vi "arc - v1.vi"() -> ()   [LabVIEW 2015]
doc: "This is the interface, the one VI which loads all the others. Run this one first.\n\n(the line below ensures settings are saved)\n[Red Tweezers Save Settings]"
uses:
  Matt Fall 2018 files/Matt working/Red Tweezers Image Processing Final 1-19/subvis/line_trapping.ctl
  Matt Fall 2018 files/Matt working/Red Tweezers Image Processing Final 1-19/subvis/spot.ctl
  <vilib>/userdefined/High Color/IMAQdx.ctl
  Matt Fall 2018 files/Matt working/Red Tweezers Image Processing Final 1-19/subvis/selection_element.ctl
  <vilib>/Analysis/Matrix/Datatypes/RealMatrix.ctl
  Matt Fall 2018 files/Matt working/Red Tweezers Image Processing Final 1-19/subvis/mouse_info.ctl
  <vilib>/Analysis/baseanly.llb/Real A x B.vi
  Matt Fall 2018 files/Matt working/Red Tweezers Image Processing Final 1-19/subvis/red_tweezers_globals_INTERNAL_VOLATILE.vi
  Matt Fall 2018 files/Matt working/Red Tweezers Image Processing Final 1-19/subvis/red_tweezers_globals.vi
  <vilib>/Analysis/Matrix/Numeric/Multiply/Multiply - RM,R.vi
  <vilib>/Analysis/NI_AALBase.lvlib
  <vilib>/vision/driver/NI_Vision_Acquisition_Software.lvlib
  <vilib>/vision/NI_Vision_Development_Module.lvlib
  <vilib>/Analysis/Matrix/NI_Matrix.lvlib
panel:
  out "Objects":T1(array[cluster]) {"Aspect Ratio" format="%.2f"; "Orientation" format="%.2f"; "Area" format="%.2f"; "Object Center"."Y" format="%.2f"; "Object Center"."X" format="%.2f"}
  out "Specific Point 2":cluster{i32, i32}
  out "Specific Point":cluster{i32, i32}
  out "bottomrx 3":dbl
  out "toply 3":dbl
  out "bottomry 3":dbl
  out "toplx 3":dbl
  out "Circles 2":T2(array[cluster]) {"Position"."Y" format="%.2f"; "Position"."X" format="%.2f"}
  out "Spot Storage":T3[](array[typedef]) {"Amplitude Correction" step=0.1; "Line Trapping"."Phase Gradient" step=0.05; "Line Trapping"."Vector"."x" step=1e-06 format="%#_6p"; "Line Trapping"."Vector"."y" step=1e-06 format="%#_6p"; "Line Trapping"."Vector"."z" step=1e-06 format="%#_6p"; "NA Position"."r" step=1e-06; "NA Position"."y" step=1e-06; "NA Position"."x" step=1e-06; "Position"."z" step=1e-06; "Position"."y" step=1e-06; "Position"."x" step=1e-06; "Phase" step=0.7753; "Intensity" step=0.1}
  out "# selected":i16
  out "Last Pattern":T3[](array[typedef]) {"Amplitude Correction" step=0.1; "Line Trapping"."Phase Gradient" step=0.05; "Line Trapping"."Vector"."x" step=1e-06 format="%#_6p"; "Line Trapping"."Vector"."y" step=1e-06 format="%#_6p"; "Line Trapping"."Vector"."z" step=1e-06 format="%#_6p"; "NA Position"."r" step=1e-06; "NA Position"."y" step=1e-06; "NA Position"."x" step=1e-06; "Position"."z" step=1e-06; "Position"."y" step=1e-06; "Position"."x" step=1e-06; "Phase" step=0.7753; "Intensity" step=0.1}
  out "Plugins":T5(array[cluster])=[{"Name"="ASI Stage", "Folder"=path "C:/Users/Richard Bowman/Dropbox/red_tweezers_1_4_rc4/plugins/ASI Stage.llb", "vi reference"=refnum, "Needs to be run"=TRUE, "Error"={"status"=FALSE, "code"=0, "source"=""}}, {"Name"="iTweezers", "Folder"=path "C:/Users/Richard Bowman/Dropbox/red_tweezers_1_4_rc4/plugins/iTweezers.llb", "vi reference"=refnum, "Needs to be run"=TRUE, "Error"={"status"=FALSE, "code"=0, "source"=""}}, {"Name"="MightexLED", "Folder"=path "C:/Users/Richard Bowman/Dropbox/red_tweezers_1_4_rc4/plugins/MightexLED.llb", "vi reference"=refnum, "Needs to be run"=TRUE, "Error"={"status"=FALSE, "code"=0, "source"=""}}]
  in  "Tab":T6(tab)
  out "Play Pressed":bool
  out "Y":dbl
  out "X":dbl
  in  "O Button":bool
  in  "OK Button":bool
  in  "Bubble Size":dbl=50.0002
  out "Hit Indicator":bool
  in  "On":bool
  out "Induce check":bool
  out "Area+ Buffer":dbl
  in  "Area to check":dbl=0.00025
  out "Prev Current Spot":dbl
  out "spots selected 2":i32=4
  out "Spot # Check":dbl
  out "Orig Y SC":dbl
  out "Orig X SC":dbl
  out "ID num check":dbl
  out "Value Check":dbl
  out "ID":dbl[](array[numeric])
  out "Null array":dbl[](array[numeric])
  out "Potential Collisions":dbl
  out "What to Check":dbl[](array[numeric])
  out "Num":dbl
  out "Old Y":dbl
  out "Old X":dbl
  out "init":dbl
  out "Looper":bool
  in  "Output to SLM":bool
  out "Maximum":dbl
  out "Projected Distance":dbl
  out "Previous Distance":dbl
  out "Group ID #":dbl
  in  "Buffer Zone":dbl=7e-05
  out "# of Spots":dbl
  out "Distance":dbl
  out "Hit":bool
  out "Y Displacement":dbl
  out "X Displacement":dbl
  out "Current Spot #":dbl
  out "spots selected":i32=4
  in  "lock aspect ratio":bool=TRUE
  in  "Size":cluster{"x":dbl, "y":dbl, "z":dbl} {"z" step=1e-06 format="%#_4p"; "y" step=1e-06 format="%#_4p"; "x" step=1e-06 format="%#_4p"}
  in  "Position":cluster{"x":dbl, "y":dbl, "z":dbl}={"x"=1e-06, "y"=-6.3e-06, "z"=0.0} {"z" step=1e-06 format="%#_4p"; "y" step=1e-06 format="%#_4p"; "x" step=1e-06 format="%#_4p"}
  in  "phase":dbl step=0.7753
  in  "Vortex Charge":i8
  in  "Intensity":dbl=1.0 step=0.1
  in  "add to selection":bool
  in  "random position":bool
  in  "new spot":bool
  in  "delete":bool
  in  "rotate":bool
  in  "Rotation Axis":u16(ring)=2 items=["Z", "X", "Y", "Custom"]
  in  "Angle (degrees)":dbl=2.0
  in  "Custom Axis":cluster{dbl, dbl, dbl}
  in  "Spot Shape":enum32{"Normal", "Line", "NA", "Mixed"}(tab)=enum."Mixed"
  in  "Line Trapping":T4 {"Phase Gradient" step=0.05; "Vector"."x" step=1e-06 format="%#_4p"; "Vector"."y" step=1e-06 format="%#_4p"; "Vector"."z" step=1e-06 format="%#_4p"}
  in  "Scale back aperture":dbl=1.1 step=0.1
  in  "Scale BA":bool
  in  "Position on back aperture":cluster{"x":dbl, "y":dbl}={"x"=-5.84327907697451e-18, "y"=0.0} {"y" step=0.1 format="%#_4p"; "x" step=0.1 format="%#_4p"}
  in  "Radius on back aperture":dbl=1.1 step=0.1
  in  "Generate":bool
  in  "Pattern":T7(tab)
  in  "Spots across centre":i32=5
  in  "Reference Array?":bool
  in  "Fraction of SLM":dbl=1.0
  in  "Spots across centre":i32=5
  in  "N":cluster{i32, i32}
  in  "spacing/m":dbl=2.0
  in  "Iterations":i32=10
  out "non-uniformity":dbl(slide)=0.031119223416512406 scale=0.0..0.2
  out "efficiency":dbl(slide)=0.8985936267644501 scale=0.0..1.0
  in  "Optimise":bool
  in  "Reset Phase/Amplitude":bool
  in  "Fall-off/m":dbl=0.00025 min=0.0 step=1e-06 format="%#_4p"
  in  "Abort Plugin":bool
  in  "Plugin:":u16(ring)=1 items=["ASI Stage", "iTweezers", "MightexLED"]
  in  "Save Video":bool
  in  "Global ROI (requires restart)":i32[](array[numeric])=[0, 0, 1280, 512]
  in  "Zoom":bool
  in  "Draw ROI":bool
  in  "Zoom to Fit":bool
  out "Image Information":string="640x480 1.93X 8-bit image 255    (0,0)"
  in  "Camera":T8
  in  "Time per Frame (ms)":dbl
  in  "Edit Sequence Mode":bool
  in  "Manual Edit":bool
  in  "Bubble ID to Empty":dbl
  in  "Clearance Button":bool
  in  "Manual Sequence":bool
  in  "Play Sequence":bool
  in  "Reset":bool
  out "Sequence Instances":dbl
  out "Counter":dbl
  in  "Save State":bool
  out "Sequence On?":bool
  in  "Sequence Order":dbl
  out "Selection/Group":T9[](array[typedef])
  in  "Sequence Storer":T3[][](array[typedef]) {"Amplitude Correction" step=0.1; "Line Trapping"."Phase Gradient" step=0.05; "Line Trapping"."Vector"."x" step=1e-06 format="%#_6p"; "Line Trapping"."Vector"."y" step=1e-06 format="%#_6p"; "Line Trapping"."Vector"."z" step=1e-06 format="%#_6p"; "NA Position"."r" step=1e-06; "NA Position"."y" step=1e-06; "NA Position"."x" step=1e-06; "Position"."z" step=1e-06; "Position"."y" step=1e-06; "Position"."x" step=1e-06; "Phase" step=0.7753; "Intensity" step=0.1}
  out "# of pairs":dbl
  out "Caging Radius":dbl
  out "Radius":dbl
  in  "New location\n ROI":bool
  out "Radius ROI x6":dbl
  out "Radius ROI y6":dbl
  out "Radius ROI y5":dbl
  out "Radius ROI x5":dbl
  out "Radius ROI y4":dbl
  out "Radius ROI x4":dbl
  out "Radius ROI y3":dbl
  out "Radius ROI x3":dbl
  out "Radius ROI x2":dbl
  out "Radius ROI y2":dbl
  out "Radius ROI y1":dbl
  out "Radius ROI x1":dbl
  out "ROI Point 1":T10
  out "ROI Point 0":T10
  out "ROI Point 2":T10
  in  "New Center Y":dbl
  in  "New Center X":dbl
  out "Delta x":dbl[](array[numeric])
  out "Delta y":dbl[](array[numeric])
  in  "Input New \nObject Location":bool
  out "Time Elapsed(ms)":i32
  out "Start":i32
  out "Stop":i32
  out "Insert End":bool
  out "NewXYRates":dbl[][](array[numeric])
  out "NewXYArraySize":dbl
  out "NewXYArray":dbl[][](array[numeric])
  in  "Rates":dbl
  out "LCS Y":dbl
  out "LCS X":dbl
  in  "LCS":dbl
  in  "Play":bool
  out "Initiate Creation":dbl
  in  "Max Number \nof Bubbles":dbl
  in  "Number of \nPlanned\nSequence Frames":dbl
  in  "Add Additional Frames":bool
  in  "Frame Location":dbl
  in  "Additional Frames Wanted":dbl
  in  "Tab Control":enum32{"Line", "Arc"}(tab)
  out "X Rate":dbl
  out "Y Rate":dbl
  out "Degree Rate":dbl
  out "Radians":dbl
  out "Center Y":dbl
  out "Center X":dbl
  in  "Radius X":dbl
  in  "Theta":dbl
  in  "Lock Current Spot":bool
  out "Locked Current Spot":dbl
  out "Numeric":dbl
  out "probe":dbl
  in  "Insert":bool
  in  "Start at Which Frame?":dbl
  out "Original Y":dbl
  out "Original X":dbl
  in  "Mark Original Position":bool
  in  "How Many Frames?":dbl
  out "New Y":dbl
  out "New X":dbl
  out "Spot Storage 2":T3[](array[typedef]) {"Amplitude Correction" step=0.1; "Line Trapping"."Phase Gradient" step=0.05; "Line Trapping"."Vector"."x" step=1e-06 format="%#_6p"; "Line Trapping"."Vector"."y" step=1e-06 format="%#_6p"; "Line Trapping"."Vector"."z" step=1e-06 format="%#_6p"; "NA Position"."r" step=1e-06; "NA Position"."y" step=1e-06; "NA Position"."x" step=1e-06; "Position"."z" step=1e-06; "Position"."y" step=1e-06; "Position"."x" step=1e-06; "Phase" step=0.7753; "Intensity" step=0.1}
  in  "Save":bool
  in  "Load":bool
  out "Object MP Y":dbl
  out "Object MP X":dbl
  out "ROI Point 3":T10
  out "Numeric 3":dbl
  out "Numeric 2":dbl
  in  "ROI points":dbl
  out "ROI Y":dbl
  out "ROI X":dbl
  out "Center Y":dbl
  out "Center X":dbl
  in  "Camera Capture 2":bool
  out "Bubble y 2":dbl
  out "Bubble x 2":dbl
  out "Number of Matches Returned":dbl
  out "bottomry 2":dbl
  out "toply 2":dbl
  out "bottomrx 2":dbl
  out "toplx 2":dbl
  in  "Send Data":bool
  out "Camera 3":T11(plugin-control)
  in  "Circle Descriptor 2":cluster{"Min Radius":dbl, "Max Radius":dbl}={"Min Radius"=3.0, "Max Radius"=500.0}
  out "Radius":dbl
  in  "Settings":T12={"Objects"=0, "Threshold"=128, "Reject Border"=FALSE, "Fill Holes"=FALSE, "Min Object Size"=FALSE, "Min Size"=3, "Max Object Size"=FALSE, "Max Size"=100, "Show Search Area"=FALSE, "Show Center"=TRUE, "Show Bounding Box"=TRUE} {"Objects" items=["Bright Objects", "Dark Objects"]; "Threshold" min=1 max=999999999 step=1; "Max Size" min=1 max=999999999 step=1; "Min Size" min=1 max=999999999 step=1}
  out "Number of Objects":i32
  in  "ROI switch":bool
  out "Video Frame Rate":dbl(knob)=50.00000000000003 scale=0.0..100.0 scale format="%.1f"
  out "Interface Frame Rate":dbl(knob)=97.23240312927678 scale=0.0..100.0 scale format="%.1f"
  in  "stop":bool=TRUE
  out "ROI new Mpy":dbl
  out "ROI new MPx":dbl
  out "ROI y6":dbl
  out "ROI x6":dbl
  out "ROI y5":dbl
  out "ROI x5":dbl
  out "ROI y4":dbl
  out "ROI x4":dbl
  out "ROI y3":dbl
  out "ROI x3":dbl
  out "ROI y2":dbl
  out "ROI x2":dbl
  out "ROI y1":dbl
  out "ROI x1":dbl
  out "ROI Point 6":T10
  out "ROI point 5":T10
  out "ROI Point 4":T10
  out "MOP pressed":bool
  out "MOP pressed After":bool
  out "X Pos every 10 sec":dbl
  out "Elapsed Time":dbl
  out "Position Indicator":string
  out "Spot Checker":T3[](array[typedef]) {"Amplitude Correction" step=0.1; "Line Trapping"."Phase Gradient" step=0.05; "Line Trapping"."Vector"."x" step=1e-06 format="%#_6p"; "Line Trapping"."Vector"."y" step=1e-06 format="%#_6p"; "Line Trapping"."Vector"."z" step=1e-06 format="%#_6p"; "NA Position"."r" step=1e-06; "NA Position"."y" step=1e-06; "NA Position"."x" step=1e-06; "Position"."z" step=1e-06; "Position"."y" step=1e-06; "Position"."x" step=1e-06; "Phase" step=0.7753; "Intensity" step=0.1}
  out "Image":T11(plugin-control)
  # "Notes:\n\nIf you are doing non-sequence controls,\nthe delete function can be used as intended.\nHowever, do not use the delete function after\nrunning a sequence! Using it will prevent\nthe bubbles from appearing as the\nnumber of spots will change, which is\nessential for the sequence to work (it would\nbe displaying the maximum number of\nbubbles). \n\nIf you happen to delete a bubble, it can be \nrestored by inserting a new spot. Once enough\nspots have been restored, click on manual edit\nto correct the # of spots tracker. It should \nbe restored to where it originally was."
  # "The SLM can be used to shape spots; here you can restrict the NA of a spot (so it comes only from part of the back aperture), or create a line-trap"
  # "The traps do not have any spot-shaping applied (so they should just be diffraction-limited focal spots)."
  # "This shapes the amplitude (and phase) of the beam to create extended line traps.  The \"Phase Gradient\" control allows the Poynting vector to push things along the line.  Unfortunately, some work is needed on the scaling factors so the phase gradient control will need tweaking if the line trap has a nonzero z component."
  # "By default,each spot comes from the whole back aperture.  Here, you can limit a spot to come from a specific part of the back aperture."
  # "The control below allows you to scale the whole back aperture (i.e. the position and size of all the apertures).  It's a one-time operation, i.e. only changes things when you push \"ok\"."
  # "A Combination of line-trapping and NA restriction has been applied to these traps.  You can get at the line trap or NA parameters on the other tabs, switching to the NA tab does not delete the line-trap settings."
  # "This tab generates Shack-Hartmann type holograms, which are often useful when aligning the system, and arrays of spots."
  # "The controls above only work when using the \"IMAQdx with ROI Buttons\" case in the bottom loop.  You can save video regardless of camera code though."
  # "Manual Edit allows a user to\ngo to a specific sequence frame."
  # "To clear the sequence, you must\nclear the array. Right click on sequence\nstorer to do this."
  # "Use this to \"clear\" a \nspecific bubble. If\nworking on a sequence,\nuse this as your delete\nbutton! You can update\nthe view by using manual edit."
  # "Use the reset button\nto clear counter.\nIt becomes necessary\nwhen you clear the array,\nespecially in manual mode."
  # "Use the sequence creator tab to specify the\nnumber of bubbles you want along with\nthe number of frames.\n\nTo save at a specific interval, the sequence\norder can be used to place the state. If used\nto correct something, it will replace the\nentire sequence frame.\n\n\"Sequence On?\" is only used in auto mode."
  # "Multiple bubbles can  be done with the\nline function. One bubble at a time for the arc\nfunction."
  # "Using the Load/Save function:\n\nRed Tweezers itself is unable to save long \nsequences, but a separate program is able to\naccomplish this. To do this, follow these\nsteps:\n\n1. After creating your sequence, press the save\nbutton below.\n\n2. Then, go to the subvi folder and find\nSequenceSaver.vi.\n\n3. At the control \"Sequence Storer,\" right-click\nthe dimensions part of the array and go to\ndata operations.\n\n4. Press \"Make Current Values Default\" and save\nthe sequence.\n\n5. The next time you load the program, simply\npress load to re-acquire the sequence. You\nwill need to insert the bubbles again, but after\nthe first frame can be recovered by using\nSequenceControl.vi."
types:
  T1 = cluster{"Object Center":cluster{"X":sgl, "Y":sgl}, "Bounding Box":cluster{"X Left":i32, "Y Top":i32, "X Right":i32, "Y Bottom":i32}, "Area":sgl, "Orientation":sgl, "Aspect Ratio":sgl, "Nb Holes":i32}[]
  T2 = cluster{"Position":cluster{"X":sgl, "Y":sgl}, "Radius":dbl, "Score":dbl}[]
  T3 = typedef "spot.ctl" = cluster{"Position":cluster{"x":dbl, "y":dbl, "z":dbl}, "Intensity":dbl, "Vortex Charge":i8, "Phase":dbl, "NA Position":cluster{"x":dbl, "y":dbl, "r":dbl}, "Line Trapping":T4, "Amplitude Correction":dbl}
  T4 = typedef "line_trapping.ctl" = cluster{"Vector":cluster{"x":dbl, "y":dbl, "z":dbl}, "Phase Gradient":dbl}
  T5 = cluster{"Name":string, "Folder":path, "vi reference":refnum<vi>, "Needs to be run":bool, "Error":errorcluster}[]
  T6 = enum32{"Current Spot", "Rotate", "Spot Shape", "Patterns", "Plugins", "Video", "Sequence", "Sequence Creator", "Spot Control", "Load/Save", "Image Process"}
  T7 = enum32{"HCP Shack-Hartmann", "Square Shack-Hartmann", "Rectangular Grid"}
  T8 = typedef "IMAQdx.ctl" = refnum<k21>
  T9 = typedef "selection_element.ctl" = cluster{"Group ID":i32, "Selected":bool}
  T10 = typedef "NI_Matrix.lvlib/RealMatrix.ctl" = dbl[][]
  T11 = typedef "IMAQ Image.ctl" = refnum<image>
  T12 = cluster{"Objects":u16, "Threshold":i32, "Reject Border":bool, "Fill Holes":bool, "Min Object Size":bool, "Min Size":i32, "Max Object Size":bool, "Max Size":i32, "Show Search Area":bool, "Show Center":bool, "Show Bounding Box":bool}
  T13 = typedef "mouse_info.ctl" = cluster{"Button Down":bool, "Dragging":bool, "Position (Image Pixels)":cluster{"X":dbl, "Y":dbl}, "Previous Position (Image Pixels)":cluster{"X":dbl, "Y":dbl}, "Button":u16, "Mods":cluster{"Double Click":bool, "Menu Key":bool}, "PlatMods":cluster{"Shift":bool, "Ctrl":bool, "Alt":bool, "Cmd":bool, "Opt":bool}}
  T14 = cluster{"Desired Font (Application)":enum16{"User-specified Font", "Application Font", "System Font", "Dialog Font"}, "[User-specified Font]":cluster{"Font Name":string, "Size":i16, "Strikeout?":bool, "Italic?":bool, "Underline?":bool, "Outline?":bool, "Shadow?":bool, "Bold?":bool, "Rotation Angle":dbl}, "Horizontal Alignment":i16, "Vertical Alignment":i16}
  T15 = cluster{"Position":cluster{"x":dbl, "y":dbl, "z":dbl}, "Intensity":dbl, "Vortex Charge":i8, "Phase":dbl, "NA Position":cluster{"x":dbl, "y":dbl, "r":dbl}, "Line Trapping":T4, "Amplitude Correction":dbl}
  T16 = enum16{"Set guide visibility", "Set grid visibility", "Show front panel", "Render on image"}
  T17 = enum32{"Current Spot", "Rotate", "Spot Shape", "Patterns", "Plugins", "Video"}
  T18 = enum16{"Left Button", "Center Button", "Right Button", "Window Close"}
  T19 = typedef "Image Type" = u32
  T20 = cluster{"number: 0 to 1":dbl, "number: 0 to 1":dbl}
  T21 = typedef "overlay_element.ctl" = cluster{"Tool":enum16{"Lines", "Oval", "Rectangle", "Text"}, "Points":cluster{"X":dbl, "Y":dbl}[], "Drawing Mode":u32, "Color":u32, "String":string}
  T22 = enum32{"Current Spot", "Rotate", "Spot Shape", "Patterns", "Plugins", "Video", "Particle Tracking", "Clamping", "Blank"}[]
  T23 = typedef "LVMenuShortCut.ctl" = cluster{"include Shift key?":bool, "include Ctrl key?":bool, "shortcut key":string}
  T24 = typedef "LVPoint32TypeDef.ctl" = cluster{"Horizontal":i32, "Vertical":i32}
  T25 = cluster{"Shift":bool, "Ctrl":bool, "Alt":bool, "Cmd":bool, "Opt":bool}
  T26 = cluster{"Button Down":bool, "Dragging":bool, "Mouse Coords (image pixels)":cluster{dbl, dbl}, "Mouse Coords (image pixels)":cluster{dbl, dbl}, "Button":u16, "Mods":cluster{"Double Click":bool, "Menu Key":bool}, "PlatMods":cluster{"Shift":bool, "Ctrl":bool, "Alt":bool, "Cmd":bool, "Opt":bool}}
  T27 = cluster{"Global Rectangle":i32[], "Contours":cluster{"Contour Type":u32, "ROI Type":u32, "Points":i32[]}[]}
  T28 = cluster{"Contour Type":u32, "ROI Type":u32, "Points":i32[]}[]
  T29 = cluster{"Position":cluster{"X":sgl, "Y":sgl}, "Radius":dbl, "Score":dbl}
  T30 = cluster{"Contour Type":u32, "ROI Type":u32, "Points":i32[]}
  T31 = cluster{"[0]":dbl, "[1]":dbl, "[2]":dbl, "[3]":dbl}
  T32 = cluster{"Object Center":cluster{"X":sgl, "Y":sgl}, "Bounding Box":cluster{"X Left":i32, "Y Top":i32, "X Right":i32, "Y Bottom":i32}, "Area":sgl, "Orientation":sgl, "Aspect Ratio":sgl, "Nb Holes":i32}
  T33 = cluster{"NewXYArray[0]":dbl, "NewXYArray[1]":dbl, "NewXYArray[2]":dbl, "NewXYArray[3]":dbl, "NewXYArray[4]":dbl, "NewXYArray[5]":dbl, "NewXYArray[6]":dbl, "NewXYArray[7]":dbl, "NewXYArray[8]":dbl}
  T34 = cluster{"Average Frame Time":dbl, "millisecond timer value":u32}
  T35 = cluster{"Position":cluster{"x":dbl, "y":dbl, "z":dbl}, "Intensity":dbl, "Vortex Charge":i8, "Phase":dbl, "NA Position":cluster{"x":dbl, "y":dbl, "r":dbl}, "Line Trapping":T4, "Amplitude Correction":dbl}[]
  T36 = enum32{"Bad", "Idle", "Run top level", "Running"}
  T37 = typedef "AviRefnum.ctl" = refnum<k1>
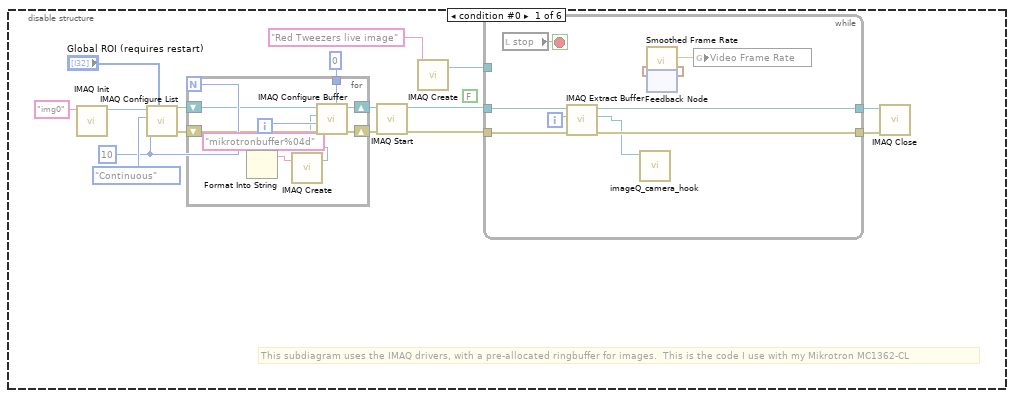
[diagram p3: hidden frame]
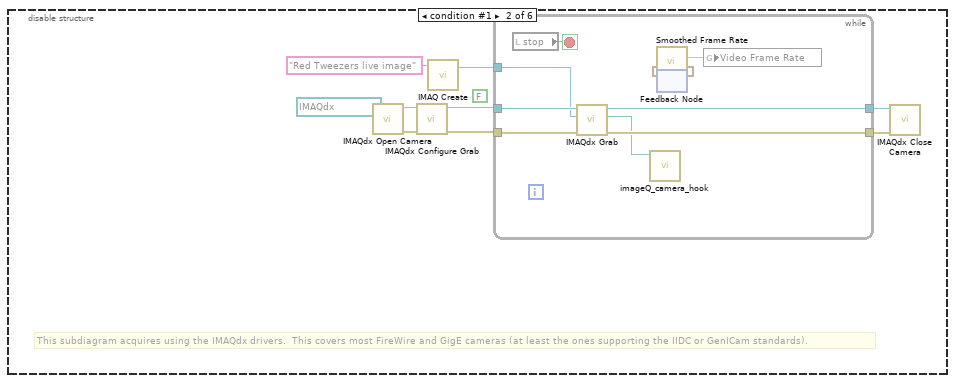
[diagram p4: hidden frame]
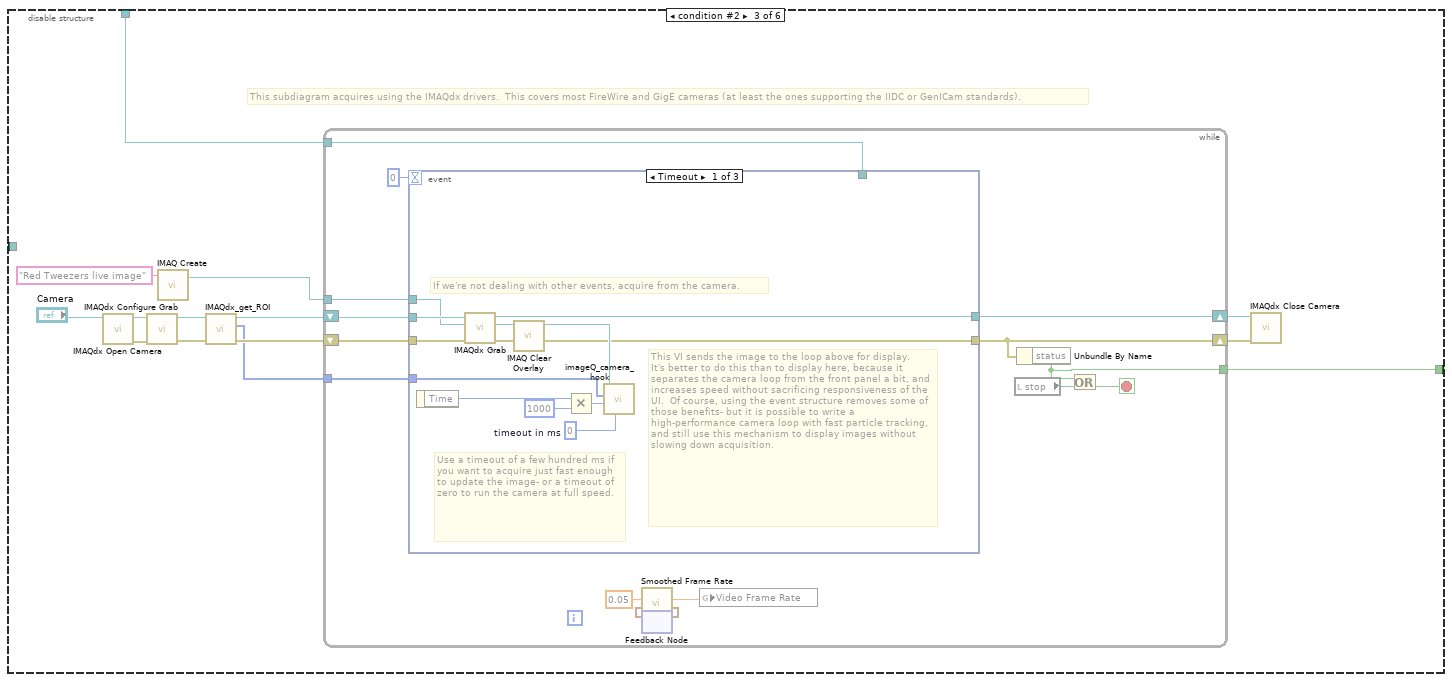
[diagram p5: hidden frame]
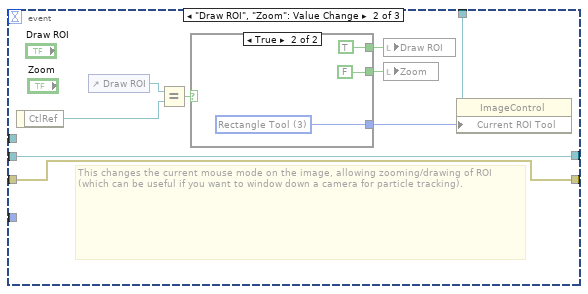
[diagram p6: hidden frame]
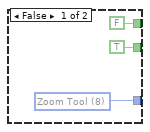
[diagram p7: hidden frame]
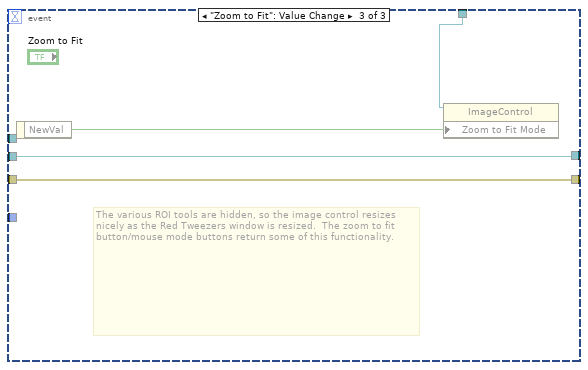
[diagram p8: hidden frame]
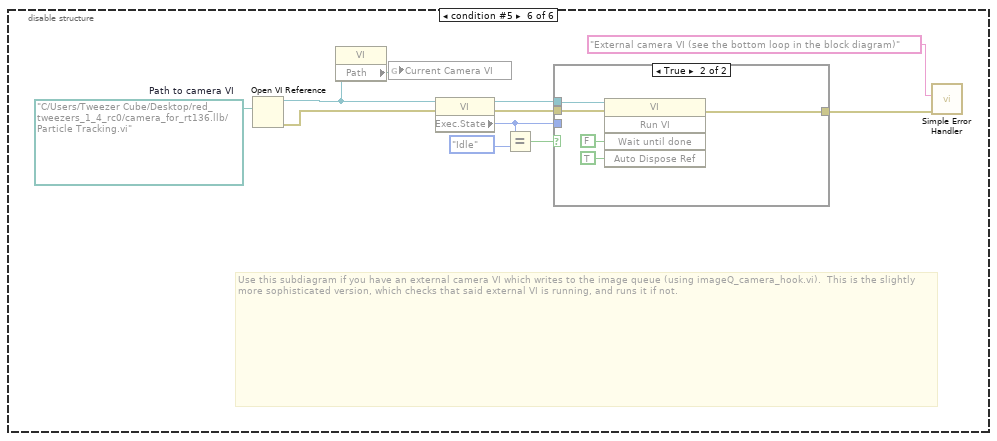
[diagram p10: hidden frame]
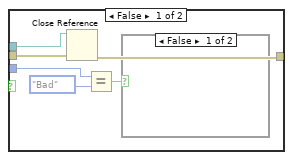
[diagram p11: hidden frame]
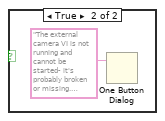
[diagram p12: hidden frame]
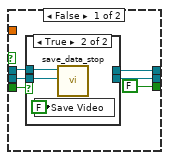
[diagram p13: hidden frame]
diagram:
  w11 = "red_tweezers_display_imageQ" ("Queue Name")
  w23 = T13 {"Button Down"=FALSE, "Dragging"=FALSE, "Position (Image Pixels)"={"X"=0.0, "Y"=0.0}, "Previous Position (Image Pixels)"={"X"=0.0, "Y"=0.0}, "Button"=0, "Mods"={"Double Click"=FALSE, "Menu Key"=FALSE}, "PlatMods"={"Shift"=FALSE, "Ctrl"=FALSE, "Alt"=FALSE, "Cmd"=FALSE, "Opt"=FALSE}}  # Mouse Information
  w24 = refnum<vi> refnum  # Image
  # "The funny looking feedback-node structure is deliberate (if odd).  We want to reload settings from the last used file (stored in the registry) only if this program has not been run since it was last loaded from file/recompiled.  That's why I use an uninitialised shift register: every time the program runs, it increments.  So, if it is zero, this is our first run (or we've been recently recompiled)."
  # "This loop handles the video that is displayed on-screen and saved to file."
  # "Initially, we only register to be told when the user clicks the image"
  # "This is the actual image control"
  # "This is a generic reference.\nIt is just a placeholder, so we can register for events later."
  # "This version of red tweezers uses two coordinate systems: \n1. Real Coordinates - corresponding to physical distances in 3D in microns\n2. Image Coordinates - position on the camera image, relative to the top left of the CURRENT ROI, measured in pixels. If the ROI changes, the relationship between \"real units\" and \"image pixels\" may change, so all values should be stored and presented to the user in REAL units unless there is a good reason to do otherwise."
  n1 = control-ref of="Plugin Pnl"() -> (w20:refnum<vi>)
  n2 = flat-sequence {
    tunnel: [w27] -> w6
    tunnel: w4 -> [_]
    frame #0 {
      n3 = vi-ref "red_tweezers_globals_INTERNAL.vi"() -> (w28:refnum<vi>)
      n4 = property class="VI"(reference=w28) -> ("Path"=w27:path)  [unwired: 1 in, 2 out]
      n5 = global write "red_tweezers_globals_INTERNAL_VOLATILE.vi" "Current Camera VI"(w27) -> ()
    }
  }
  n6 = control-ref of="Plugin:"() -> (w21:refnum<vi>)
  n7 = feedback #1() -> (w14:dbl)  [unwired: 1 in]
  n8 = Equal To 0?(x=w14) -> (x = 0?=w13:bool)
  n9 = Increment(x=w14) -> (x+1=w12:dbl)
  n10 = feedback-in #1(w12) -> ()
  n11 = call "plugins_load.vi"("Sub Panel"=w20, "Plugin Chooser"=w21) -> ("error out"=w15:errorcluster, "Plugins"=w17:T5)  [unwired: 2 in, 2 out]
  "Plugins" <- w17
  n12 = control-ref of="Image"() -> (w5:refnum<vi>)
  n13 = case shown="True" w13 {
    tunnel: w15 -> [_ w29]
    tunnel: [_ w29] -> w4
    frame False {
    }
    frame True {
      n14 = call "settings_load_default_file.vi"("error out"=w29) -> ()
    }
  }
  n15 = flat-sequence {
    tunnel: w4 -> [_]
    tunnel: w2 -> [w31]
    frame #0 {
      # "ensure we don't accidentally start saving video, and run UDP Sender to set up the hologram window."
      n16 = local write "Save Video"(FALSE ("background subtraction")) -> ()
      n17 = call "UDP Sender generic_2.vi"("Spots"=w31) -> ()  [unwired: 2 in, 1 out]
    }
  }
  n18 = global read "red_tweezers_globals.vi" "Selection/Group"() -> (w22:T9[])
  n19 = register-events(w5, w24, w24, w24) -> (reference out=w25:refnum<event-registration>)  [unwired: 2 in, 1 out]
  n20 = global read "red_tweezers_globals.vi" "Spots"() -> (w2:T3[])
  n21 = local write "stop"(FALSE ("STOP")) -> ()
  n22 = call "ensure_selection_matches_spots.vi"("Selection and Groups in"=w22, "Spots"=w2) -> ("Selection and Groups out"=w26:T9[], "Spots (duplicate)"=w1:T3[])  [unwired: 4 in]
  n23 = call "IMAQ Create"("Image Name"=w11) -> ("New Image"=w9:T11)  [unwired: 4 in, 1 out]
  n24 = call "imageQ_create_return_queue.vi"("Queue Name"=w11) -> ("queue out"=w10:refnum<queue>)
  n25 = while {
    shift-right: [w147] -> _
    shift-left: w1 -> [w167]
    shift-right: [w166] -> _
    shift-left: w26 -> [w165]
    shift-right: [w169] -> _
    shift-left: _ -> [w160]
    shift-right: [w168] -> _
    shift-left: _ -> [w159]
    tunnel: w5 -> [w164]
    shift-right: [w158] -> _
    shift-left: w23 -> [w157]
    shift-right: [w161] -> _
    shift-left: w25 -> [w162]
    border: errorcluster {"status"=FALSE, "code"=0, "source"=""} ("error out") -> [_]
    tunnel: [errorcluster {"status"=FALSE, "code"=0, "source"=""} ("error in (no error)")] -> w18
    border: w17 -> [_]
    tunnel: w1 -> [w148]
    stop <- w149 stop-if-true
    (unwired) 1 ("index")
    w64 = 7 items=["Red", "Green", "Blue", "Hue", "Saturation", "Luminance", "Value", "Intensity"] ("Color Plane")
    w67 = T19 0 items=["Grayscale (U8)", "Grayscale (I16)", "Grayscale (SGL)", "Complex (CSG)", "RGB (U32)", "HSL (U32)", "RGB (U64)", "Grayscale (U16)"] ("Image Type")
    # "When done obtatining points\nKEEP it at 7!"
    # "Cycle through to obtain points"
    # "This is the calculation for the center of the detected circle, not sure where to put for now"
    # "This Play Function inserts bubbles from a given .mat file into the sequence storer"
    # "The function inserts the newly generated sequence for the automatic sequence generator. It also contains the code\nthe code necessary to check whether the bubbles will intersect with each other in the sequence."
    # "This calculates the size of the area including the buffer zone length.\nThe bubble diameter will also be included in the near future."
    # "The statement to the right controls the area that are being chcecked and checks\nwhich bubbles need to be checked.  There are two instances where this activates\nin this case:\n\nWhen a new bubble is selected\nWhen a bubble is deselected, reverting to the last current spot #\n\nThe other case, when the bubble moves out of the area specified, is located\ninside the while loop controlling the bubble movement with a mouse."
    # "Timer function example"
    # "These functions help with the calculations for the sequence generator."
    # "This loads the sequence from the \"saver\" VI. The save function below \"saves\" the sequence into the saver VI."
    # "The VI above is SequenceSaver.vi which contains the\ncode necessary to create a sequence."
    # "This case structure is the Save State structure. This stores\nthe current state of the bubbles (ie position)."
    # "Reset sets the counter back to zero. This is particularly useful \nwhen using the manual sequence."
    # "This case structure helps to continue the sequence.\nThis takes the true case of the Sequence On? function\nor the true case for the Manual Sequence function\nin order to go to the next sequence frame."
    # "This case structure allows for the playing of the sequence.\nThe amount of time it takes to go through the sequence\ncan be edited on the current spot menu."
    # "We only write to the image overlay when we are in one of the tabs, to prevent it disappearing when we are (for example) using the mouse."
    # "These wires control saving undo info. See the VI below's tip strips for details."
    # "Setting these wires to false means:\n(1) dragging moves the selection\n(2) clicking spots changes selection\nset them to true to stop the default mouse behaviour, don't wire them straight through!"
    n26 = event shown="[6] <Image>: Mouse Move" {
      selector: w162 -> [w764 w1435 w1440 w1662 w1690 w1707 w1804 _]
      dyn-events: [w764 w1434 w1440 w1660 w1687 w1708 w1804 _] -> w161
      timeout: 0 -> [_ _ _ _ _ _ _ _]
      tunnel: [w772 _ w1442 w1657 w1692 w1699 w1791 _] -> w169
      tunnel: [w771 _ w1441 w1656 w1691 w1698 w1795 _] -> w168
      tunnel: [w770 _ _ _ _ _ _ _] -> w120
      tunnel: w167 -> [w769 w1430 w1447 w1652 w1685 w1704 w1799 w2122]
      tunnel: [w768 w1430 w1445 w1652 w1685 w1695 w1797 w2122] -> w155
      tunnel: [w767 w1429 w1444 w1641 w1684 w1705 w1787 w2121] -> w154
      tunnel: w165 -> [w766 w1429 w1446 w1641 w1684 w1703 w1798 w2121]
      tunnel: w164 -> [w765 w1431 w1437 w1651 w1688 w1706 w1800 _]
      tunnel: [w763 _ w1439 w1661 T13 {"Button Down"=FALSE, "Dragging"=FALSE, "Position (Image Pixels)"={"X"=0.0, "Y"=0.0}, "Previous Position (Image Pixels)"={"X"=0.0, "Y"=0.0}, "Button"=0, "Mods"={"Double Click"=FALSE, "Menu Key"=FALSE}, "PlatMods"={"Shift"=FALSE, "Ctrl"=FALSE, "Alt"=FALSE, "Cmd"=FALSE, "Opt"=FALSE}} T13 {"Button Down"=FALSE, "Dragging"=FALSE, "Position (Image Pixels)"={"X"=0.0, "Y"=0.0}, "Previous Position (Image Pixels)"={"X"=0.0, "Y"=0.0}, "Button"=0, "Mods"={"Double Click"=FALSE, "Menu Key"=FALSE}, "PlatMods"={"Shift"=FALSE, "Ctrl"=FALSE, "Alt"=FALSE, "Cmd"=FALSE, "Opt"=FALSE}} w1803 _] -> w158
      tunnel: w157 -> [w763 _ w1439 _ _ w1702 w1794 _]
      tunnel: w160 -> [_ _ w1442 w1657 w1692 w1699 w1791 _]
      tunnel: w159 -> [_ _ w1441 w1656 w1691 w1698 w1795 _]
      tunnel: [w762 _ _ _ _ _ _ _] -> w156
      tunnel: [_ _ w1438 _ _ _ TRUE _] -> w153
      tunnel: [_ _ _ TRUE TRUE TRUE FALSE _] -> w152
      tunnel: [TRUE _ _ _ _ _ _ _] -> w150
      tunnel: [_ _ _ _ _ _ _ "stop"] -> w149
      tunnel: w148 -> [_ _ _ _ _ _ w1788 _]
      event Timeout {
        n27 = event-data() -> ()  [unwired: 1 in, 1 out]
        n28 = case shown="\"Current Spot\", Default" "Tab" {
          tunnel: [w787 w1055 w1202 w1304 w1385 w1423] -> w768
          tunnel: w769 -> [w784 w1057 w1203 w1306 w1385 w1423]
          tunnel: w766 -> [w773 w1056 w1200 w1305 w1384 w1422]
          tunnel: [w786 w1054 w1201 w1303 w1384 w1422] -> w767
          tunnel: [w774 _ TRUE _ _ _] -> w772
          tunnel: [w774 _ _ _ _ _] -> w771
          tunnel: [_ _ _ FALSE _ _] -> w770
          tunnel: w765 -> [_ _ _ _ _ w1419]
          tunnel: w763 -> [_ _ w1182 _ _ _]
          tunnel: [_ _ w1184 _ _ _] -> w762
          frame "Current Spot", Default {
            w774 = FALSE
            # "The function below contains the code necessary to use the automatic sequence generator to create specific movements. It also helps translate cases where the point is entered in not dragged.\nThis prevents bubbles from intersecting if the bubble is told not to intersect."
            # "If it's out of date, update front panel"
            n29 = call "find_centroid.vi"("Selection and Groups"=w773, "Spots"=w784) -> ("Mean Values"=w782:T3, "size"=w776:cluster{"x":dbl, "y":dbl, "z":dbl}, "centroid"=w777:cluster{"x":dbl, "y":dbl, "z":dbl}, "# selected"=w775:i16)  [unwired: 2 in, 1 out]
            n30 = stacked-sequence {
              tunnel: w775 -> [_ w789]
              frame #0 {
                n31 = local read "spots selected"() -> (→"spots selected 2":i32)
              }
              frame #1 {
                "spots selected" <- w789
              }
            }
            n32 = feedback-in #2(w782) -> ()
            n33 = feedback #2() -> (w783:T3)  [unwired: 1 in]
            n34 = feedback #3() -> (w781:cluster{"x":dbl, "y":dbl, "z":dbl})  [unwired: 1 in]
            n35 = feedback-in #3(w776) -> ()
            n36 = Not Equal?(x=w783, y=w782) -> (x != y?=w780:bool)
            n37 = Not Equal?(x=w781, y=w776) -> (x != y?=w779:bool)
            n38 = Or(x=w780, y=w779) -> (x .or. y?=w778:bool)
            n39 = case shown="True" w778 {
              tunnel: w782 -> [_ w795]
              tunnel: w776 -> [_ w791]
              frame False {
              }
              frame True {
                n40 = Unbundle By Name(w795) -> ("Position"=w790:cluster{"x":dbl, "y":dbl, "z":dbl}, "Intensity"=w793:dbl, "Vortex Charge"=w792:i8, "Phase"=w794:dbl)
                n41 = local write "Size"(w791) -> ()
                n42 = local write "Vortex Charge"(w792) -> ()
                n43 = local write "Intensity"(w793) -> ()
                n44 = local write "Position"(w790) -> ()
                n45 = local write "phase"(w794) -> ()
                n46 = Unbundle By Name(w790) -> ()  [unwired: 2 out]
              }
            }
            n47 = local write "Selection/Group"(w773) -> ()
            n48 = event shown="[3] \"Position\": Value Change" {
              selector: _ -> [_ _ _ _ _ _ _ _]
              dyn-events: _ -> [_ _ _ _ _ _ _ _]
              timeout: 10 -> [_ _ _ _ _ _ _ _]
              tunnel: w784 -> [w797 w801 w815 w838 w942 w987 w1013 w1036]
              tunnel: w773 -> [w796 w800 w818 w845 w929 w984 w1010 w1034]
              tunnel: [w797 w799 w816 w837 w930 w985 w1011 w1035] -> w787
              tunnel: [w796 w798 w817 w845 w929 w984 w1010 w1034] -> w786
              tunnel: w777 -> [_ _ _ _ w941 _ _ _]
              event Timeout {
                n49 = event-data() -> ()  [unwired: 3 out]
              }
              event "delete": Value Change {
                n50 = event-data() -> ()  [unwired: 7 out]
                n51 = call "delete_selected_spots.vi"("Selection/Group 3"=w800, "Spots 3"=w801) -> ("Selection/Group 2"=w798:T9[], "Spots 2"=w799:T3[])  [unwired: 4 in]
              }
              event "new spot": Value Change {
                # "If we're not adding it to the selection, de-select all the other spots"
                n52 = event-data() -> ()  [unwired: 7 out]
                n53 = call "coords_ROI_currentimage.vi"() -> ("Mono ROI"=w802:i32[])
                n54 = case shown="False" "add to selection" {
                  tunnel: w818 -> [w831 w836]
                  tunnel: [w830 w836] -> w813
                  frame False {
                    n55 = for {
                      tunnel: w831 -> [w834] mode=indexing
                      tunnel: [w835] -> w830 mode=indexing
                      n56 = Unbundle(w834) -> ("Group ID"=w833:i32)  [unwired: 1 out]
                      n57 = Bundle(cluster=w834, "Group ID"=w833, "Selected"=FALSE ("Label.Visible")) -> (w835:T9)
                    }
                  }
                  frame True {
                  }
                }
                n58 = Index Array(array=w802) -> (element #1=w808:i32, element #2=w809:i32, element #3=w807:i32, element #4=w806:i32)  [unwired: 4 in]
                n59 = Bundle("Numeric"=w808, "Numeric"=w809) -> (w803:cluster{"Numeric":i32, "Numeric":i32})  [unwired: 1 in]
                n60 = Bundle("Numeric"=w807, "Numeric"=w806) -> (w805:cluster{"Numeric":i32, "Numeric":i32})  [unwired: 1 in]
                n61 = Subtract(x=w805, y=w803) -> (x-y=w804:cluster{"Numeric":i32, "Numeric":i32})
                n62 = case shown="True" "random position" {
                  tunnel: [w820 w826] -> w811
                  tunnel: w804 -> [_ w822]
                  tunnel: w803 -> [_ w821]
                  frame False {
                    n63 = call "replace_position.vi"("Position"=cluster{"x":dbl, "y":dbl, "z":dbl} {"x"=0.0, "y"=0.0, "z"=0.0}) -> ("Spot"=w820:T3)  [unwired: 1 in, 2 out]
                  }
                  frame True {
                    n64 = Random Number (0-1)() -> (number: 0 to 1=w828:dbl)
                    n65 = Random Number (0-1)() -> (number: 0 to 1=w829:dbl)
                    n66 = Bundle("number: 0 to 1"=w829, "number: 0 to 1"=w828) -> (w827:T20)  [unwired: 1 out]
                    n67 = Multiply(x=w827, y=w822) -> (x*y=w824:cluster{dbl, dbl})
                    n68 = Add(x=w824, y=w821) -> (x+y=w823:cluster{dbl, dbl})
                    n69 = call "coords_image_to_real_currentimage.vi"("Position (pixels on image)"=w823) -> ("Position (real coords)"=w825:cluster{dbl, dbl, "Z":dbl})  [unwired: 9 in]
                    n70 = call "replace_position.vi"("Position"=w825) -> ("Spot"=w826:T3)  [unwired: 1 in, 2 out]
                  }
                }
                n71 = Build Array (concatenate)(w815, w811) -> (w816:T3[])
                n72 = Build Array (concatenate)(w813, cluster{i32, "Label.Visible":bool} {0, "Label.Visible"=TRUE}) -> (w817:T9[])
              }
              event "Position": Value Change {
                # "If the position has changed, translate the spots"
                n73 = event-data() -> ("OldVal"=w843:cluster{"x":dbl, "y":dbl, "z":dbl}, "NewVal"=w844:cluster{"x":dbl, "y":dbl, "z":dbl})  [unwired: 5 out]
                n74 = flat-sequence {
                  tunnel: w845 -> [w849]
                  tunnel: w842 -> [w848]
                  tunnel: w838 -> [w847]
                  tunnel: [w846] -> w839
                  frame #0 {
                    n75 = for {
                      tunnel: w847 -> [w854] mode=indexing
                      tunnel: w849 -> [w851] mode=indexing
                      tunnel: [w853] -> w846 mode=indexing
                      tunnel: w848 -> [w852]
                      n76 = Unbundle(w851) -> ("Selected"=w850:bool)  [unwired: 1 out]
                      n77 = case shown="True" w850 {
                        tunnel: w854 -> [w855 w860]
                        tunnel: [w855 w859] -> w853
                        tunnel: w852 -> [_ w856]
                        frame False {
                        }
                        frame True {
                          n78 = call "extract_position.vi"("Spot"=w860) -> ("Position"=w857:cluster{"x":dbl, "y":dbl, "z":dbl})
                          n79 = Add(x=w857, y=w856) -> (x+y=w858:cluster{"x":dbl, "y":dbl, "z":dbl})
                          n80 = call "replace_position.vi"("Position"=w858, "Spot in"=w860) -> ("Spot"=w859:T3)  [unwired: 2 out]
                        }
                      }
                    }
                  }
                }
                n81 = Subtract(x=w844, y=w843) -> (x-y=w842:cluster{"x":dbl, "y":dbl, "z":dbl})
                n82 = local read "# of Spots"() -> (w841:dbl)
                n83 = stacked-sequence {
                  tunnel: w838 -> [_ w865 _]
                  tunnel: w839 -> [_ w864 _]
                  tunnel: w841 -> [_ w863 _]
                  tunnel: [_ _ w912] -> w840
                  tunnel: w839 -> [_ _ w911]
                  tunnel: w838 -> [_ _ w910]
                  tunnel: [_ _ w909] -> w837
                  frame #0 {
                    n84 = local write "Looper"(FALSE) -> ()
                    "init" <- 0
                  }
                  frame #1 {
                    n85 = for {
                      N: w863 -> [_]
                      tunnel: w865 -> [w870]
                      tunnel: w864 -> [w875]
                      stop <- w876 stop-if-true
                      n86 = local read "init"() -> (w869:dbl)
                      n87 = Index Array(array=w875, index=w869) -> (element=w874:T3)
                      n88 = Index Array(array=w870, index=w869) -> (element=w868:T3)
                      n89 = Unbundle By Name(w874) -> ("Position.x"=w873:dbl, "Position.y"=w872:dbl)
                      n90 = local read "# of Spots"() -> (w871:dbl)
                      n91 = Unbundle By Name(w868) -> ("Position.x"=→"Old X":dbl, "Position.y"=→"Old Y":dbl)
                      n92 = local write "New X"(w873) -> ()
                      n93 = local write "New Y"(w872) -> ()
                      n94 = stacked-sequence {
                        tunnel: w870 -> [w881 _]
                        tunnel: w873 -> [w880 _]
                        tunnel: w872 -> [w879 _]
                        tunnel: w871 -> [w878 _]
                        tunnel: w869 -> [w877 _]
                        frame #0 {
                          n95 = for {
                            N: w878 -> [_]
                            tunnel: w881 -> [w903]
                            tunnel: w880 -> [w902]
                            tunnel: w879 -> [w900]
                            tunnel: w877 -> [w885]
                            i -> [w887]
                            stop <- w886 stop-if-true
                            n96 = Index Array(array=w903, index=w887) -> (element=w904:T3)
                            n97 = Unbundle By Name(w904) -> ("Position.x"=w901:dbl, "Position.y"=w899:dbl)
                            n98 = Subtract(x=w902, y=w901) -> (x-y=w898:dbl)
                            n99 = Subtract(x=w900, y=w899) -> (x-y=w897:dbl)
                            n100 = Square(x=w898) -> (x^2=w896:dbl)
                            n101 = Square(x=w897) -> (x^2=w895:dbl)
                            n102 = local read "# of Spots"() -> (w889:dbl)
                            n103 = Add(x=w896, y=w895) -> (x+y=w894:dbl)
                            n104 = local read "Buffer Zone"() -> (w884:dbl)
                            n105 = Square Root(x=w894) -> (sqrt(x)=w893:dbl)
                            n106 = Multiply(x=2, y=w884) -> (x*y=w882:dbl)
                            n107 = Less?(x=w893, y=w882) -> (x < y?=w891:bool)
                            n108 = Not Equal?(x=w885, y=w887) -> (x != y?=w890:bool)
                            n109 = Equal?(x=w889, y=w887) -> (x = y?=w892:bool)
                            n110 = And(x=w890, y=w891) -> (x .and. y?=w888:bool)
                            "Looper" <- w888
                            n111 = Or(x=w888, y=w892) -> (x .or. y?=w886:bool)
                          }
                        }
                        frame #1 {
                          n112 = local read "Looper"() -> (w905:bool)
                          n113 = case shown="False" w905 {
                            frame False {
                              n114 = local read "init"() -> (w906:dbl)
                              n115 = Add(x=w906, y=1) -> (x+y=w908:dbl)
                              n116 = local write "init"(w908) -> ()
                            }
                            frame True {
                            }
                          }
                        }
                      }
                      n117 = local read "Looper"() -> (w876:bool)
                    }
                  }
                  frame #2 {
                    n118 = local read "Looper"() -> (w913:bool)
                    n119 = case shown="True" w913 {
                      tunnel: w911 -> [w917 _]
                      tunnel: w910 -> [_ w925]
                      tunnel: ["This is an acceptable entry." "ERROR: A bubble will intersect the buffer zone."] -> w912
                      tunnel: [w917 w925] -> w909
                      frame False {
                        n120 = local write "Looper"(FALSE) -> ()
                        n121 = local read "Current Spot #"() -> (w918:dbl)
                        n122 = Index Array(array=w917, index=w918) -> (element=w916:T3)
                        n123 = Unbundle By Name(w916) -> ("Position.x"=w915:dbl, "Position.y"=w914:dbl)
                        n124 = local write "New Y"(w914) -> ()
                        n125 = local write "New X"(w915) -> ()
                      }
                      frame True {
                        # "Restore original position"
                        n126 = local write "Looper"(FALSE) -> ()
                        n127 = local read "Old Y"() -> (w922:dbl)
                        n128 = local read "Old X"() -> (w923:dbl)
                        n129 = local read "Position"() -> (w921:cluster{"x":dbl, "y":dbl, "z":dbl})
                        n130 = Bundle By Name(cluster=w921, "x"=w923, "y"=w922) -> (w924:cluster{"x":dbl, "y":dbl, "z":dbl})
                        n131 = local write "Position"(w924) -> ()
                      }
                    }
                  }
                }
                "Position Indicator" <- w840
              }
              event "Size": Value Change {
                # "If we were constraining the aspect ratio, or preventing a divide by zero, the size control on the FP may be incorrect.  We refresh it in here to stop it displaying a wrong value."
                # "If the size has changed, scale the spots"
                n132 = event-data() -> ("OldVal"=w934:cluster{"x":dbl, "y":dbl, "z":dbl}, "NewVal"=w940:cluster{"x":dbl, "y":dbl, "z":dbl})  [unwired: 5 out]
                n133 = Not Equal?(x=w934, y=w940) -> (x != y?=w933:cluster{"x":bool, "y":bool, "z":bool})
                n134 = Divide(x=w940, y=w934) -> (x/y=w939:cluster{"x":dbl, "y":dbl, "z":dbl})
                n135 = Not Equal To 0?(x=w934) -> (x != 0?=w932:cluster{"x":bool, "y":bool, "z":bool})
                n136 = And(x=w933, y=w932) -> (x .and. y?=w931:cluster{"x":bool, "y":bool, "z":bool})
                n137 = Cluster To Array(cluster=w931) -> (array=w938:bool[])
                n138 = Cluster To Array(cluster=w939) -> (array=w937:dbl[])
                n139 = case shown="True" "lock aspect ratio" {
                  tunnel: w938 -> [w946 w963]
                  tunnel: w937 -> [w945 w961]
                  tunnel: [w943 w953] -> w936
                  frame False {
                    # "We are not constraining the aspect ratio here, so just check we're not introducing NAs"
                    n140 = for {
                      tunnel: w946 -> [w952] mode=indexing
                      tunnel: w945 -> [w948] mode=indexing
                      tunnel: [w950] -> w944 mode=indexing
                      n141 = Not A Number/Path/Refnum?(number/path/refnum=w948) -> (NaN/Path/Refnum?=w949:bool)
                      n142 = Compound Arithmetic op=AND(w952, invert w949) -> (w951:bool)
                      n143 = Select(t=w948, s=w951, f=1.0) -> (s? t:f=w950:dbl)
                    }
                    n144 = Array To Cluster(array=w944) -> (cluster=w943:cluster{"[0]":dbl, "[1]":dbl, "[2]":dbl})
                  }
                  frame True {
                    # "Pick the first element that changed and use it.  Also need to make sure (1) an element did change and (2) everything's valid (no divide by zeros)"
                    n145 = Search 1D Array(1D array=w963, element=TRUE) -> (index of element=w960:i32)  [unwired: 1 in]
                    n146 = Index Array(array=w961, index=w960) -> (element=w956:dbl)
                    n147 = Not A Number/Path/Refnum?(number/path/refnum=w956) -> (NaN/Path/Refnum?=w959:bool)
                    n148 = Less Than 0?(x=w960) -> (x < 0?=w958:bool)
                    n149 = Or(x=w959, y=w958) -> (x .or. y?=w957:bool)
                    n150 = Select(t=1.0, s=w957, f=w956) -> (s? t:f=w954:dbl)
                    n151 = Bundle("x"=w954, "x"=w954, "x"=w954) -> (w953:cluster{"x":dbl, "x":dbl, "x":dbl})  [unwired: 1 in]
                  }
                }
                n152 = for {
                  tunnel: w942 -> [w969] mode=indexing
                  tunnel: w929 -> [w966] mode=indexing
                  tunnel: [w968] -> w930 mode=indexing
                  tunnel: w936 -> [w967]
                  tunnel: w941 -> [w964]
                  n153 = Unbundle(w966) -> ("Selected"=w965:bool)  [unwired: 1 out]
                  n154 = case shown="True" w965 {
                    tunnel: w969 -> [w970 w978]
                    tunnel: [w970 w977] -> w968
                    tunnel: w967 -> [_ w976]
                    tunnel: w964 -> [_ w972]
                    frame False {
                    }
                    frame True {
                      n155 = call "extract_position.vi"("Spot"=w978) -> ("Position"=w974:cluster{"x":dbl, "y":dbl, "z":dbl})
                      n156 = Subtract(x=w974, y=w972) -> (x-y=w975:cluster{"x":dbl, "y":dbl, "z":dbl})
                      n157 = Multiply(x=w975, y=w976) -> (x*y=w973:cluster{"x":dbl, dbl, dbl})
                      n158 = Add(x=w972, y=w973) -> (x+y=w971:cluster{"x":dbl, dbl, dbl})
                      n159 = call "replace_position.vi"("Position"=w971, "Spot in"=w978) -> ("Spot"=w977:T3)  [unwired: 2 out]
                    }
                  }
                }
                n160 = call "find_centroid.vi"("Selection and Groups"=w929, "Spots"=w930) -> ("size"=w928:cluster{"x":dbl, "y":dbl, "z":dbl})  [unwired: 2 in, 4 out]
                n161 = local write "Size"(w928) -> ()
              }
              event "Intensity": Value Change {
                # "When  the user changes intensity, scale all the spots selected so the new mean is correct but keep the ratio between the selected spots.\n\nThe exception to this is when the mean intensity is zero, in which case multiplying makes no sense- in that case we just replace with the new value."
                n162 = event-data() -> ("NewVal"=w979:dbl, "OldVal"=w986:dbl)  [unwired: 5 out]
                n163 = Equal To 0?(x=w986) -> (x = 0?=w982:bool)
                n164 = Not A Number/Path/Refnum?(number/path/refnum=w986) -> (NaN/Path/Refnum?=w981:bool)
                n165 = Or(x=w982, y=w981) -> (x .or. y?=w980:bool)
                n166 = Divide(x=w979, y=w986) -> (x/y=w983:dbl)
                n167 = for {
                  tunnel: w987 -> [w992] mode=indexing
                  tunnel: w984 -> [w994] mode=indexing
                  tunnel: [w991] -> w985 mode=indexing
                  tunnel: w983 -> [w990]
                  tunnel: w980 -> [w989]
                  tunnel: w979 -> [w988]
                  n168 = Unbundle(w994) -> ("Selected"=w993:bool)  [unwired: 1 out]
                  n169 = case shown="True" w993 {
                    tunnel: w992 -> [w995 w1002]
                    tunnel: [w995 w999] -> w991
                    tunnel: w990 -> [_ w998]
                    tunnel: w989 -> [_ w997]
                    tunnel: w988 -> [_ w996]
                    frame False {
                    }
                    frame True {
                      n170 = Unbundle By Name(w1002) -> ("Intensity"=w1000:dbl)
                      n171 = case shown="True" w997 {
                        tunnel: [w1005 w1006] -> w1001
                        tunnel: w1000 -> [w1004 _]
                        tunnel: w998 -> [w1003 _]
                        tunnel: w996 -> [_ w1006]
                        frame False {
                          n172 = Multiply(x=w1004, y=w1003) -> (x*y=w1005:dbl)
                        }
                        frame True {
                        }
                      }
                      n173 = Bundle By Name(cluster=w1002, "Intensity"=w1001) -> (w999:T3)
                    }
                  }
                }
              }
              event "phase": Value Change {
                # "When  the user changes phase, translate the phase of all spots selectedd"
                n174 = event-data() -> ("NewVal"=w1008:dbl, "OldVal"=w1012:dbl)  [unwired: 5 out]
                n175 = Not A Number/Path/Refnum?(number/path/refnum=w1012) -> (NaN/Path/Refnum?=w1007:bool)
                n176 = Subtract(x=w1008, y=w1012) -> (x-y=w1009:dbl)
                n177 = for {
                  tunnel: w1013 -> [w1018] mode=indexing
                  tunnel: w1010 -> [w1020] mode=indexing
                  tunnel: [w1017] -> w1011 mode=indexing
                  tunnel: w1009 -> [w1016]
                  tunnel: w1007 -> [w1015]
                  tunnel: w1008 -> [w1014]
                  n178 = Unbundle(w1020) -> ("Selected"=w1019:bool)  [unwired: 1 out]
                  n179 = case shown="False" w1019 {
                    tunnel: w1018 -> [w1021 w1028]
                    tunnel: [w1021 w1025] -> w1017
                    tunnel: w1016 -> [_ w1024]
                    tunnel: w1015 -> [_ w1023]
                    tunnel: w1014 -> [_ w1022]
                    frame False {
                    }
                    frame True {
                      n180 = Unbundle By Name(w1028) -> ("Phase"=w1026:dbl)
                      n181 = case shown="False" w1023 {
                        tunnel: [w1031 w1032] -> w1027
                        tunnel: w1026 -> [w1030 _]
                        tunnel: w1024 -> [w1029 _]
                        tunnel: w1022 -> [_ w1032]
                        frame False {
                          n182 = Add(x=w1030, y=w1029) -> (x+y=w1031:dbl)
                        }
                        frame True {
                        }
                      }
                      n183 = Bundle By Name(cluster=w1028, "Phase"=w1027) -> (w1025:T3)
                    }
                  }
                }
              }
              event "Vortex Charge": Value Change {
                # "When  the user changes l, just set all selected spots to have that value of l."
                n184 = event-data() -> ("NewVal"=w1033:i8)  [unwired: 6 out]
                n185 = for {
                  tunnel: w1036 -> [w1039] mode=indexing
                  tunnel: w1034 -> [w1041] mode=indexing
                  tunnel: [w1038] -> w1035 mode=indexing
                  tunnel: w1033 -> [w1037]
                  n186 = Unbundle(w1041) -> ("Selected"=w1040:bool)  [unwired: 1 out]
                  n187 = case shown="True" w1040 {
                    tunnel: w1039 -> [w1042 w1045]
                    tunnel: [w1042 w1044] -> w1038
                    tunnel: w1037 -> [_ w1043]
                    frame False {
                    }
                    frame True {
                      n188 = Bundle By Name(cluster=w1045, "Vortex Charge"=w1043) -> (w1044:T3)
                    }
                  }
                }
              }
            }
          }
          frame "Spot Shape" {
            # "We update the spot shape tab only when spots have changed OUTSIDE this tab.  This avoids unnecessary jumping about of the tab control."
            n189 = call "find_centroid.vi"("Selection and Groups"=w1056, "Spots"=w1057) -> ("Mean Values"=w1052:T3)  [unwired: 2 in, 4 out]
            n190 = Wait (ms)(milliseconds to wait=u32 10) -> ()  [unwired: 1 out]
            n191 = call "spots_shape.vi"("Selection and Groups"=w1056, "Spots"=w1057) -> ("Spot Shape"=w1059:enum32{"Normal", "Line", "NA", "Mixed"})  [unwired: 7 in]
            n192 = feedback-in #4(w1052) -> ()
            n193 = feedback #4() -> (w1053:T3)  [unwired: 1 in]
            n194 = Not Equal?(x=w1053, y=w1052) -> (x != y?=w1058:bool)
            n195 = feedback #5() -> (w1048:enum32{"Normal", "Line", "NA", "Mixed"})  [unwired: 1 in]
            n196 = feedback #6() -> (w1050:T3)  [unwired: 1 in]
            n197 = Not Equal?(x=w1050, y=w1052) -> (x != y?=w1049:bool)
            n198 = case shown="False" w1049 {
              tunnel: w1059 -> [_ w1178]
              tunnel: ["Spot Shape" w1178] -> w1047
              frame False {
              }
              frame True {
                n199 = local write "Spot Shape"(w1178) -> ()
              }
            }
            n200 = feedback-in #5(w1047) -> ()
            n201 = Not Equal?(x=w1047, y=w1048) -> (x != y?=w1046:bool)
            n202 = case shown="\"Normal\", Default" w1047 {
              tunnel: w1057 -> [w1063 w1080 w1106 w1176]
              tunnel: w1056 -> [w1062 w1079 w1105 w1175]
              tunnel: [w1062 w1078 w1103 w1175] -> w1054
              tunnel: [w1061 w1077 w1104 w1176] -> w1055
              tunnel: w1052 -> [_ w1076 w1102 _]
              tunnel: w1058 -> [_ w1075 w1101 _]
              tunnel: w1046 -> [_ w1073 w1099 _]
              frame "Normal", Default {
                # "If \"normal\" is selected, don't allow any NA or line-trapping stuff"
                n203 = for {
                  tunnel: w1063 -> [w1066] mode=indexing
                  tunnel: w1062 -> [w1065] mode=indexing
                  tunnel: [w1067] -> w1061 mode=indexing
                  n204 = Unbundle(w1065) -> ("Selected"=w1064:bool)  [unwired: 1 out]
                  n205 = case shown="True" w1064 {
                    tunnel: [w1068 w1072] -> w1067
                    tunnel: w1066 -> [w1068 w1071]
                    frame False {
                    }
                    frame True {
                      n206 = Bundle By Name(cluster=w1071, "NA Position"=cluster{"x":dbl, "y":dbl, "r":dbl} {"x"=0.0, "y"=0.0, "r"=1.0} ("x"), "Line Trapping"=T4 {"Vector"={"x"=0.0, "y"=0.0, "z"=0.0}, "Phase Gradient"=0.0}) -> (w1072:T3)
                    }
                  }
                }
              }
              frame "Line" {
                # "If it's out of date, update front panel"
                n207 = Or(x=w1075, y=w1073) -> (x .or. y?=w1074:bool)
                n208 = case shown="True" w1074 {
                  tunnel: w1076 -> [_ w1083]
                  frame False {
                  }
                  frame True {
                    n209 = Unbundle By Name(w1083) -> ("Line Trapping"=w1082:T4)
                    n210 = local write "Line Trapping"(w1082) -> ()
                  }
                }
                n211 = event shown="[1] \"Line Trapping\": Value Change" {
                  selector: _ -> [_ _]
                  dyn-events: _ -> [_ _]
                  timeout: 10 -> [_ _]
                  tunnel: w1080 -> [w1085 w1089]
                  tunnel: w1079 -> [w1084 w1087]
                  tunnel: [w1085 w1088] -> w1077
                  tunnel: [w1084 w1087] -> w1078
                  event Timeout {
                    n212 = event-data() -> ()  [unwired: 3 out]
                  }
                  event Value Change {
                    # "If the line vector has changed, update it"
                    n213 = event-data() -> ("NewVal"=w1086:T4)  [unwired: 6 out]
                    n214 = for {
                      tunnel: w1089 -> [w1094] mode=indexing
                      tunnel: w1087 -> [w1091] mode=indexing
                      tunnel: [w1093] -> w1088 mode=indexing
                      tunnel: w1086 -> [w1092]
                      n215 = Unbundle(w1091) -> ("Selected"=w1090:bool)  [unwired: 1 out]
                      n216 = case shown="True" w1090 {
                        tunnel: w1094 -> [w1095 w1097]
                        tunnel: [w1095 w1098] -> w1093
                        tunnel: w1092 -> [_ w1096]
                        frame False {
                        }
                        frame True {
                          n217 = Bundle By Name(cluster=w1097, "Line Trapping"=w1096) -> (w1098:T3)
                        }
                      }
                    }
                  }
                }
              }
              frame "NA" {
                n218 = Or(x=w1099, y=w1101) -> (x .or. y?=w1100:bool)
                n219 = case shown="True" w1100 {
                  tunnel: w1102 -> [_ w1111]
                  frame False {
                  }
                  frame True {
                    n220 = Unbundle By Name(w1111) -> ("NA Position"=w1110:cluster{"x":dbl, "y":dbl, "r":dbl})
                    n221 = call "xyz_to_xy.vi"("Position"=w1110) -> ("Position (2D)"=w1109:cluster{"x":dbl, "y":dbl}, "z"=w1108:dbl)  [unwired: 6 out]
                    n222 = local write "Position on back aperture"(w1109) -> ()
                    n223 = local write "Radius on back aperture"(w1108) -> ()
                  }
                }
                n224 = event shown="[3] \"Scale BA\": Value Change" {
                  selector: _ -> [_ _ _ _]
                  dyn-events: _ -> [_ _ _ _]
                  timeout: 10 -> [_ _ _ _]
                  tunnel: w1106 -> [w1113 w1119 w1140 w1162]
                  tunnel: w1105 -> [w1112 w1117 w1137 w1163]
                  tunnel: [w1113 w1118 w1138 w1160] -> w1104
                  tunnel: [w1112 w1117 w1137 w1163] -> w1103
                  event Timeout {
                    n225 = event-data() -> ()  [unwired: 3 out]
                  }
                  event "Position on back aperture": Value Change {
                    # "If the position has changed, translate the spots"
                    n226 = event-data() -> ("OldVal"=w1115:cluster{"x":dbl, "y":dbl}, "NewVal"=w1116:cluster{"x":dbl, "y":dbl})  [unwired: 5 out]
                    n227 = Subtract(x=w1116, y=w1115) -> (x-y=w1114:cluster{"x":dbl, "y":dbl})
                    n228 = for {
                      tunnel: w1119 -> [w1124] mode=indexing
                      tunnel: w1117 -> [w1121] mode=indexing
                      tunnel: [w1123] -> w1118 mode=indexing
                      tunnel: w1114 -> [w1122]
                      n229 = Unbundle(w1121) -> ("Selected"=w1120:bool)  [unwired: 1 out]
                      n230 = case shown="True" w1120 {
                        tunnel: w1124 -> [w1125 w1127]
                        tunnel: [w1125 w1128] -> w1123
                        tunnel: w1122 -> [_ w1129]
                        frame False {
                        }
                        frame True {
                          n231 = Unbundle By Name(w1127) -> ("NA Position"=w1131:cluster{"x":dbl, "y":dbl, "r":dbl})
                          n232 = call "xy_to_xyz.vi"("Position (2D)"=w1129) -> ("Position (3D)"=w1130:cluster{dbl, dbl, dbl})  [unwired: 1 in, 2 out]
                          n233 = Add(x=w1131, y=w1130) -> (x+y=w1126:cluster{dbl, dbl, dbl})
                          n234 = Bundle By Name(cluster=w1127, "NA Position"=w1126) -> (w1128:T3)
                        }
                      }
                    }
                  }
                  event "Radius on back aperture": Value Change {
                    # "When  the user changes intensity, scale all the spots selected so the new mean is correct but keep the ratio between the selected spots.\n\nThe exception to this is when the mean intensity is zero, in which case multiplying makes no sense- in that case we just replace with the new value."
                    n235 = event-data() -> ("NewVal"=w1132:dbl, "OldVal"=w1139:dbl)  [unwired: 5 out]
                    n236 = Equal To 0?(x=w1139) -> (x = 0?=w1135:bool)
                    n237 = Not A Number/Path/Refnum?(number/path/refnum=w1139) -> (NaN/Path/Refnum?=w1134:bool)
                    n238 = Or(x=w1135, y=w1134) -> (x .or. y?=w1133:bool)
                    n239 = Divide(x=w1132, y=w1139) -> (x/y=w1136:dbl)
                    n240 = for {
                      tunnel: w1140 -> [w1145] mode=indexing
                      tunnel: w1137 -> [w1147] mode=indexing
                      tunnel: [w1144] -> w1138 mode=indexing
                      tunnel: w1136 -> [w1143]
                      tunnel: w1133 -> [w1142]
                      tunnel: w1132 -> [w1141]
                      n241 = Unbundle(w1147) -> ("Selected"=w1146:bool)  [unwired: 1 out]
                      n242 = case shown="True" w1146 {
                        tunnel: w1145 -> [w1148 w1155]
                        tunnel: [w1148 w1152] -> w1144
                        tunnel: w1143 -> [_ w1151]
                        tunnel: w1142 -> [_ w1150]
                        tunnel: w1141 -> [_ w1149]
                        frame False {
                        }
                        frame True {
                          n243 = Unbundle By Name(w1155) -> ("NA Position.r"=w1153:dbl)
                          n244 = case shown="False" w1150 {
                            tunnel: [w1158 w1159] -> w1154
                            tunnel: w1153 -> [w1157 _]
                            tunnel: w1151 -> [w1156 _]
                            tunnel: w1149 -> [_ w1159]
                            frame False {
                              n245 = Multiply(x=w1157, y=w1156) -> (x*y=w1158:dbl)
                            }
                            frame True {
                            }
                          }
                          n246 = Bundle By Name(cluster=w1155, "NA Position.r"=w1154) -> (w1152:T3)
                        }
                      }
                    }
                  }
                  event "Scale BA": Value Change {
                    n247 = event-data() -> ()  [unwired: 7 out]
                    n248 = for {
                      tunnel: w1163 -> [w1168] mode=indexing
                      tunnel: w1162 -> [w1166] mode=indexing
                      tunnel: "Scale back aperture" -> [w1165]
                      tunnel: [w1164] -> w1160 mode=indexing
                      n249 = Unbundle(w1168) -> ("Selected"=w1167:bool)  [unwired: 1 out]
                      n250 = case shown="True" w1167 {
                        tunnel: w1166 -> [w1169 w1170]
                        tunnel: w1165 -> [_ w1173]
                        tunnel: [w1169 w1171] -> w1164
                        frame False {
                        }
                        frame True {
                          n251 = Unbundle By Name(w1170) -> ("NA Position"=w1174:cluster{"x":dbl, "y":dbl, "r":dbl})
                          n252 = Multiply(x=w1173, y=w1174) -> (x*y=w1172:cluster{"x":dbl, "y":dbl, "r":dbl})
                          n253 = Bundle By Name(cluster=w1170, "NA Position"=w1172) -> (w1171:T3)
                        }
                      }
                    }
                  }
                }
              }
              frame "Mixed" {
              }
            }
            n254 = call "find_centroid.vi"("Selection and Groups"=w1054, "Spots"=w1055) -> ("Mean Values"=w1051:T3)  [unwired: 2 in, 4 out]
            n255 = feedback-in #6(w1051) -> ()
          }
          frame "Rotate" {
            w1189 = u32 0 items=["Frame", "Fill", "Highlight"] ("Drawing Mode")
            w1188 = u32 0 ("Color")
            w1185 = i16 100 ("radius")
            # "It's necessary to check this has changed to stop us unintentionally \"spinning\" the spots..."
            # "Draw the centroid as a spot, then a large circle+cross"
            # "It's important that this loop doesn't go too fast- it hogs the CPU.  However, each tab can have a different loop speed."
            n256 = Unbundle By Name(w1182) -> ("Position (Image Pixels)"=w1198:cluster{"X":dbl, "Y":dbl}, "Previous Position (Image Pixels)"=w1197:cluster{"X":dbl, "Y":dbl}, "Dragging"=w1199:bool)
            n257 = feedback-in #7(w1182) -> ()
            n258 = feedback #7() -> (w1183:T13)  [unwired: 1 in]
            n259 = call "find_centroid.vi"("Selection and Groups"=w1200, "Spots"=w1203) -> ("centroid"=w1196:cluster{"x":dbl, "y":dbl, "z":dbl})  [unwired: 2 in, 4 out]
            n260 = Not Equal?(x=w1182, y=w1183) -> (x != y?=w1180:bool)
            n261 = Wait (ms)(milliseconds to wait=u32 10) -> ()  [unwired: 1 out]
            n262 = And(x=w1180, y=w1199) -> (x .and. y?=w1181:bool)
            n263 = call "coords_real_to_image_currentview.vi"("Position (real coords)"=w1196) -> ("Position (pixels, relative to the top left of the image)"=w1179:cluster{dbl, dbl})  [unwired: 7 in, 1 out]
            n264 = case shown="True" w1181 {
              tunnel: w1203 -> [w1212 w1256]
              tunnel: [w1214 w1255] -> w1202
              tunnel: w1200 -> [w1213 w1257]
              tunnel: [w1213 w1257] -> w1201
              tunnel: w1196 -> [w1211 w1248]
              tunnel: w1198 -> [_ w1247]
              tunnel: w1197 -> [_ w1246]
              tunnel: w1179 -> [_ w1245]
              frame False {
                n265 = event shown="[1] Timeout" {
                  selector: _ -> [_ _]
                  dyn-events: _ -> [_ _]
                  timeout: 10 -> [_ _]
                  tunnel: [w1227 w1244] -> w1214
                  tunnel: w1213 -> [w1226 _]
                  tunnel: w1212 -> [w1225 w1244]
                  tunnel: w1211 -> [w1221 _]
                  event "rotate": Value Change {
                    n266 = event-data() -> ()  [unwired: 6 out]
                    n267 = case shown="3" "Rotation Axis" {
                      tunnel: [cluster{dbl, dbl, dbl} {0.0, 0.0, 1.0} ("Custom Axis") cluster{dbl, dbl, dbl} {1.0, 0.0, 0.0} ("Custom Axis") cluster{dbl, dbl, dbl} {0.0, 1.0, 0.0} ("Custom Axis") "Custom Axis"] -> w1222
                      frame 0, Default {
                        # "Z"
                      }
                      frame 1 {
                        # "X"
                      }
                      frame 2 {
                        # "Y"
                      }
                      frame 3 {
                      }
                    }
                    n268 = call "normalise_3d_vector.vi"("Vector"=w1222) -> ("Unit Vector"=w1224:cluster{dbl, dbl, dbl})  [unwired: 3 out]
                    n269 = Divide(x=6.283185307179586, y=360.0) -> (x/y=w1219:dbl)
                    n270 = Multiply(x="Angle (degrees)", y=w1219) -> (x*y=w1216:dbl)
                    n271 = call "arb_rotation_matrix.vi"("Unit Vector"=w1224, "theta"=w1216) -> ("Real Matrix"=w1228:T10)
                    n272 = for {
                      tunnel: w1226 -> [w1238] mode=indexing
                      tunnel: w1225 -> [w1233] mode=indexing
                      tunnel: [w1234] -> w1227 mode=indexing
                      tunnel: w1221 -> [w1236]
                      tunnel: w1228 -> [w1235]
                      n273 = Unbundle(w1238) -> ("Selected"=w1237:bool)  [unwired: 1 out]
                      n274 = case shown="True" w1237 {
                        tunnel: w1236 -> [_ w1243]
                        tunnel: [w1239 w1242] -> w1234
                        tunnel: w1233 -> [w1239 w1241]
                        tunnel: w1235 -> [_ w1240]
                        frame False {
                        }
                        frame True {
                          n275 = call "apply_matrix_transformation_to_spots.vi"("Transform centre (i.e. transform about this point)"=w1243, "Transformation Matrix (3x3)"=w1240, "Spot In"=w1241) -> ("Spot Out"=w1242:T3)  [unwired: 5 out]
                        }
                      }
                    }
                  }
                  event Timeout {
                    n276 = event-data() -> ()  [unwired: 4 out]
                  }
                }
              }
              frame True {
                # "if the mouse has not moved, stuff will be NaN, so let's make like a leopard and not change our spots"
                # "the magnitude of the change in our direction vector gives the rotation angle in radians"
                # "If it's within 100px of the centroid, pretend the mouse is on the surface of a sphere, and synthesize Z accordingly (z^2=100^2-x^2-y^2).  This allows rotation in 3d :)  The output should always be a unit vector."
                n277 = Build Array(w1247, w1246) -> (w1262:cluster{"X":dbl, "Y":dbl}[])
                n278 = for {
                  tunnel: w1245 -> [w1295]
                  tunnel: w1262 -> [w1291] mode=indexing
                  tunnel: [w1281] -> w1261 mode=indexing
                  n279 = Subtract(x=w1291, y=w1295) -> (x-y=w1286:cluster{dbl, dbl})
                  n280 = Divide(x=w1286, y=100.0 ("x")) -> (x/y=w1287:cluster{dbl, dbl})
                  n281 = Square(x=w1287) -> (x^2=w1294:cluster{dbl, dbl})
                  n282 = Unbundle(w1294) -> (w1292:dbl, w1293:dbl)
                  n283 = Add(x=w1292, y=w1293) -> (x+y=w1283:dbl)
                  n284 = Subtract(x=1.0, y=w1283) -> (x-y=w1289:dbl)
                  n285 = Square Root(x=w1283) -> (sqrt(x)=w1284:dbl)
                  n286 = Greater Than 0?(x=w1289) -> (x > 0?=w1290:bool)
                  n287 = case shown="False" w1290 {
                    tunnel: w1289 -> [_ w1302]
                    tunnel: [0.0 w1301] -> w1280
                    tunnel: w1287 -> [w1299 w1300]
                    tunnel: w1284 -> [w1298 _]
                    tunnel: [w1297 w1300] -> w1282
                    frame False {
                      n288 = Divide(x=w1299, y=w1298) -> (x/y=w1297:cluster{dbl, dbl})
                    }
                    frame True {
                      n289 = Square Root(x=w1302) -> (sqrt(x)=w1301:dbl)
                    }
                  }
                  n290 = call "xy_to_xyz.vi"("z"=w1280, "Position (2D)"=w1282) -> ("Position (3D)"=w1281:cluster{dbl, dbl, dbl})  [unwired: 2 out]
                }
                n291 = Index Array(array=w1261) -> (element #1=w1260:cluster{dbl, dbl, dbl}, element #2=w1251:cluster{dbl, dbl, dbl})  [unwired: 2 in]
                n292 = Add(x=w1260, y=w1251) -> (x+y=w1250:cluster{dbl, dbl, dbl})
                n293 = Subtract(x=w1260, y=w1251) -> (x-y=w1249:cluster{dbl, dbl, dbl})
                n294 = call "cross_product.vi"("b"=w1250, "a"=w1249) -> ("a cross b"=w1259:cluster{dbl, dbl, dbl})
                n295 = call "normalise_3d_vector.vi"("Vector"=w1259) -> ("Unit Vector"=w1258:cluster{dbl, dbl, dbl})  [unwired: 3 out]
                n296 = call "normalise_3d_vector.vi"("Vector"=w1249) -> ("magnitude"=w1253:dbl)  [unwired: 3 out]
                n297 = Not Equal To 0?(x=w1253) -> (x != 0?=w1252:bool)
                n298 = call "arb_rotation_matrix.vi"("Unit Vector"=w1258, "theta"=w1253) -> ("Real Matrix"=w1254:T10)
                n299 = case shown="True" w1252 {
                  tunnel: w1257 -> [_ w1268]
                  tunnel: w1256 -> [w1263 w1267]
                  tunnel: [w1263 w1266] -> w1255
                  tunnel: w1254 -> [_ w1265]
                  tunnel: w1248 -> [_ w1264]
                  frame False {
                  }
                  frame True {
                    n300 = for {
                      tunnel: w1268 -> [w1274] mode=indexing
                      tunnel: w1267 -> [w1271] mode=indexing
                      tunnel: [w1270] -> w1266 mode=indexing
                      tunnel: w1265 -> [w1272]
                      tunnel: w1264 -> [w1269]
                      n301 = Unbundle(w1274) -> ("Selected"=w1273:bool)  [unwired: 1 out]
                      n302 = case shown="True" w1273 {
                        tunnel: [w1275 w1278] -> w1270
                        tunnel: w1271 -> [w1275 w1279]
                        tunnel: w1272 -> [_ w1276]
                        tunnel: w1269 -> [_ w1277]
                        frame False {
                        }
                        frame True {
                          n303 = call "apply_matrix_transformation_to_spots.vi"("Transform centre (i.e. transform about this point)"=w1277, "Transformation Matrix (3x3)"=w1276, "Spot In"=w1279) -> ("Spot Out"=w1278:T3)  [unwired: 5 out]
                        }
                      }
                    }
                  }
                }
              }
            }
            n304 = call "coords_real_to_image_currentview.vi"("Position (real coords)"=w1196) -> ("Position (pixels, relative to the top left of the image)"=w1191:cluster{dbl, dbl}, "z (real coords)"=w1195:dbl)  [unwired: 7 in]
            n305 = expression code="z*1e7+20"(w1195) -> (w1207:dbl)
            n306 = In Range and Coerce(upper limit=100.0, x=w1207, lower limit=2.0) -> (coerced(x)=w1194:dbl)  [unwired: 1 out]
            n307 = Bundle("upper limit"=w1194, "upper limit"=w1194) -> (w1187:cluster{"upper limit":dbl, "upper limit":dbl})  [unwired: 1 in]
            n308 = call "myoverlay_oval.vi"("Color"=w1188, "Drawing Mode"=w1189, "Size"=w1187, "Centre Position (pixels on image)"=w1191) -> ("Overlay Elements Out"=w1193:T21[])  [unwired: 5 in]
            n309 = Bundle("radius"=w1185, "radius"=w1185) -> (w1186:cluster{"radius":i16, "radius":i16})  [unwired: 1 in]
            n310 = call "myoverlay_oval.vi"("Color"=w1188, "Drawing Mode"=w1189, "Size"=w1186, "Centre Position (pixels on image)"=w1191, "Overlay Elements In"=w1193) -> ("Overlay Elements Out"=w1192:T21[])  [unwired: 4 in]
            n311 = Multiply(x=w1185, y=cluster{dbl, dbl}[] [{0.0, 0.0}, {1.0, 0.0}, {0.0, 0.0}, {0.0, 1.0}, {0.0, 0.0}, {-1.0, 0.0}, {0.0, 0.0}, {0.0, -1.0}, {0.0, 0.0}]) -> (x*y=w1204:cluster{dbl, dbl}[])
            n312 = Add(x=w1191, y=w1204) -> (x+y=w1190:cluster{dbl, dbl}[])
            n313 = call "myoverlay_lines.vi"("Color"=w1188, "Drawing Mode"=w1189, "Line Endpoints"=w1190, "Overlay Elements In"=w1192) -> ("Overlay Elements Out"=w1184:T21[])  [unwired: 5 in]
          }
          frame "Patterns" {
            n314 = event shown="[3] \"Optimise\": Value Change" {
              selector: _ -> [_ _ _ _ _]
              dyn-events: _ -> [_ _ _ _ _]
              timeout: u32 10 ("milliseconds to wait") -> [_ _ _ _ _]
              tunnel: [w1321 w1351 w1355 w1358 w1369] -> w1304
              tunnel: [w1320 w1352 w1354 w1361 w1370] -> w1303
              tunnel: w1306 -> [w1319 w1351 w1355 w1359 w1368]
              tunnel: w1305 -> [w1318 w1352 w1354 w1361 w1370]
              event "Generate": Value Change {
                # "If there were previous spots, centre the pattern on the spots"
                n315 = event-data() -> ()  [unwired: 1 in, 1 out]
                n316 = call "find_centroid.vi"("Selection and Groups"=w1318, "Spots"=w1319) -> ("size"=w1314:cluster{"x":dbl, "y":dbl, "z":dbl}, "centroid"=w1310:cluster{"x":dbl, "y":dbl, "z":dbl}, "# selected"=w1316:i16)  [unwired: 2 in, 2 out]
                n317 = Greater?(x=w1316, y=i16 1) -> (0:w1311:bool)
                n318 = case shown="False" w1311 {
                  tunnel: w1314 -> [_ w1337]
                  tunnel: [cluster{"x":dbl, "y":dbl, "z":dbl} {"x"=2e-05, "y"=2e-05, "z"=2e-05} ("size") w1337] -> w1313
                  frame False {
                  }
                  frame True {
                  }
                }
                n319 = case shown="\"HCP Shack-Hartmann\"" "Pattern" {
                  tunnel: [w1339 w1342 w1348] -> w1312
                  tunnel: w1313 -> [_ w1341 _]
                  frame "Square Shack-Hartmann" {
                    n320 = call "patterns_square_shack_hartmann.vi"("N"="Spots across centre") -> ("Spots"=w1339:T3[])
                  }
                  frame "HCP Shack-Hartmann" {
                    n321 = Unbundle By Name(w1341) -> ("x"=w1340:dbl)
                    n322 = call "pattern_hcp_shack_hartmann.vi"("Width"=w1340, "Reference Array?"="Reference Array?", "Fraction of SLM"="Fraction of SLM", "N"="Spots across centre") -> ("Shack-Hartmann Spots"=w1342:T3[])  [unwired: 7 in]
                  }
                  frame "Rectangular Grid" {
                    n323 = call "patterns_rectangular_grid.vi"("spacing/m"="spacing/m", "N"="N") -> ("Spots"=w1348:T3[])
                  }
                }
                n324 = local write "Generate"(FALSE ("Generate")) -> ()
                n325 = case shown="True" w1311 {
                  tunnel: w1312 -> [w1324 w1328]
                  tunnel: w1310 -> [_ w1330]
                  tunnel: [w1324 w1326] -> w1322
                  frame False {
                  }
                  frame True {
                    n326 = call "find_centroid.vi"("Spots"=w1328) -> ("centroid"=w1329:cluster{"x":dbl, "y":dbl, "z":dbl}, "# selected"=→"# selected":i16)  [unwired: 3 in, 3 out]
                    n327 = Subtract(x=w1330, y=w1329) -> (x-y=w1327:cluster{"x":dbl, "y":dbl, "z":dbl})
                    n328 = for {
                      tunnel: w1328 -> [w1333] mode=indexing
                      tunnel: w1327 -> [w1332]
                      tunnel: [w1331] -> w1326 mode=indexing
                      n329 = call "extract_position.vi"("Spot"=w1333) -> ("Position"=w1334:cluster{"x":dbl, "y":dbl, "z":dbl})
                      n330 = Add(x=w1334, y=w1332) -> (x+y=w1335:cluster{"x":dbl, "y":dbl, "z":dbl})
                      n331 = call "replace_position.vi"("Position"=w1335, "Spot in"=w1333) -> ("Spot"=w1331:T3)  [unwired: 2 out]
                    }
                  }
                }
                "Last Pattern" <- w1322
                n332 = call "ensure_selection_matches_spots.vi"("Select All (default: no)"=TRUE ("Select All (default: true)"), "Spots"=w1322) -> ("Selection and Groups out"=w1320:T9[], "Spots (duplicate)"=w1321:T3[])  [unwired: 4 in]
              }
              event "Spots across centre", "Fraction of SLM", "Reference Array?", "N", "spacing/m", "Spots across centre": Value Change {
                n333 = event-data() -> ()  [unwired: 1 in, 1 out]
                n334 = local read "Last Pattern"() -> (w1350:T3[])
                n335 = Equal?(x=w1351, y=w1350) -> (x = y?=w1349:bool)
                n336 = case shown="True" w1349 {
                  selector: w1349 -> [_ w1353]
                  frame False {
                  }
                  frame True {
                    n337 = property on="Generate" class="Bool (strict)"("Val(Sgnl)"=w1353) -> ()  [unwired: 2 in, 2 out]
                  }
                }
              }
              event Timeout {
                n338 = event-data() -> ()  [unwired: 1 in, 1 out]
              }
              event "Optimise": Value Change {
                n339 = event-data() -> ()  [unwired: 1 in, 1 out]
                n340 = for {
                  N: "Iterations" -> [_]
                  tunnel: 203 ("Optimisation Resolution") -> [w1365]
                  shift-right: [w1366] -> w1358
                  shift-left: w1359 -> [w1367]
                  tunnel: "Fall-off/m" -> [w1362]
                  n341 = call "do_gsw_step.vi"("Optimisation Resolution"=w1365, "Sinc Zero"=w1362, "Spots In"=w1367) -> ("non-uniformity"=→"non-uniformity":dbl, "efficiency"=→"efficiency":dbl, "Spots Out"=w1366:T3[])  [unwired: 6 in]
                }
              }
              event "Reset Phase/Amplitude": Value Change {
                n342 = event-data() -> ()  [unwired: 1 in, 1 out]
                n343 = for {
                  tunnel: [w1373] -> w1369 mode=indexing
                  tunnel: w1368 -> [w1374] mode=indexing
                  n344 = Bundle By Name(cluster=w1374, "Phase"=0.0, "Amplitude Correction"=0.0) -> (w1373:T3)
                }
              }
            }
          }
          frame "Plugins" {
            # "The local variable ensures the references are  correct when they make it through to the \"close plugins\" block."
            # "This is the error from loading/unloading VIs on the front panel"
            n345 = control-ref of="Plugin Pnl"() -> (w1378:refnum<vi>)
            n346 = Wait (ms)(milliseconds to wait=u32 10) -> ()  [unwired: 1 out]
            n347 = feedback #8() -> (w1377:T5)
            n348 = feedback #9() -> (w1379:errorcluster)
            n349 = event shown="[1] \"Plugin:\": Value Change" {
              selector: _ -> [_ _ _]
              dyn-events: _ -> [_ _ _]
              timeout: 10 -> [_ _ _]
              tunnel: "Abort Plugin" -> [w1386 _ _]
              tunnel: "Plugin:" -> [w1391 _ w1407]
              tunnel: w1379 -> [w1390 w1405 w1409]
              tunnel: [w1389 w1400 w1408] -> w1380
              tunnel: [w1388 w1401 w1411] -> w1376
              tunnel: w1377 -> [w1392 w1402 w1410]
              tunnel: w1378 -> [_ w1403 _]
              event Timeout {
                n350 = event-data() -> ()  [unwired: 1 in, 2 out]
                n351 = Not(x=w1386) -> (.not. x?=w1387:bool)
                n352 = case shown="True" w1387 {
                  tunnel: w1392 -> [w1394 w1399]
                  tunnel: w1391 -> [_ w1398]
                  tunnel: w1390 -> [w1393 w1397]
                  tunnel: [w1393 w1396] -> w1389
                  tunnel: [w1394 w1395] -> w1388
                  frame False {
                  }
                  frame True {
                    n353 = call "plugins_run.vi"("Error In"=w1397, "Plugin Index"=w1398, "Plugins In"=w1399) -> ("Error Out"=w1396:errorcluster, "Plugins"=w1395:T5)  [unwired: 7 in]
                  }
                }
              }
              event "Plugin:": Value Change {
                n354 = event-data() -> ("NewVal"=w1404:u16)  [unwired: 1 in]
                n355 = call "plugins_switch.vi"("error in"=w1405, "Plugin Pnl"=w1403, "Plugin Index"=w1404, "Plugins In"=w1402) -> ("error out"=w1400:errorcluster, "Plugins Out"=w1401:T5)  [unwired: 4 in]
              }
              event "Abort Plugin": Value Change {
                n356 = event-data() -> ("NewVal"=w1406:bool)  [unwired: 1 in]
                n357 = case shown="True" w1406 {
                  tunnel: [w1413 w1418] -> w1411
                  tunnel: w1410 -> [w1413 w1417]
                  tunnel: w1409 -> [w1412 w1416]
                  tunnel: [w1412 w1415] -> w1408
                  tunnel: w1407 -> [_ w1414]
                  frame False {
                  }
                  frame True {
                    n358 = call "plugins_abort.vi"("Error In"=w1416, "Plugin Index"=w1414, "Plugins In"=w1417) -> ("Error Out"=w1415:errorcluster, "Plugins Out"=w1418:T5)  [unwired: 7 in]
                  }
                }
              }
            }
            n359 = feedback-in #8(w1376) -> ()
            n360 = feedback-in #9(w1380) -> ()
            n361 = local write "Plugins"(w1376) -> ()
          }
          frame "Video" {
            # "All the controls on this tab are in the bottom (camera) loop."
            n362 = Wait (ms)(milliseconds to wait=u32 10) -> ()  [unwired: 1 out]
            n363 = property on="Property Node" class="ImageControl"(reference=w1419) -> ("Image Information String"=→"Image Information":string)  [unwired: 1 in, 2 out]
          }
        }
      }
      event "Tab": Value Change {
        w1427 = T22 [enum."Video", enum."Particle Tracking"] items=["Current Spot", "Rotate", "Spot Shape", "Patterns", "Plugins", "Video", "Particle Tracking", "Clamping", "Blank"]
        w1432 = refnum<vi> refnum  # Image
        # "This allows us to disable custom mouse-handling for certain tabs.  It can also be done from within the \"mouse down\" event case."
        n364 = event-data() -> ("NewVal"=w1428:T6)  [unwired: 1 in, 3 out]
        n365 = Equal?(x=w1427, y=w1428) -> (x = y?=w1426:bool[])
        n366 = Or Array Elements(Boolean array=w1426) -> (logical OR=w1425:bool)
        n367 = Not(x=w1425) -> (.not. x?=w1424:bool)
        n368 = Select(t=w1431, s=w1424, f=w1432) -> (s? t:f=w1433:refnum<vi>)
        n369 = register-events(reference=w1435, w1433, w1432, w1432, w1432) -> (reference out=w1434:refnum<event-registration>)  [unwired: 1 in, 1 out]
      }
      event Menu Selection (User) {
        n370 = event-data() -> ("ItemTag"=w1443:string, "MenuRef"=w1436:refnum<k9>)  [unwired: 1 in]
        n371 = case shown="\"ToggleSavingData\"" w1443 {
          tunnel: w1447 -> [w1451 w1461 w1470 w1484 w1503 w1507 w1510 w1517 w1524 w1526 w1529 w1558 w1584 w1605 w1616 w1627 w1630 w1632 w1637 w1640]
          tunnel: w1446 -> [w1450 w1460 w1469 w1493 w1502 w1506 w1508 w1515 w1523 w1525 w1528 w1557 w1583 w1604 w1615 w1626 w1629 w1633 w1638 w1639]
          tunnel: [w1451 w1461 w1470 w1484 w1501 w1504 w1510 w1517 w1524 w1526 w1529 w1558 w1584 w1605 w1616 w1627 w1630 w1632 w1637 w1640] -> w1445
          tunnel: [w1450 w1460 w1469 w1493 w1500 w1505 w1509 w1516 w1522 w1527 w1530 w1557 w1583 w1604 w1615 w1626 w1629 w1633 w1638 w1639] -> w1444
          tunnel: [_ _ _ _ TRUE _ _ _ _ _ _ _ _ _ _ _ _ _ _ _] -> w1438
          tunnel: w1437 -> [_ _ _ _ _ _ _ _ _ _ _ w1556 w1582 w1596 _ _ _ _ _ _]
          tunnel: w1436 -> [_ _ _ _ _ _ _ _ _ _ _ w1547 w1576 w1599 w1610 w1621 _ _ _ _]
          frame "ToggleSavingData" {
            # "Data is saved from the middle loop: look there for an explanation."
            n372 = local read "Save Video"() -> (w1449:bool)
            n373 = Not(x=w1449) -> (.not. x?=w1448:bool)
            n374 = local write "Save Video"(w1448) -> ()
          }
          frame "SaveStateToFile" {
            # "Save the current settings (i.e. the values of all the controls in VIs that have [Red Tweezers Save Settings] in their documentation string) to a file."
            n375 = call "File Dialog"("prompt"="Please select a location to save the settings", "button label"="Save", "default name"="red_tweezers_settings.xml", "pattern (all files)"="*.xml" ("pattern label"), "pattern label"="XML Settings Files") -> ("selected path"=w1459:path, "cancelled"=w1452:bool)  [unwired: 7 in, 2 out]
            n376 = Not(x=w1452) -> (.not. x?=w1453:bool)
            n377 = case shown="True" w1453 {
              tunnel: w1459 -> [_ w1463]
              frame False {
              }
              frame True {
                n378 = Path To String(path=w1463) -> (string=w1462:string)
                n379 = call "settings_save_to_file.vi"("XML File Path"=w1463) -> ()  [unwired: 11 in]
                n380 = call "settings_filename_to_registry.vi"("Last Used Settings File"=w1462) -> ()  [unwired: 11 in]
              }
            }
          }
          frame "SaveStateToCurrentFile" {
            # "As SaveStateToFile, but using the current file (i.e. Save not Save As...)."
            n381 = global read "red_tweezers_globals_INTERNAL_VOLATILE.vi" "Current Settings File"() -> (w1468:path)
            n382 = call <vilib>:"Check if File or Folder Exists.vi"("path"=w1468) -> ("file or folder exists?"=w1467:bool, "dup path"=w1466:path)  [unwired: 8 in, 1 out]
            n383 = case shown="True" w1467 {
              selector: w1467 -> [_ w1481]
              tunnel: w1466 -> [_ w1482]
              tunnel: [w1473 w1482] -> w1465
              tunnel: [w1474 w1481] -> w1464
              frame False {
                n384 = call "File Dialog3"("prompt"="Please select a location to save the settings", "button label"="Save", "default name"="red_tweezers_settings.xml", "pattern (all files)"="*.xml" ("pattern label"), "pattern label"="XML Settings Files") -> ("selected path"=w1473:path, "cancelled"=w1480:bool)  [unwired: 7 in, 2 out]
                n385 = Not(x=w1480) -> (.not. x?=w1474:bool)
              }
              frame True {
              }
            }
            n386 = case shown="True" w1464 {
              tunnel: w1465 -> [_ w1472]
              frame False {
              }
              frame True {
                n387 = Path To String(path=w1472) -> (string=w1471:string)
                n388 = call "settings_save_to_file.vi"("XML File Path"=w1472) -> ()  [unwired: 11 in]
                n389 = call "settings_filename_to_registry.vi"("Last Used Settings File"=w1471) -> ()  [unwired: 11 in]
              }
            }
          }
          frame "LoadStateFromFile" {
            # "Load a file, and use it to reset the values of all the front panel controls."
            # "We need to re-run the initialisation stuff in UDP sender after changing settings\n(for example, this synchronises the settings like camera pixel size with the\nrelevant global variable)"
            n390 = call "File Dialog2"("prompt"="Please select a settings file", "button label"="Open", "default name"="red_tweezers_settings.xml", "pattern (all files)"="*.xml" ("pattern label"), "pattern label"="XML Settings Files") -> ("selected path"=w1485:path, "cancelled"=w1492:bool)  [unwired: 7 in, 2 out]
            n391 = Not(x=w1492) -> (.not. x?=w1491:bool)
            n392 = case shown="False" w1491 {
              selector: w1491 -> [w1494 w1495]
              tunnel: w1485 -> [_ w1496]
              tunnel: [w1494 w1495] -> w1483
              frame False {
              }
              frame True {
                n393 = call "settings_load_from_file.vi"("XML File Path"=w1496) -> ()  [unwired: 9 in, 2 out]
                n394 = Path To String(path=w1496) -> (string=w1497:string)
                n395 = call "settings_filename_to_registry.vi"("Last Used Settings File"=w1497) -> ()  [unwired: 11 in]
              }
            }
            n396 = call "UDP Sender generic_2.vi"("re-initialise"=w1483, "Spots"=w1484) -> ()  [unwired: 1 in, 1 out]
          }
          frame "Undo" {
            # "This should get the last undo vector and replace the spots with it :)"
            n397 = call "red_tweezers_UNDO.vi"("Selection/Group"=w1502, "Undo/Store (store, False)"=TRUE, "Spots"=w1503) -> ("Selection/Group Out (Undo only)"=w1500:T9[], "Spots Out (Undo only)"=w1501:T3[])  [unwired: 7 in]
          }
          frame "Delete" {
            n398 = call "delete_selected_spots.vi"("Selection/Group 3"=w1506, "Spots 3"=w1507) -> ("Selection/Group 2"=w1505:T9[], "Spots 2"=w1504:T3[])  [unwired: 4 in]
          }
          frame "SelectAllSpots" {
            n399 = for {
              tunnel: w1508 -> [w1513] mode=indexing
              tunnel: [w1514] -> w1509 mode=indexing
              n400 = Unbundle(w1513) -> ("Group ID"=w1512:i32)  [unwired: 1 out]
              n401 = Bundle(cluster=w1513, "Group ID"=w1512, "Selected"=TRUE ("Label.Visible")) -> (w1514:T9)
            }
          }
          frame "SelectNoSpots" {
            n402 = for {
              tunnel: w1515 -> [w1520] mode=indexing
              tunnel: [w1521] -> w1516 mode=indexing
              n403 = Unbundle(w1520) -> ("Group ID"=w1519:i32)  [unwired: 1 out]
              n404 = Bundle(cluster=w1520, "Group ID"=w1519, "Selected"=FALSE ("Label.Visible")) -> (w1521:T9)
            }
          }
          frame "SelectSpecificSpots" {
            n405 = call "select_by_id.vi"("Selection/Group"=w1523, "Spots"=w1524) -> ("Selection/Group Out"=w1522:T9[])  [unwired: 9 in]
          }
          frame "Group" {
            # "Group the currently selected spots"
            n406 = call "group_selected_spots.vi"("Selection/Group 2"=w1525) -> ("Array"=w1527:T9[])
          }
          frame "Ungroup" {
            # "Ungroup the currently selected spots"
            n407 = for {
              tunnel: [w1534] -> w1530 mode=indexing
              tunnel: w1528 -> [w1533] mode=indexing
              tunnel: 0 -> [w1532]
              n408 = Unbundle(w1533) -> ("Selected"=w1535:bool)  [unwired: 1 out]
              n409 = case shown="False" w1535 {
                tunnel: [w1536 w1539] -> w1534
                tunnel: w1533 -> [w1536 w1538]
                tunnel: w1532 -> [_ w1537]
                frame False {
                }
                frame True {
                  n410 = Unbundle(w1538) -> ("Selected"=w1540:bool)  [unwired: 1 out]
                  n411 = Bundle(cluster=w1538, "Group ID"=w1537, "Selected"=w1540) -> (w1539:T9)
                }
              }
            }
          }
          frame "ZoomIn" {
            w1541 = "ZoomToFit" ("item tag")
            # "turn off \"zoom to fit\""
            n412 = property class="ImageControl"(reference=w1556) -> (reference out=w1550:refnum<vi>, "ZoomSingle"=w1555:cluster{"X":sgl, "Y":sgl}, "Image Center Position"=w1548:cluster{"X":u32, "Y":u32})  [unwired: 1 in, 1 out]
            n413 = Unbundle(w1555) -> ("X"=w1553:sgl)  [unwired: 1 out]
            n414 = Round To Nearest(number=w1553) -> (nearest integer value=w1549:sgl)
            n415 = Greater Than 0?(x=w1549) -> (x > 0?=w1554:bool)
            n416 = case shown="True" w1554 {
              tunnel: w1553 -> [w1563 w1566]
              tunnel: [w1562 w1564] -> w1552
              frame False {
                n417 = Reciprocal(x=w1563) -> (1/x=w1560:sgl)
                n418 = Round Toward +Infinity(x=w1560) -> (ceil(x): smallest int >= x=w1561:sgl)
                n419 = Decrement(x=w1561) -> (x-1=w1559:sgl)
                n420 = Reciprocal(x=w1559) -> (1/x=w1562:sgl)
              }
              frame True {
                n421 = Round Toward -Infinity(1:w1566) -> (0:w1565:sgl)
                n422 = Increment(x=w1565) -> (x+1=w1564:sgl)
              }
            }
            n423 = Bundle(w1552, w1552) -> (w1551:cluster{sgl, sgl})  [unwired: 1 in]
            n424 = property class="ImageControl"(reference=w1550, "ZoomSingle"=w1551, "Image Center Position"=w1548) -> ()  [unwired: 1 in, 2 out]
            n425 = Get Menu Item Info(7:w1541, 11:w1547) -> (1:w1544:bool, 2:w1545:string, 3:w1546:refnum<k9>, 6:w1543:T23)  [unwired: 1 in, 3 out]
            n426 = Set Menu Item Info(4:w1543, 6:FALSE ("checked"), 7:w1541, 9:w1544, 10:w1545, 11:w1546) -> ()  [unwired: 1 in, 2 out]
          }
          frame "ZoomOut" {
            w1570 = "ZoomToFit" ("item tag")
            # "turn off \"zoom to fit\""
            n427 = property class="ImageControl"(reference=w1582) -> (reference out=w1578:refnum<vi>, "ZoomSingle"=w1581:cluster{"X":sgl, "Y":sgl}, "Image Center Position"=w1577:cluster{"X":u32, "Y":u32})  [unwired: 1 in, 1 out]
            n428 = Unbundle(w1581) -> ("X"=w1567:sgl)  [unwired: 1 out]
            n429 = Greater?(x=w1567, y=1.0) -> (0:w1569:bool)
            n430 = case shown="False" w1569 {
              tunnel: w1567 -> [w1591 w1594]
              tunnel: [w1590 w1592] -> w1580
              frame False {
                n431 = Reciprocal(x=w1591) -> (1/x=w1588:sgl)
                n432 = Add(x=w1588, y=sgl 0.01 ("x")) -> (x+y=w1586:sgl)
                n433 = Round Toward -Infinity(1:w1586) -> (0:w1589:sgl)
                n434 = Increment(x=w1589) -> (x+1=w1587:sgl)
                n435 = Reciprocal(x=w1587) -> (1/x=w1590:sgl)
              }
              frame True {
                n436 = Round Toward +Infinity(x=w1594) -> (ceil(x): smallest int >= x=w1593:sgl)
                n437 = Decrement(x=w1593) -> (x-1=w1592:sgl)
              }
            }
            n438 = Bundle(w1580, w1580) -> (w1579:cluster{sgl, sgl})  [unwired: 1 in]
            n439 = property class="ImageControl"(reference=w1578, "ZoomSingle"=w1579, "Image Center Position"=w1577) -> ()  [unwired: 1 in, 2 out]
            n440 = Get Menu Item Info(7:w1570, 11:w1576) -> (1:w1573:bool, 2:w1574:string, 3:w1575:refnum<k9>, 6:w1572:T23)  [unwired: 1 in, 3 out]
            n441 = Set Menu Item Info(4:w1572, 6:FALSE ("checked"), 7:w1570, 9:w1573, 10:w1574, 11:w1575) -> ()  [unwired: 1 in, 2 out]
          }
          frame "ZoomToFit" {
            w1600 = "ZoomToFit" ("item tag")
            # "and make sure the image obeys the result"
            # "Toggle menu checkmark"
            n442 = Get Menu Item Info(7:w1600, 11:w1599) -> (1:w1598:bool, 2:w1602:string, 3:w1603:refnum<k9>, 4:w1597:bool, 6:w1601:T23)  [unwired: 1 in, 2 out]
            n443 = Not(x=w1597) -> (.not. x?=w1595:bool)
            n444 = Set Menu Item Info(4:w1601, 6:w1595, 7:w1600, 9:w1598, 10:w1602, 11:w1603) -> ()  [unwired: 1 in, 2 out]
            n445 = property class="ImageControl"(reference=w1596, "Zoom to Fit Mode"=w1595) -> ()  [unwired: 1 in, 2 out]
          }
          frame "ShowGrid" {
            w1611 = "ShowGrid" ("item tag")
            # "Toggle menu checkmark"
            n446 = Get Menu Item Info(7:w1611, 11:w1610) -> (1:w1609:bool, 2:w1613:string, 3:w1614:refnum<k9>, 4:w1608:bool, 6:w1612:T23)  [unwired: 1 in, 2 out]
            n447 = Not(x=w1608) -> (.not. x?=w1607:bool)
            n448 = Set Menu Item Info(4:w1612, 6:w1607, 7:w1611, 9:w1609, 10:w1613, 11:w1614) -> ()  [unwired: 1 in, 2 out]
            n449 = call "grid_and_guides.vi"("Boolean"=w1607, "Operation"=T16."Set grid visibility") -> ()  [unwired: 9 in, 1 out]
          }
          frame "ShowGuides" {
            w1622 = "ShowGuides" ("item tag")
            # "Toggle menu checkmark"
            n450 = Get Menu Item Info(7:w1622, 11:w1621) -> (1:w1620:bool, 2:w1624:string, 3:w1625:refnum<k9>, 4:w1619:bool, 6:w1623:T23)  [unwired: 1 in, 2 out]
            n451 = Not(x=w1619) -> (.not. x?=w1618:bool)
            n452 = Set Menu Item Info(4:w1623, 6:w1618, 7:w1622, 9:w1620, 10:w1624, 11:w1625) -> ()  [unwired: 1 in, 2 out]
            n453 = call "grid_and_guides.vi"("Boolean"=w1618, "Operation"=T16."Set guide visibility") -> ()  [unwired: 9 in, 1 out]
          }
          frame "ConfigureGridAndGuides" {
            n454 = call "grid_and_guides.vi"("Operation"=T16."Show front panel") -> ()  [unwired: 10 in, 1 out]
          }
          frame "ShowSettings" {
            n455 = call "UDP Sender generic_2.vi"("Show panel"=TRUE, "Spots"=w1632) -> ()  [unwired: 1 in, 1 out]
          }
          frame "CameraSettings" {
            n456 = global read "red_tweezers_globals_INTERNAL_VOLATILE.vi" "Current Camera VI"() -> (w1635:path)
            n457 = Open VI Reference(vi path=w1635) -> (vi reference=w1634:refnum<vi>)  [unwired: 5 in, 1 out]
            n458 = property class="VI"(reference=w1634, "Front Panel.Open"=TRUE ("Front Panel Window:Open")) -> ()  [unwired: 1 in, 2 out]
          }
          frame Default {
          }
        }
      }
      event Mouse Down? {
        # "We don't process clicks when the user is on the video tab, so that we can set ROIs."
        # "When the mouse button goes down over the image, we save where it went down, etc. and wait to see what happens next.  We also register to be told when the mouse leaves the control, goes up, or moves.  \"click\" or \"drag\" are only detected once the mouse moves or goes up."
        n459 = event-data() -> ("Coords"=w1655:T24, "Button"=w1650:u16, "Mods"=w1659:cluster{"Double Click":bool, "Menu Key":bool}, "PlatMods"=w1658:T25)  [unwired: 1 in]
        n460 = call "mouse_to_image_coords.vi"("Mouse Coords (screen/pane units)"=w1655, "Image Control"=w1651) -> ("Cursor is on Display Area"=w1649:bool, "Mouse Coords (image pixels)"=w1654:cluster{dbl, dbl})  [unwired: 4 in]
        n461 = disable-structure shown="Enabled" {
          disable-tunnel: w1650 -> [w1667 _]
          disable-tunnel: w1649 -> [w1665 w1668]
          disable-tunnel: [w1664 w1668] -> w1645
          frame Enabled {
            n462 = Equal?(x=u16 1, y=w1667) -> (x = y?=w1666:bool)
            n463 = And(x=w1665, y=w1666) -> (x .and. y?=w1664:bool)
          }
          frame Disabled {
            # "use other pane to allow right-clicking on image"
          }
        }
        n464 = local read "Tab"() -> (w1646:T6)
        n465 = Not Equal?(x=w1646, y=T17."Video" ("Tab")) -> (x != y?=w1644:bool)
        n466 = And(x=w1645, y=w1644) -> (x .and. y?=w1643:bool)
        n467 = case shown="False" w1643 {
          tunnel: w1662 -> [w1671 w1682]
          tunnel: [T13 {"Button Down"=FALSE, "Dragging"=FALSE, "Position (Image Pixels)"={"X"=0.0, "Y"=0.0}, "Previous Position (Image Pixels)"={"X"=0.0, "Y"=0.0}, "Button"=0, "Mods"={"Double Click"=FALSE, "Menu Key"=FALSE}, "PlatMods"={"Shift"=FALSE, "Ctrl"=FALSE, "Alt"=FALSE, "Cmd"=FALSE, "Opt"=FALSE}} w1681] -> w1661
          tunnel: [w1671 w1678] -> w1660
          tunnel: w1650 -> [_ w1677]
          tunnel: w1659 -> [_ w1676]
          tunnel: w1658 -> [_ w1675]
          tunnel: w1654 -> [_ w1674]
          tunnel: [FALSE TRUE] -> w1653
          tunnel: w1651 -> [_ w1672]
          frame False {
            # "If the user clicked on a scrollbar, ignore it and let LabVIEW handle it. (this keeps the scrollbars working)"
          }
          frame True {
            w1680 = FALSE  # Dragging
            w1679 = TRUE  # Button Down
            n468 = register-events(reference=w1682, w1672, w1672, w1672, w1672) -> (reference out=w1678:refnum<event-registration>)  [unwired: 1 in, 1 out]
            n469 = Bundle("Button Down"=w1679, "Dragging"=w1680, "Mouse Coords (image pixels)"=w1674, "Mouse Coords (image pixels)"=w1674, "Button"=w1677, "Mods"=w1676, "PlatMods"=w1675) -> (w1681:T26)  [unwired: 1 in]
          }
        }
        n470 = Array Size(array=w1641) -> (size(s)=w1642:i32)
        n471 = local write "# of Spots"(w1642) -> ()
        n472 = local write "Selection/Group"(w1641) -> ()
        n473 = event-data("Discard?"=w1653) -> ()  [unwired: 4 in, 1 out]
      }
      event Mouse Leave {
        w1689 = refnum<vi> refnum  # Dummy
        # "When the mouse leaves, we reset things."
        n474 = event-data() -> ()  [unwired: 1 in, 2 out]
        n475 = register-events(reference=w1690, w1688, w1689, w1689, w1689) -> (reference out=w1687:refnum<event-registration>)  [unwired: 1 in, 1 out]
      }
      event Mouse Up {
        w1709 = refnum<vi> refnum  # Dummy
        # "Double clicking adds a spot at the mouse position."
        # "deregister"
        # "If we get here the mouse has gone down and up again.  If we've not moved in between, we have a Click.\nEither way we're no longer interested in mouse leave/move/up events."
        n476 = event-data() -> ("Mods"=w1696:cluster{"Double Click":bool, "Menu Key":bool})  [unwired: 1 in, 5 out]
        n477 = Unbundle By Name(w1702) -> ("Dragging"=w1711:bool)
        n478 = Unbundle By Name(w1696) -> ("Double Click"=w1693:bool)
        n479 = Not(x=w1711) -> (.not. x?=w1710:bool)
        n480 = Not(x=w1698) -> (.not. x?=w1700:bool)
        n481 = And(x=w1710, y=w1700) -> (x .and. y?=w1694:bool)
        n482 = case shown="True" w1694 {
          tunnel: w1702 -> [_ w1717]
          tunnel: w1704 -> [w1712 w1716]
          tunnel: w1703 -> [w1713 w1719]
          tunnel: [w1713 w1718] -> w1705
          tunnel: w1693 -> [_ w1714]
          tunnel: [w1712 w1715] -> w1695
          frame False {
          }
          frame True {
            n483 = case shown="True" w1714 {
              tunnel: w1719 -> [w1726 w1776]
              tunnel: [w1724 w1782] -> w1718
              tunnel: w1716 -> [w1720 w1783]
              tunnel: w1717 -> [w1723 w1778]
              tunnel: [w1720 w1774] -> w1715
              frame False {
                w1730 = 400.0  # 20^2 px
                # "If the user clicked, determine which spots should be selected: if we've clicked a spot/group then select it.  Shift-clicking toggles selection for that spot, and leaves the rest of the selection unchanged."
                # "check we're close enough"
                # "find closest"
                n484 = Unbundle By Name(w1723) -> ("Position (Image Pixels)"=w1722:cluster{"X":dbl, "Y":dbl}, "PlatMods.Shift"=w1721:bool)
                n485 = for {
                  tunnel: [w1766] -> w1728 mode=indexing
                  tunnel: w1722 -> [w1765]
                  tunnel: w1720 -> [w1764] mode=indexing
                  # "calculate distances between mouse position and spot positions"
                  n486 = call "extract_position.vi"("Spot"=w1764) -> ("Position"=w1763:cluster{"x":dbl, "y":dbl, "z":dbl})
                  n487 = call "coords_real_to_image_currentview.vi"("Position (real coords)"=w1763) -> ("Position (pixels, relative to the top left of the image)"=w1762:cluster{dbl, dbl})  [unwired: 7 in, 1 out]
                  n488 = Subtract(x=w1762, y=w1765) -> (x-y=w1769:cluster{dbl, dbl})
                  n489 = Multiply(x=w1769, y=w1769) -> (x*y=w1768:cluster{dbl, dbl})
                  n490 = Cluster To Array(cluster=w1768) -> (array=w1767:dbl[])
                  n491 = Add Array Elements(numeric array=w1767) -> (sum=w1766:dbl)
                }
                n492 = Array Max & Min(array=w1728) -> (min value=w1729:dbl, min index (indices)=w1725:i32)  [unwired: 2 out]
                n493 = Less Or Equal?(x=w1729, y=w1730) -> (x <= y?=w1727:bool)
                n494 = case shown="True" w1727 {
                  tunnel: w1726 -> [w1731 w1738]
                  tunnel: w1725 -> [_ w1732]
                  tunnel: w1721 -> [_ w1734]
                  tunnel: [w1731 w1733] -> w1724
                  frame False {
                    # "If we didn't click a spot, do nothing."
                  }
                  frame True {
                    # "If the spot is in a group, act on all spots in that group, not just the spot we clicked."
                    # "This case statement toggles the selection of the spot/group we clicked, and leaves other spots unchanged if we're holding shift.  Otherwise, we select the spot/group that was clicked and deselect everything else."
                    n495 = stacked-sequence {
                      tunnel: w1732 -> [_ w1740]
                      frame #0 {
                        n496 = local read "Current Spot #"() -> (→"Prev Current Spot":dbl)
                      }
                      frame #1 {
                        "Current Spot #" <- w1740
                      }
                    }
                    n497 = Index Array(array=w1738, index=w1732) -> (element=w1737:T9)
                    n498 = Unbundle(w1737) -> ("Group ID"=w1735:i32)  [unwired: 1 out]
                    n499 = Greater Than 0?(x=w1735) -> (x > 0?=w1736:bool)
                    n500 = for {
                      tunnel: w1738 -> [w1751] mode=indexing
                      tunnel: w1736 -> [w1748]
                      tunnel: w1735 -> [w1747]
                      tunnel: w1732 -> [w1746]
                      tunnel: w1734 -> [w1744]
                      tunnel: [w1742] -> w1733 mode=indexing
                      i -> [w1745]
                      n501 = Unbundle(w1751) -> ("Group ID"=w1741:i32, "Selected"=w1749:bool)
                      n502 = case shown="True" w1748 {
                        tunnel: w1741 -> [_ w1755]
                        tunnel: [w1753 w1757] -> w1743
                        tunnel: w1747 -> [_ w1756]
                        tunnel: w1746 -> [w1754 _]
                        tunnel: w1745 -> [w1752 _]
                        frame False {
                          n503 = Equal?(x=w1752, y=w1754) -> (x = y?=w1753:bool)
                        }
                        frame True {
                          n504 = Equal?(x=w1755, y=w1756) -> (x = y?=w1757:bool)
                        }
                      }
                      n505 = case shown="True" w1744 {
                        tunnel: [w1758 w1759] -> w1750
                        tunnel: w1749 -> [_ w1760]
                        tunnel: w1743 -> [w1758 w1761]
                        frame False {
                        }
                        frame True {
                          n506 = Exclusive Or(1:w1761, 2:w1760) -> (0:w1759:bool)
                        }
                      }
                      n507 = Bundle("Group ID"=w1741, w1750) -> (w1742:cluster{"Group ID":i32, bool})  [unwired: 1 out]
                    }
                  }
                }
              }
              frame True {
                # "convert mouse position to real coords, and add a spot there."
                # "Double-click detected"
                n508 = Unbundle By Name(w1778) -> ("Position (Image Pixels)"=w1777:cluster{"X":dbl, "Y":dbl})
                n509 = for {
                  tunnel: w1776 -> [w1786] mode=indexing
                  tunnel: [w1785] -> w1775 mode=indexing
                  n510 = Bundle(cluster=w1786, "Selected"=FALSE) -> (w1785:T9)  [unwired: 1 in]
                }
                n511 = call "coords_image_to_real_currentimage.vi"("Position (pixels on image)"=w1777) -> ("Position (real coords)"=w1779:cluster{dbl, dbl, "Z":dbl})  [unwired: 9 in]
                n512 = call "replace_position.vi"("Position"=w1779) -> ("Spot"=w1781:T3)  [unwired: 3 in]
                n513 = Build Array (concatenate)(w1783, w1781) -> (w1774:T3[])
                n514 = Build Array (concatenate)(w1775, T9 {"Group ID"=0, "Selected"=TRUE} ("selection_element")) -> (w1782:T9[])
                n515 = Array Size(array=w1774) -> (size(s)=w1773:i32)
                n516 = local write "Induce check"(TRUE) -> ()
                n517 = Subtract(x=w1773, y=1) -> (x-y=w1772:i32)
                n518 = local write "Current Spot #"(w1772) -> ()
              }
            }
          }
        }
        n519 = register-events(reference=w1707, w1706, w1709, w1709, w1709) -> (reference out=w1708:refnum<event-registration>)  [unwired: 1 in, 1 out]
      }
      event Mouse Move {
        n520 = event-data() -> ("Coords"=w1801:T24)  [unwired: 1 in, 2 out]
        n521 = call "mouse_to_image_coords.vi"("Mouse Coords (screen/pane units)"=w1801, "Image Control"=w1800) -> ("Mouse Coords (image pixels)"=w1792:cluster{dbl, dbl})  [unwired: 4 in, 1 out]
        n522 = Not(x=w1791) -> (.not. x?=w1796:bool)
        n523 = case shown="True" w1796 {
          tunnel: w1794 -> [_ w1814]
          tunnel: w1799 -> [w1806 w1816]
          tunnel: w1798 -> [w1805 w1815]
          tunnel: [w1805 w1815] -> w1787
          tunnel: [w1806 w1817] -> w1797
          tunnel: w1792 -> [_ w1808]
          tunnel: w1788 -> [_ w1807]
          frame False {
          }
          frame True {
            # "this is the displacement of the mouse, since the last iteration, in \"real\" coordinates (NB the conversions go before subtracting, as it may involve adding a constant as well as multiplying, which would confuse things as we're only interested in displacements here."
            # "The \"position\" local variable is there just in case we're on the \"current spot\" tab, so that the position updates nicely"
            # "If the user is dragging, translate the spots.\nHolding down shift causes the mouse's motion to be transformed into scaling about the centroid of the spots and rotation about the same point"
            n524 = Unbundle By Name(w1814) -> ("Position (Image Pixels)"=w1809:cluster{"X":dbl, "Y":dbl})
            n525 = call "find_centroid.vi"("Selection and Groups"=w1815, "Spots"=w1816) -> ("centroid"=w1810:cluster{"x":dbl, "y":dbl, "z":dbl})  [unwired: 2 in, 4 out]
            n526 = Unbundle By Name(w1814) -> ("PlatMods.Shift"=w1813:bool)
            n527 = disable-structure shown="Disabled" {
              disable-tunnel: w1810 -> [w1818 _]
              frame Disabled {
                n528 = local write "Position"(w1818) -> ()
              }
              frame Enabled {
              }
            }
            n529 = call "coords_image_to_real_currentimage.vi"("Position (pixels on image)"=w1808) -> ("Position (real coords)"=w1811:cluster{dbl, dbl, "Z":dbl})  [unwired: 9 in]
            n530 = call "coords_image_to_real_currentimage.vi"("Position (pixels on image)"=w1809) -> ("Position (real coords)"=w1812:cluster{dbl, dbl, "Z":dbl})  [unwired: 9 in]
            n531 = case shown="False" w1813 {
              tunnel: [w1823 w2097] -> w1817
              tunnel: w1816 -> [w1829 w2098]
              tunnel: w1815 -> [w1828 w2096]
              tunnel: w1812 -> [w1827 w2083]
              tunnel: w1810 -> [_ w2093]
              tunnel: w1811 -> [w1824 w2084]
              tunnel: w1807 -> [_ _]
              frame False {
                # "Spot Checker passes on information for the bubble collision,system so proper calculations can be made."
                n532 = while {
                  tunnel: w1827 -> [w1868]
                  tunnel: [w1858] -> w1825
                  tunnel: w1824 -> [w1857]
                  i -> [w1851]
                  stop <- w1853 stop-if-true
                  w1843 = 0
                  # "This while loop statement makes sure\nthat every spot gets checked before \nallowing any spot to move."
                  # "Buffer zone controls the amount of space between the\ncenter of a spot compared to the center of another spot.\nThis is used to prevent bubbles from colliding with each other."
                  # "Projected distance calculates the distance between two spots- this is used for when a \"hit\" occurs. If the projected distance becomes larger than the previous distance, the program will assume that the spot is being pulled from the buffer zone and as a result will allow the bubble to exit."
                  # "This subVI leads to the distance function, which outputs the distance between a spot being checked compared to the current spot number."
                  n533 = control-ref of="Value Check"() -> (w1848:refnum<vi>)
                  n534 = control-ref of="ID num check"() -> (w1847:refnum<vi>)
                  n535 = control-ref of="Spot Checker"() -> (w1864:refnum<vi>)
                  n536 = Subtract(x=w1857, y=w1868) -> (x-y=w1858:cluster{dbl, dbl, "Z":dbl})
                  n537 = call "DistanceFunction.vi"("Condition Driver"=FALSE, "Position (real coords)"=w1868, "Current Spot Number"=w1847, "Spot Checker"=w1864, "Spot Number Being Checked"=w1848) -> ("Distance"=w1830:dbl)  [unwired: 6 in]
                  n538 = stacked-sequence {
                    tunnel: w1830 -> [_ w1873]
                    frame #0 {
                      n539 = local read "Distance"() -> (→"Previous Distance":dbl)
                    }
                    frame #1 {
                      "Distance" <- w1873
                    }
                  }
                  n540 = Unbundle(w1858) -> (→"X Displacement":dbl, →"Y Displacement":dbl)  [unwired: 1 out]
                  n541 = control-ref of="ID num check"() -> (w1849:refnum<vi>)
                  n542 = control-ref of="Spot Checker"() -> (w1862:refnum<vi>)
                  n543 = control-ref of="Y Displacement"() -> (w1860:refnum<vi>)
                  n544 = control-ref of="Value Check"() -> (w1850:refnum<vi>)
                  n545 = control-ref of="X Displacement"() -> (w1861:refnum<vi>)
                  n546 = call "ProjectedDistance.vi"("X Displacement"=w1861, "Spot Number Check"=w1850, "Current Spot #"=w1849, "Spot Checker"=w1862, "Y Displacement"=w1860) -> ("Numeric"=→"Projected Distance":dbl)  [unwired: 6 in]
                  n547 = local read "Projected Distance"() -> (w1836:dbl)
                  n548 = Multiply(x="Buffer Zone", y=2) -> (x*y=w1867:dbl)
                  n549 = Less Or Equal?(x=w1830, y=w1867) -> (x <= y?=w1837:bool)
                  n550 = Not Equal?(x=w1836, y=0) -> (x != y?=w1834:bool)
                  n551 = And(x=w1837, y=w1834) -> (x .and. y?=w1831:bool)
                  "Hit" <- w1831
                  n552 = local read "ID num check"() -> (w1844:dbl)
                  n553 = local read "Value Check"() -> (w1845:dbl)
                  n554 = Equal?(x=w1830, y=0) -> (x = y?=w1833:bool)
                  n555 = case shown="False" w1833 {
                    frame False {
                      n556 = local read "Hit"() -> (w1870:bool)
                      n557 = local write "Hit Indicator"(w1870) -> ()
                    }
                    frame True {
                      "Hit Indicator" <- FALSE
                    }
                  }
                  n558 = Equal?(x=w1844, y=w1843) -> (x = y?=w1842:bool)
                  n559 = Equal?(x=w1843, y=w1845) -> (x = y?=w1841:bool)
                  n560 = Not(x=w1831) -> ()  [unwired: 1 out]
                  n561 = And(x=w1842, y=w1841) -> (x .and. y?=w1840:bool)
                  n562 = Or(x=w1831, y=w1840) -> (x .or. y?=w1846:bool)
                  n563 = case shown="True" w1846 {
                    frame False {
                      n564 = stacked-sequence {
                        frame #0 {
                          n565 = local read "Potential Collisions"() -> (w1876:dbl)
                          n566 = local read "Spot # Check"() -> (w1878:dbl)
                          n567 = Subtract(x=w1876, y=1) -> (x-y=w1874:dbl)
                          n568 = Less Or Equal?(x=w1878, y=w1874) -> (x <= y?=w1877:bool)
                          n569 = case shown="True" w1877 {
                            frame False {
                              # "Spot # Check resets if the the number of potential collisons is more than Spot # Check."
                              n570 = local write "Spot # Check"(0) -> ()
                            }
                            frame True {
                              n571 = stacked-sequence {
                                frame #0 {
                                # "Spot # Check increments by 1 every time it is greater than the # of potential collisions."
                                n572 = local read "Spot # Check"() -> (w1882:dbl)
                                n573 = Add(x=w1882, y=1) -> (x+y=→"Spot # Check":dbl)
                                }
                                frame #1 {
                                # "Spot # Check resets if the Spot # Check is eqaul to the # of potential collisions."
                                n574 = local read "Potential Collisions"() -> (w1883:dbl)
                                n575 = local read "Spot # Check"() -> (w1884:dbl)
                                n576 = Equal?(x=w1884, y=w1883) -> (x = y?=w1885:bool)
                                n577 = case shown="True" w1885 {
                                frame False {
                                }
                                frame True {
                                n578 = local write "Spot # Check"(0) -> ()
                                }
                                }
                                }
                                frame #2 {
                                n579 = local read "Spot Checker"() -> (w1900:T3[])
                                n580 = local read "Current Spot #"() -> (w1901:dbl)
                                n581 = local read "Area to check"() -> (w1887:dbl)
                                n582 = Index Array(array=w1900, index=w1901) -> (element=w1899:T3)
                                n583 = local read "Orig Y SC"() -> (w1896:dbl)
                                n584 = Unbundle By Name(w1899) -> ("Position.x"=w1897:dbl, "Position.y"=w1895:dbl)
                                n585 = local read "Orig X SC"() -> (w1898:dbl)
                                n586 = Subtract(x=w1895, y=w1896) -> (x-y=w1888:dbl)
                                n587 = Absolute Value(x=w1888) -> (abs(x)=w1889:dbl)
                                n588 = Subtract(x=w1897, y=w1898) -> (x-y=w1891:dbl)
                                n589 = Greater?(x=w1889, y=w1887) -> (0:w1893:bool)
                                n590 = Absolute Value(x=w1891) -> (abs(x)=w1890:dbl)
                                n591 = Greater?(x=w1890, y=w1887) -> (0:w1892:bool)
                                n592 = Or(x=w1892, y=w1893) -> (x .or. y?=w1894:bool)
                                n593 = case shown="True" w1894 {
                                frame False {
                                }
                                frame True {
                                n594 = stacked-sequence {
                                frame #0 {
                                n595 = local read "Null array"() -> (w1906:dbl[])
                                n596 = local write "What to Check"(w1906) -> ()
                                n597 = local write "ID"(w1906) -> ()
                                n598 = local read "Current Spot #"() -> (w1908:dbl)
                                n599 = local write "Potential Collisions"(0) -> ()
                                n600 = local read "Spot Checker"() -> (w1907:T3[])
                                n601 = Index Array(array=w1907, index=w1908) -> (element=w1909:T3)
                                n602 = Wait (ms)(milliseconds to wait=100) -> ()  [unwired: 1 out]
                                n603 = Unbundle By Name(w1909) -> ("Position.x"=w1903:dbl, "Position.y"=w1904:dbl)
                                n604 = local write "Orig Y SC"(w1904) -> ()
                                n605 = local write "Orig X SC"(w1903) -> ()
                                }
                                frame #1 {
                                # "All this is a  statement checking whether the microrobot is within the area being checked using absolute value statements. The number of potential collisions gets added by 1 every time a bubble is detected within the area."
                                n606 = local read "# of Spots"() -> (w1910:dbl)
                                n607 = for {
                                N: w1910 -> [_]
                                tunnel: w1910 -> [w1915]
                                i -> [w1911]
                                n608 = local read "Selection/Group"() -> (w1914:T9[])
                                n609 = Index Array(array=w1914, index=w1911) -> (element=w1913:T9)
                                n610 = Unbundle By Name(w1913) -> ("Selected"=w1912:bool)
                                n611 = case shown="True" w1912 {
                                tunnel: w1915 -> [_ w1917]
                                tunnel: w1911 -> [_ w1916]
                                frame False {
                                }
                                frame True {
                                n612 = for {
                                N: w1917 -> [_]
                                tunnel: w1916 -> [w1918]
                                i -> [w1919]
                                n613 = local read "Selection/Group"() -> (w1923:T9[])
                                n614 = Index Array(array=w1923, index=w1919) -> (element=w1922:T9)
                                n615 = Unbundle By Name(w1922) -> ("Selected"=w1920:bool)
                                n616 = Not(x=w1920) -> (.not. x?=w1921:bool)
                                n617 = case shown="True" w1921 {
                                tunnel: w1919 -> [_ w1927]
                                tunnel: w1918 -> [_ w1926]
                                tunnel: w1918 -> [_ w1925]
                                frame False {
                                }
                                frame True {
                                n618 = local read "Spot Checker"() -> (w1944:T3[])
                                n619 = Index Array(array=w1944, index=w1927) -> (element=w1945:T3)
                                n620 = Index Array(array=w1944, index=w1926) -> (element=w1943:T3)
                                n621 = Unbundle By Name(w1943) -> ("Position.x"=w1940:dbl, "Position.y"=w1936:dbl)
                                n622 = Unbundle By Name(w1945) -> ("Position.x"=w1937:dbl, "Position.y"=w1933:dbl)
                                n623 = local read "Area+ Buffer"() -> (w1924:dbl)
                                n624 = Subtract(x=w1940, y=w1924) -> (x-y=w1941:dbl)
                                n625 = Greater Or Equal?(x=w1937, y=w1941) -> (x >= y?=w1942:bool)
                                n626 = Add(x=w1936, y=w1924) -> (x+y=w1935:dbl)
                                n627 = Subtract(x=w1936, y=w1924) -> (x-y=w1934:dbl)
                                n628 = Add(x=w1940, y=w1924) -> (x+y=w1938:dbl)
                                n629 = Less Or Equal?(x=w1933, y=w1935) -> (x <= y?=w1932:bool)
                                n630 = Greater Or Equal?(x=w1933, y=w1934) -> (x >= y?=w1931:bool)
                                n631 = Less Or Equal?(x=w1937, y=w1938) -> (x <= y?=w1939:bool)
                                n632 = And(x=w1942, y=w1939) -> (x .and. y?=w1929:bool)
                                n633 = And(x=w1932, y=w1931) -> (x .and. y?=w1930:bool)
                                n634 = And(x=w1929, y=w1930) -> (x .and. y?=w1928:bool)
                                n635 = case shown="True" w1928 {
                                tunnel: w1927 -> [_ _]
                                tunnel: w1927 -> [_ w1947]
                                tunnel: w1925 -> [_ w1946]
                                frame False {
                                }
                                frame True {
                                n636 = stacked-sequence {
                                tunnel: w1947 -> [w1948 _]
                                tunnel: w1946 -> [w1949 _]
                                frame #0 {
                                n637 = local read "Potential Collisions"() -> (w1952:dbl)
                                n638 = local read "What to Check"() -> (w1953:dbl[])
                                n639 = Insert Into Array(array=w1953, index=w1952, new element=w1948) -> (w1954:dbl[])
                                n640 = local read "ID"() -> (w1951:dbl[])
                                n641 = local write "What to Check"(w1954) -> ()
                                n642 = Insert Into Array(array=w1951, index=w1952, new element=w1949) -> (w1950:dbl[])
                                n643 = local write "ID"(w1950) -> ()
                                }
                                frame #1 {
                                n644 = local read "Potential Collisions"() -> (w1957:dbl)
                                n645 = Add(x=w1957, y=1) -> (x+y=w1955:dbl)
                                n646 = local write "Potential Collisions"(w1955) -> ()
                                }
                                }
                                }
                                }
                                }
                                }
                                }
                                }
                                }
                                }
                                }
                                frame #2 {
                                n647 = local read "Current Spot #"() -> (w1958:dbl)
                                n648 = local write "Prev Current Spot"(w1958) -> ()
                                }
                                }
                                }
                                }
                                }
                              }
                            }
                          }
                        }
                        frame #1 {
                          # "This updates the ID and Value being checked at the beginning of IDs and values being checked."
                          n649 = local read "Spot # Check"() -> (w1961:dbl)
                          n650 = local read "What to Check"() -> (w1962:dbl[])
                          n651 = local read "ID"() -> (w1963:dbl[])
                          n652 = Index Array(array=w1963, index=w1961) -> (element=w1960:dbl)
                          n653 = Index Array(array=w1962, index=w1961) -> (element=w1959:dbl)
                          n654 = local write "Value Check"(w1959) -> ()
                          n655 = local write "ID num check"(w1960) -> ()
                        }
                      }
                    }
                    frame True {
                      n656 = stacked-sequence {
                        frame #0 {
                          # "This section activate a case statement which allows us to change the area being checked. Orig X/Y SC holds the position of the area to check and changes after the bubble exits the area beig checked."
                          # "This statement controls the areas selected and finds which bubbles needs to be checked. This activates when the bubble\nmoves out of the area specified."
                          n657 = local read "# of Spots"() -> (w1983:dbl)
                          n658 = local read "Current Spot #"() -> (w1982:dbl)
                          n659 = Subtract(x=w1983, y=1) -> (x-y=w1984:dbl)
                          n660 = Equal?(x=w1982, y=w1984) -> (x = y?=w1980:bool)
                          n661 = case shown="True" w1980 {
                            tunnel: [w2043 w2046] -> w1981
                            frame True {
                              n662 = local read "# of Spots"() -> (w2044:dbl)
                              n663 = Subtract(x=w2044, y=2) -> (x-y=w2043:dbl)
                            }
                            frame False {
                              n664 = local read "# of Spots"() -> (w2045:dbl)
                              n665 = Subtract(x=w2045, y=1) -> (x-y=w2046:dbl)
                            }
                          }
                          "Maximum" <- w1981
                          n666 = local read "Spot Checker"() -> (w1979:T3[])
                          n667 = local read "Current Spot #"() -> (w1978:dbl)
                          n668 = Index Array(array=w1979, index=w1978) -> (element=w1977:T3)
                          n669 = Unbundle By Name(w1977) -> ("Position.x"=w1976:dbl, "Position.y"=w1975:dbl)
                          n670 = local read "Orig Y SC"() -> (w1973:dbl)
                          n671 = local read "Orig X SC"() -> (w1974:dbl)
                          n672 = Subtract(x=w1975, y=w1973) -> (x-y=w1970:dbl)
                          n673 = Subtract(x=w1976, y=w1974) -> (x-y=w1972:dbl)
                          n674 = Absolute Value(x=w1970) -> (abs(x)=w1969:dbl)
                          n675 = Absolute Value(x=w1972) -> (abs(x)=w1971:dbl)
                          n676 = local read "Area to check"() -> (w1965:dbl)
                          n677 = local read "Area to check"() -> (w1964:dbl)
                          n678 = Greater?(x=w1971, y=w1965) -> (0:w1968:bool)
                          n679 = Greater?(x=w1969, y=w1964) -> (0:w1967:bool)
                          n680 = Or(x=w1968, y=w1967) -> (x .or. y?=w1966:bool)
                          n681 = case shown="True" w1966 {
                            frame False {
                            }
                            frame True {
                              n682 = stacked-sequence {
                                frame #0 {
                                # "A small time delay of 100 ms is provided to allow the data to pass throguh properly."
                                n683 = Wait (ms)(milliseconds to wait=100) -> ()  [unwired: 1 out]
                                n684 = local read "Null array"() -> (→"What to Check" →"ID":dbl[])
                                n685 = local read "Spot Checker"() -> (w1991:T3[])
                                n686 = local read "Current Spot #"() -> (w1990:dbl)
                                n687 = Index Array(array=w1991, index=w1990) -> (element=w1989:T3)
                                n688 = Unbundle By Name(w1989) -> ("Position.x"=→"Orig X SC":dbl, "Position.y"=→"Orig Y SC":dbl)
                                "Potential Collisions" <- 0
                                }
                                frame #1 {
                                n689 = local read "# of Spots"() -> (w1994:dbl)
                                n690 = for {
                                N: w1994 -> [_]
                                tunnel: w1994 -> [w1999]
                                i -> [w1995]
                                n691 = local read "Selection/Group"() -> (w1998:T9[])
                                n692 = Index Array(array=w1998, index=w1995) -> (element=w1997:T9)
                                n693 = Unbundle By Name(w1997) -> ("Selected"=w1996:bool)
                                n694 = case shown="True" w1996 {
                                tunnel: w1999 -> [_ w2001]
                                tunnel: w1995 -> [_ w2000]
                                frame False {
                                }
                                frame True {
                                n695 = for {
                                N: w2001 -> [_]
                                tunnel: w2000 -> [w2002]
                                i -> [w2003]
                                n696 = local read "Selection/Group"() -> (w2007:T9[])
                                n697 = Index Array(array=w2007, index=w2003) -> (element=w2006:T9)
                                n698 = Unbundle By Name(w2006) -> ("Selected"=w2004:bool)
                                n699 = Not(x=w2004) -> (.not. x?=w2005:bool)
                                n700 = case shown="True" w2005 {
                                tunnel: w2003 -> [_ w2011]
                                tunnel: w2002 -> [_ w2010]
                                tunnel: w2002 -> [_ w2009]
                                frame False {
                                }
                                frame True {
                                n701 = local read "Spot Checker"() -> (w2028:T3[])
                                n702 = Index Array(array=w2028, index=w2011) -> (element=w2029:T3)
                                n703 = Index Array(array=w2028, index=w2010) -> (element=w2027:T3)
                                n704 = Unbundle By Name(w2027) -> ("Position.x"=w2024:dbl, "Position.y"=w2020:dbl)
                                n705 = Unbundle By Name(w2029) -> ("Position.x"=w2021:dbl, "Position.y"=w2017:dbl)
                                n706 = local read "Area+ Buffer"() -> (w2008:dbl)
                                n707 = Subtract(x=w2024, y=w2008) -> (x-y=w2025:dbl)
                                n708 = Greater Or Equal?(x=w2021, y=w2025) -> (x >= y?=w2026:bool)
                                n709 = Add(x=w2020, y=w2008) -> (x+y=w2019:dbl)
                                n710 = Subtract(x=w2020, y=w2008) -> (x-y=w2018:dbl)
                                n711 = Add(x=w2024, y=w2008) -> (x+y=w2022:dbl)
                                n712 = Less Or Equal?(x=w2017, y=w2019) -> (x <= y?=w2016:bool)
                                n713 = Greater Or Equal?(x=w2017, y=w2018) -> (x >= y?=w2015:bool)
                                n714 = Less Or Equal?(x=w2021, y=w2022) -> (x <= y?=w2023:bool)
                                n715 = And(x=w2026, y=w2023) -> (x .and. y?=w2013:bool)
                                n716 = And(x=w2016, y=w2015) -> (x .and. y?=w2014:bool)
                                n717 = And(x=w2013, y=w2014) -> (x .and. y?=w2012:bool)
                                n718 = case shown="True" w2012 {
                                tunnel: w2011 -> [_ _]
                                tunnel: w2011 -> [_ w2031]
                                tunnel: w2009 -> [_ w2030]
                                frame False {
                                }
                                frame True {
                                n719 = stacked-sequence {
                                tunnel: w2031 -> [w2032 _]
                                tunnel: w2030 -> [w2033 _]
                                frame #0 {
                                n720 = local read "Potential Collisions"() -> (w2036:dbl)
                                n721 = local read "What to Check"() -> (w2037:dbl[])
                                n722 = Insert Into Array(array=w2037, index=w2036, new element=w2032) -> (w2038:dbl[])
                                n723 = local read "ID"() -> (w2035:dbl[])
                                n724 = Insert Into Array(array=w2035, index=w2036, new element=w2033) -> (w2034:dbl[])
                                n725 = local write "What to Check"(w2038) -> ()
                                n726 = local write "ID"(w2034) -> ()
                                }
                                frame #1 {
                                n727 = local read "Potential Collisions"() -> (w2041:dbl)
                                n728 = Add(x=w2041, y=1) -> (x+y=w2039:dbl)
                                n729 = local write "Potential Collisions"(w2039) -> ()
                                }
                                }
                                }
                                }
                                }
                                }
                                }
                                }
                                }
                                }
                                }
                              }
                            }
                          }
                        }
                        frame #1 {
                          n730 = local read "# of Spots"() -> (w2050:dbl)
                          n731 = Not Equal?(x=w2050, y=1) -> (x != y?=w2048:bool)
                          n732 = case shown="True" w2048 {
                            frame False {
                            }
                            frame True {
                              n733 = stacked-sequence {
                                frame #0 {
                                n734 = local read "Potential Collisions"() -> (w2053:dbl)
                                n735 = local read "Spot # Check"() -> (w2055:dbl)
                                n736 = Subtract(x=w2053, y=1) -> (x-y=w2051:dbl)
                                n737 = Less Or Equal?(x=w2055, y=w2051) -> (x <= y?=w2054:bool)
                                n738 = case shown="False" w2054 {
                                frame False {
                                n739 = local write "Spot # Check"(0) -> ()
                                }
                                frame True {
                                }
                                }
                                }
                                frame #1 {
                                n740 = local read "What to Check"() -> (w2061:dbl[])
                                n741 = local read "ID"() -> (w2059:dbl[])
                                n742 = local read "Spot # Check"() -> (w2057:dbl)
                                n743 = Index Array(array=w2061, index=w2057) -> (element=→"Value Check":dbl)
                                n744 = Index Array(array=w2059, index=w2057) -> (element=→"ID num check":dbl)
                                }
                              }
                            }
                          }
                        }
                      }
                    }
                  }
                  n745 = local read "Potential Collisions"() -> (w1838:dbl)
                  n746 = Subtract(x=w1838, y=1) -> (x-y=w1839:dbl)
                  n747 = local read "Hit"() -> (w1856:bool)
                  n748 = Equal?(x=w1851, y=w1839) -> (x = y?=w1855:bool)
                  n749 = Or(x=w1856, y=w1855) -> (x .or. y?=w1853:bool)
                }
                n750 = for {
                  tunnel: w1828 -> [w2075] mode=indexing
                  tunnel: w1829 -> [w2072] mode=indexing
                  tunnel: [w2074] -> w1823 mode=indexing
                  tunnel: w1825 -> [w2073]
                  # "If the projected distance is greater than the\nprevious distance, then the selected spots will move. \nThis situation only occurs if the bubble is about to/crossing \nthe buffer zone of another bubble. \n\nThe selected spots will also move if none of the bubbles\nare near/crossing the buffer zone of another bubble."
                  n751 = local read "Hit"() -> (w2065:bool)
                  n752 = Unbundle By Name(w2072) -> ()  [unwired: 1 out]
                  n753 = local read "Projected Distance"() -> (w2064:dbl)
                  n754 = Unbundle(w2075) -> ("Group ID"=→"Group ID #":i32, "Selected"=w2069:bool)
                  n755 = local read "Previous Distance"() -> (w2067:dbl)
                  n756 = Not(x=w2065) -> (.not. x?=w2063:bool)
                  n757 = Greater?(x=w2064, y=w2067) -> (0:w2066:bool)
                  n758 = And(x=w2065, y=w2066) -> (x .and. y?=w2062:bool)
                  n759 = Or(x=w2063, y=w2062) -> (x .or. y?=w2068:bool)
                  n760 = And(x=w2069, y=w2068) -> (x .and. y?=w2070:bool)
                  n761 = case shown="True" w2070 {
                    tunnel: w2072 -> [w2076 w2080]
                    tunnel: [w2076 w2079] -> w2074
                    tunnel: w2073 -> [_ w2081]
                    frame False {
                      # "otherwise, leave it alone!"
                    }
                    frame True {
                      # "If the spot is selected, move it by the same amount as the mouse"
                      n762 = call "extract_position.vi"("Spot"=w2080) -> ("Position"=w2078:cluster{"x":dbl, "y":dbl, "z":dbl})
                      n763 = Add(x=w2078, y=w2081) -> (x+y=w2077:cluster{dbl, dbl, dbl})
                      n764 = call "replace_position.vi"("Position"=w2077, "Spot in"=w2080) -> ("Spot"=w2079:T3)  [unwired: 2 out]
                    }
                  }
                }
                "Spot Checker" <- w1823
                n765 = local read "Locked Current Spot"() -> (w1819:dbl)
                n766 = Index Array(array=w1823, index=w1819) -> (element=w1822:T3)
                n767 = Unbundle By Name(w1822) -> ("Position.x"=→"New X":dbl, "Position.y"=→"New Y":dbl)  [unwired: 1 out]
                n768 = Array Size(array=w1823) -> (size(s)=→"# of Spots":i32)
              }
              frame True {
                # "coordinate conversion to find the rotation and scaling done by the mouse, about the centroid of the spots"
                n769 = Subtract(x=w2083, y=w2093) -> (x-y=w2102:cluster{dbl, dbl, dbl})
                n770 = Subtract(x=w2084, y=w2093) -> (x-y=w2101:cluster{dbl, dbl, dbl})
                n771 = Unbundle(w2101) -> (w2087:dbl, w2088:dbl)  [unwired: 1 out]
                n772 = Unbundle(w2102) -> (w2092:dbl, w2091:dbl)  [unwired: 1 out]
                n773 = Re/Im To Polar(2:w2088, 3:w2087) -> (0:w2085:dbl, 1:w2086:dbl)
                n774 = Re/Im To Polar(2:w2091, 3:w2092) -> (0:w2089:dbl, 1:w2090:dbl)
                n775 = Divide(x=w2086, y=w2090) -> (x/y=w2082:dbl)
                n776 = Subtract(x=w2085, y=w2089) -> (x-y=w2094:dbl)
                n777 = Bundle(w2082, w2082, w2082) -> (w2104:cluster{dbl, dbl, dbl})  [unwired: 1 out]
                n778 = call "scale_matrix.vi"("Scale Factors"=w2104) -> ("Scale Matrix"=w2100:T10)
                n779 = call "arb_rotation_matrix.vi"("Unit Vector"=cluster{dbl, dbl, dbl} {0.0, 0.0, 1.0}, "theta"=w2094) -> ("Real Matrix"=w2099:T10)
                n780 = call-poly <vilib>:"A x B.vi"("B"=w2099, "A"=w2100) -> ("A x B"=w2095:T10)  [unwired: 1 out]
                n781 = for {
                  tunnel: w2098 -> [w2110] mode=indexing
                  tunnel: [w2109] -> w2097 mode=indexing
                  tunnel: w2096 -> [w2108] mode=indexing
                  tunnel: w2093 -> [w2106]
                  tunnel: w2095 -> [w2105]
                  n782 = Unbundle(w2108) -> ("Selected"=w2107:bool)  [unwired: 1 out]
                  n783 = case shown="True" w2107 {
                    tunnel: w2110 -> [w2111 w2115]
                    tunnel: [w2111 w2114] -> w2109
                    tunnel: w2106 -> [_ w2113]
                    tunnel: w2105 -> [_ w2112]
                    frame False {
                    }
                    frame True {
                      n784 = call "apply_matrix_transformation_to_spots.vi"("Transform centre (i.e. transform about this point)"=w2113, "Transformation Matrix (3x3)"=w2112, "Spot In"=w2115) -> ("Spot Out"=w2114:T3)  [unwired: 5 out]
                    }
                  }
                }
              }
            }
          }
        }
        "Selection/Group" <- w1787
        n785 = Unbundle By Name(w1794) -> ("Position (Image Pixels)"=w1793:cluster{"X":dbl, "Y":dbl})
        n786 = Bundle By Name(cluster=w1794, "Dragging"=TRUE, "Previous Position (Image Pixels)"=w1793, "Position (Image Pixels)"=w1792) -> (w1803:T13)
      }
      event "stop": Value Change {
        n787 = event-data() -> ()  [unwired: 1 in, 4 out]
        n788 = global read "red_tweezers_globals_INTERNAL_VOLATILE.vi" "Current Settings File"() -> (w2119:path)
        n789 = call <vilib>:"Check if File or Folder Exists.vi"("path"=w2119) -> ("file or folder exists?"=w2118:bool)  [unwired: 8 in, 2 out]
        n790 = case shown="False" w2118 {
          tunnel: [w2126 w2130] -> w2120
          frame False {
            n791 = Two Button Dialog(message="Save current settings?", 1:"Don't Save" ("F button name (\"Cancel\")"), 2:"Save As..." ("T button name (\"OK\")")) -> (T button?=w2123:bool)
            n792 = Select(t=T18."Center Button" ("Which Button?"), s=w2123, f=T18."Right Button" ("Which Button?")) -> (s? t:f=w2126:T18)
          }
          frame True {
            n793 = call <vilib>:"Three Button Dialog.vi"("Allow user to close window? (TRUE)"=TRUE, "Window Title (\"\")"="Save Settings?" ("Window Title (\"\")"), "Right Button Text (\"Cancel\")"="No" ("Right Button Text (\"Cancel\")"), "Center Button Text (\"No\")"="Save As..." ("Center Button Text (\"No\")"), "Left Button Text (\"Yes\")"="Save" ("Left Button Text (\"Yes\")"), "message"="Would you like to save the current settings? You can choose to use the current settings file or save to a new location.") -> ("Which Button?"=w2130:T18)  [unwired: 5 in]
          }
        }
        n794 = case shown="\"Center Button\"" w2120 {
          tunnel: [TRUE TRUE FALSE FALSE] -> w2117
          frame "Left Button", Default {
          }
          frame "Center Button" {
            n795 = call "File Dialog5"("prompt"="Please select a location to save the settings", "button label"="Save", "default name"="red_tweezers_settings.xml", "pattern (all files)"="*.xml" ("pattern label"), "pattern label"="XML Settings Files") -> ("selected path"=w2138:path)  [unwired: 7 in, 3 out]
            n796 = global write "red_tweezers_globals_INTERNAL_VOLATILE.vi" "Current Settings File"(w2138) -> ()
          }
          frame "Right Button" {
          }
          frame "Window Close" {
          }
        }
        n797 = global write "red_tweezers_globals_INTERNAL_VOLATILE.vi" "Save Settings On Exit"(w2117) -> ()
      }
    }
    n798 = case shown="1" "ROI points" {
      frame 0, Default {
        # "ROI point 0 is not used"
        n799 = local read "ROI Y"() -> (w173:dbl)
        "ROI new Mpy" <- w173
        n800 = local read "ROI X"() -> (w174:dbl)
        "ROI new MPx" <- w174
        n801 = Build Array(w174, w173) -> (→"ROI Point 0":T10)
      }
      frame 1 {
        n802 = local read "Object MP Y"() -> (w180:dbl)
        n803 = local read "Object MP X"() -> (w181:dbl)
        n804 = local read "ROI Y"() -> (w177:dbl)
        "ROI y1" <- w177
        n805 = local read "ROI X"() -> (w176:dbl)
        "ROI x1" <- w176
        n806 = Subtract(x=w177, y=w180) -> (x-y=→"Radius ROI y1":dbl)
        n807 = Subtract(x=w176, y=w181) -> (x-y=→"Radius ROI x1":dbl)
        n808 = Build Array(w176, w177) -> (→"ROI Point 1":T10)
      }
      frame 2 {
        n809 = local read "Object MP Y"() -> (w187:dbl)
        n810 = local read "Object MP X"() -> (w188:dbl)
        n811 = local read "ROI Y"() -> (w183:dbl)
        "ROI y2" <- w183
        n812 = local read "ROI X"() -> (w184:dbl)
        "ROI x2" <- w184
        n813 = Subtract(x=w183, y=w187) -> (x-y=→"Radius ROI y2":dbl)
        n814 = Subtract(x=w184, y=w188) -> (x-y=→"Radius ROI x2":dbl)
        n815 = Build Array(w184, w183) -> (→"ROI Point 2":T10)
      }
      frame 3 {
        n816 = local read "Object MP Y"() -> (w194:dbl)
        n817 = local read "Object MP X"() -> (w195:dbl)
        n818 = local read "ROI Y"() -> (w190:dbl)
        "ROI y3" <- w190
        n819 = local read "ROI X"() -> (w191:dbl)
        "ROI x3" <- w191
        n820 = Subtract(x=w190, y=w194) -> (x-y=→"Radius ROI y3":dbl)
        n821 = Subtract(x=w191, y=w195) -> (x-y=→"Radius ROI x3":dbl)
        n822 = Build Array(w191, w190) -> (→"ROI Point 3":T10)
      }
      frame 4 {
        n823 = local read "Object MP Y"() -> (w202:dbl)
        n824 = local read "Object MP X"() -> (w201:dbl)
        n825 = local read "ROI Y"() -> (w197:dbl)
        "ROI y4" <- w197
        n826 = local read "ROI X"() -> (w198:dbl)
        "ROI x4" <- w198
        n827 = Subtract(x=w197, y=w202) -> (x-y=→"Radius ROI y4":dbl)
        n828 = Subtract(x=w198, y=w201) -> (x-y=→"Radius ROI x4":dbl)
        n829 = Build Array(w198, w197) -> (→"ROI Point 4":T10)
      }
      frame 5 {
        n830 = local read "Object MP Y"() -> (w209:dbl)
        n831 = local read "Object MP X"() -> (w208:dbl)
        n832 = local read "ROI Y"() -> (w205:dbl)
        "ROI y5" <- w205
        n833 = local read "ROI X"() -> (w204:dbl)
        "ROI x5" <- w204
        n834 = Subtract(x=w205, y=w209) -> (x-y=→"Radius ROI y5":dbl)
        n835 = Subtract(x=w204, y=w208) -> (x-y=→"Radius ROI x5":dbl)
        n836 = Build Array(w204, w205) -> (→"ROI point 5":T10)
      }
      frame 6 {
        n837 = local read "Object MP Y"() -> (w216:dbl)
        n838 = local read "Object MP X"() -> (w215:dbl)
        n839 = local read "ROI Y"() -> (w211:dbl)
        "ROI y6" <- w211
        n840 = local read "ROI X"() -> (w212:dbl)
        "ROI x6" <- w212
        n841 = Subtract(x=w211, y=w216) -> (x-y=→"Radius ROI y6":dbl)
        n842 = Subtract(x=w212, y=w215) -> (x-y=→"Radius ROI x6":dbl)
        n843 = Build Array(w212, w211) -> (→"ROI Point 6":T10)
      }
      frame 7 {
      }
    }
    n844 = call "IMAQ Create"("Image Name"="untitled", "Image Type"=w67) -> ("New Image"=w66:T11)  [unwired: 3 in, 1 out]
    n845 = call "Vision Acquisition"() -> ("Image Out"=w65:T11)  [unwired: 24 in, 3 out]
    n846 = call "IMAQ ExtractSingleColorPlane"("Color Plane"=w64, "Image Dst"=w66, "Image Src"=w65) -> ("Image Dst Out"=w43:T11)  [unwired: 7 in, 1 out]
    n847 = case shown="False" "ROI switch" {
      tunnel: w43 -> [w219 w255]
      frame False {
        n848 = local read "Number of Matches Returned"() -> (w218:dbl)
        n849 = Add(x=w218, y=1.0 ("x+y")) -> (x+y=w220:dbl)
        n850 = for {
          N: w220 -> [_]
          tunnel: w219 -> [w224]
          i -> [w250]
          n851 = property on="Camera 3" class="ImageControl"() -> ("ROI"=w225:T27)  [unwired: 2 in, 2 out]
          n852 = Unbundle By Name(w225) -> ("Contours"=w234:T28)
          n853 = local read "Circles 2"() -> (w237:T2)
          n854 = Number To Decimal String(number=w250) -> (decimal integer string=w249:string)  [unwired: 1 in]
          n855 = Index Array(array=w237) -> (element=w254:T29)  [unwired: 1 in]
          n856 = Index Array(array=w234) -> (element=w233:T30)  [unwired: 1 in]
          n857 = Unbundle(w254) -> ("Position"=w248:cluster{"X":sgl, "Y":sgl}, "Radius"=w236:dbl)  [unwired: 1 out]
          "Radius" <- w236
          n858 = Unbundle By Name(w233) -> ("Points"=w232:i32[])
          n859 = Unbundle(w248) -> ("X"=w252:sgl, "Y"=w251:sgl)
          n860 = Subtract(x=w252, y=w236) -> (x-y=→"toplx 2":dbl)
          n861 = Add(x=w252, y=w236) -> (x+y=→"bottomrx 2":dbl)
          n862 = Add(x=w251, y=w236) -> (x+y=→"bottomry 2":dbl)
          n863 = Subtract(x=w251, y=w236) -> (x-y=→"toply 2":dbl)
          n864 = Index Array(array=w232, index #1=0 ("index"), index #2=1 ("index")) -> (element #1=w223:i32, element #2=w222:i32)
          n865 = Bundle(w223, w222) -> (w229:cluster{i32, i32})  [unwired: 1 in]
          "Specific Point 2" <- w229
          n866 = call "IMAQ Overlay Text"("Text Color (black)"=u32 1703680, "Font, Size & Style"=T14 {"Desired Font (Application)"=enum."Application Font", "[User-specified Font]"={"Font Name"="", "Size"=40, "Strikeout?"=FALSE, "Italic?"=FALSE, "Underline?"=FALSE, "Outline?"=FALSE, "Shadow?"=FALSE, "Bold?"=FALSE, "Rotation Angle"=0.0}, "Horizontal Alignment"=0, "Vertical Alignment"=0}, "String"="ROI", "Origin"=w229, "Image"=w224) -> ()  [unwired: 5 in, 2 out]
          n867 = local read "toply 2"() -> (w240:dbl)
          n868 = local read "bottomrx 2"() -> (w239:dbl)
          n869 = local read "toplx 2"() -> (w241:dbl)
          n870 = local read "bottomry 2"() -> (w238:dbl)
          n871 = local write "ROI X"(w223) -> ()
          n872 = local write "ROI Y"(w222) -> ()
          n873 = Build Array(w241, w240, w239, w238) -> (w246:dbl[])
          n874 = Array To Cluster(array=w246) -> (cluster=w253:T31)
          n875 = call "IMAQ Overlay Oval"("Bounding Rectangle"=w253, "Image"=w224) -> ("Image Out"=w247:T11)  [unwired: 8 in, 1 out]
          n876 = call "IMAQ Overlay Text"("String"=w249, "Origin"=w248, "Image"=w247) -> ("Image Out"=→"Camera 3":T11)  [unwired: 7 in, 1 out]
        }
      }
      frame True {
        # "This is the code for ROI and Object detection"
        n877 = local read "Number of Objects"() -> (w257:i32)
        n878 = Add(x=w257, y=1.0 ("x+y")) -> (x+y=w256:dbl)
        n879 = for {
          N: w256 -> [_]
          tunnel: w255 -> [w268]
          # "This part of the\ncode detects \nobeject"
          # "This is the ROI, a specific point selected"
          # "This part of the code will obtain the Midpoint"
          n880 = local read "Objects"() -> (w262:T1)
          n881 = Index Array(array=w262) -> (element=w263:T32)  [unwired: 1 in]
          n882 = property on="Camera 3" class="ImageControl"() -> ("ROI"=w267:T27)  [unwired: 2 in, 2 out]
          n883 = Unbundle(w263) -> ("Object Center"=w261:cluster{"X":sgl, "Y":sgl})  [unwired: 5 out]
          n884 = Unbundle By Name(w267) -> ("Contours"=w277:T28)
          n885 = call "IMAQ Count Objects 2"("Settings"="Settings", "Image"=w268) -> ("Number of Objects"=→"Number of Objects":i32, "Image Out"=w280:T11, "Objects"=→"Objects":T1)  [unwired: 5 in, 2 out]
          n886 = Unbundle(w261) -> ("X"=→"Object MP X":sgl, "Y"=→"Object MP Y":sgl)
          n887 = local write "Camera 3"(w280) -> ()
          n888 = Index Array(array=w277) -> (element=w276:T30)  [unwired: 1 in]
          n889 = Unbundle By Name(w276) -> ("Points"=w275:i32[])
          n890 = Index Array(array=w275, index #1=0 ("index"), index #2=1 ("index")) -> (element #1=w266:i32, element #2=w265:i32)
          "ROI X" <- w266
          "ROI Y" <- w265
          n891 = Bundle(w266, w265) -> (w272:cluster{i32, i32})  [unwired: 1 in]
          "Specific Point" <- w272
          n892 = call "IMAQ Overlay Text"("Text Color (black)"=u32 1703680, "Font, Size & Style"=T14 {"Desired Font (Application)"=enum."Application Font", "[User-specified Font]"={"Font Name"="", "Size"=40, "Strikeout?"=FALSE, "Italic?"=FALSE, "Underline?"=FALSE, "Outline?"=FALSE, "Shadow?"=FALSE, "Bold?"=FALSE, "Rotation Angle"=0.0}, "Horizontal Alignment"=0, "Vertical Alignment"=0}, "String"="ROI", "Origin"=w272, "Image"=w268) -> ()  [unwired: 5 in, 2 out]
        }
      }
    }
    n893 = call-poly "IMAQ Detect Shapes"("Circle Descriptor"="Circle Descriptor 2", "Image"=w43) -> ("Number of Matches Returned"=→"Number of Matches Returned":i32, "Circles"=→"Circles 2":T2)  [unwired: 7 in, 1 out]
    n894 = property on="Image" class="ImageControl"() -> ("ROI"=w36:T27)  [unwired: 2 in, 2 out]
    n895 = Unbundle By Name(w36) -> ("Contours"=w32:T28)
    n896 = Index Array(array=w32) -> (element=w33:T30)  [unwired: 1 in]
    n897 = Unbundle By Name(w33) -> ("Points"=w34:i32[])
    n898 = Index Array(array=w34, index #1=0 ("index")) -> (element #1=→"Numeric 3":i32, element #2=→"Numeric 2":i32)  [unwired: 1 in]
    n899 = case shown="True" "Camera Capture 2" {
      frame False {
      }
      frame True {
        n900 = local read "Circles 2"() -> (w283:T2)
        n901 = Index Array(array=w283) -> (element=w284:T29)  [unwired: 1 in]
        n902 = Index Array(array=w283) -> (element=w294:T29)  [unwired: 1 in]
        n903 = Unbundle(w284) -> ("Position"=w292:cluster{"X":sgl, "Y":sgl}, "Radius"=w285:dbl)  [unwired: 1 out]
        n904 = Unbundle(w294) -> ("Position"=w293:cluster{"X":sgl, "Y":sgl})  [unwired: 2 out]
        n905 = Unbundle(w292) -> ("X"=w290:sgl, "Y"=w291:sgl)
        n906 = Unbundle(w293) -> ("X"=→"Bubble x 2":sgl, "Y"=→"Bubble y 2":sgl)
        n907 = Subtract(x=w290, y=w285) -> (x-y=→"toplx 3":dbl)
        n908 = Add(x=w290, y=w285) -> (x+y=→"bottomrx 3":dbl)
        n909 = Add(x=w291, y=w285) -> (x+y=→"bottomry 3":dbl)
        n910 = Subtract(x=w291, y=w285) -> (x-y=→"toply 3":dbl)
      }
    }
    n911 = local read "Stop"() -> (w70:i32)
    n912 = local read "Start"() -> (w69:i32)
    n913 = Subtract(x=w70, y=w69) -> (x-y=→"Time Elapsed(ms)":i32)
    n914 = case shown="True" "Play" {
      frame False {
      }
      frame True {
        n915 = stacked-sequence {
          frame #0 {
            n916 = Tick Count (ms)() -> (millisecond timer value=→"Start":u32)
          }
          frame #1 {
            n917 = local read "ROI switch"() -> (w428:bool)
            n918 = case shown="False" w428 {
              frame True {
                # "When this is on select a new Midpoint using the ROI tool"
                n919 = case shown="True" "New location\n ROI" {
                  frame False {
                    w445 = 1e-07
                    n920 = local read "ROI Point 2"() -> (w441:T10)
                    n921 = local read "ROI Point 1"() -> (w440:T10)
                    n922 = local read "ROI Point 3"() -> (w439:T10)
                    n923 = local read "ROI Point 4"() -> (w442:T10)
                    n924 = local read "ROI point 5"() -> (w443:T10)
                    n925 = local read "ROI Point 6"() -> (w444:T10)
                    n926 = call-poly <vilib>:"Multiply.vi"("Real Scalar c"=w445, "Real Matrix A"=w440) -> ("A * c"=w437:T10)
                    n927 = call-poly <vilib>:"Multiply.vi"("Real Scalar c"=w445, "Real Matrix A"=w441) -> ("A * c"=w436:T10)
                    n928 = call-poly <vilib>:"Multiply.vi"("Real Scalar c"=w445, "Real Matrix A"=w439) -> ("A * c"=w435:T10)
                    n929 = call-poly <vilib>:"Multiply.vi"("Real Scalar c"=w445, "Real Matrix A"=w442) -> ("A * c"=w446:T10)
                    n930 = call-poly <vilib>:"Multiply.vi"("Real Scalar c"=w445, "Real Matrix A"=w443) -> ("A * c"=w447:T10)
                    n931 = call-poly <vilib>:"Multiply.vi"("Real Scalar c"=w445, "Real Matrix A"=w444) -> ("A * c"=w448:T10)
                    n932 = Build Array (concatenate) ("Build Matrix")(w437, w436, w435, w446, w447, w448) -> (w438:T10)
                    n933 = local write "NewXYArray"(w438) -> ()
                  }
                  frame True {
                    w485 = 1e-07
                    n934 = local read "Radius ROI x1"() -> (w487:dbl)
                    n935 = local read "Radius ROI x3"() -> (w468:dbl)
                    n936 = local read "Radius ROI x4"() -> (w466:dbl)
                    n937 = local read "Radius ROI y1"() -> (w486:dbl)
                    n938 = local read "Radius ROI y2"() -> (w469:dbl)
                    n939 = local read "Radius ROI y3"() -> (w467:dbl)
                    n940 = local read "Radius ROI y4"() -> (w465:dbl)
                    n941 = local read "Radius ROI y5"() -> (w463:dbl)
                    n942 = local read "Radius ROI y6"() -> (w461:dbl)
                    n943 = local read "Radius ROI x2"() -> (w470:dbl)
                    n944 = local read "ROI new MPx"() -> (w472:dbl)
                    n945 = local read "ROI new Mpy"() -> (w471:dbl)
                    n946 = local read "Radius ROI x5"() -> (w464:dbl)
                    n947 = local read "Radius ROI x6"() -> (w462:dbl)
                    n948 = Add(x=w487, y=w472) -> (x+y=w460:dbl)
                    n949 = Add(x=w486, y=w471) -> (x+y=w459:dbl)
                    n950 = Add(x=w472, y=w470) -> (x+y=w458:dbl)
                    n951 = Add(x=w471, y=w469) -> (x+y=w457:dbl)
                    n952 = Add(x=w472, y=w468) -> (x+y=w456:dbl)
                    n953 = Add(x=w471, y=w467) -> (x+y=w455:dbl)
                    n954 = Add(x=w472, y=w466) -> (x+y=w454:dbl)
                    n955 = Add(x=w471, y=w465) -> (x+y=w453:dbl)
                    n956 = Add(x=w472, y=w464) -> (x+y=w452:dbl)
                    n957 = Add(x=w463, y=w471) -> (x+y=w451:dbl)
                    n958 = Add(x=w472, y=w462) -> (x+y=w450:dbl)
                    n959 = Add(x=w461, y=w471) -> (x+y=w449:dbl)
                    n960 = Build Array(w460, w459) -> (w484:T10)
                    n961 = Build Array(w458, w457) -> (w481:T10)
                    n962 = Build Array(w456, w455) -> (w480:T10)
                    n963 = Build Array(w454, w453) -> (w479:T10)
                    n964 = Build Array(w452, w451) -> (w478:T10)
                    n965 = Build Array(w450, w449) -> (w477:T10)
                    n966 = call-poly <vilib>:"Multiply.vi"("Real Scalar c"=w485, "Real Matrix A"=w484) -> ("A * c"=w483:T10)
                    n967 = call-poly <vilib>:"Multiply.vi"("Real Scalar c"=w485, "Real Matrix A"=w481) -> ("A * c"=w482:T10)
                    n968 = call-poly <vilib>:"Multiply.vi"("Real Scalar c"=w485, "Real Matrix A"=w480) -> ("A * c"=w476:T10)
                    n969 = call-poly <vilib>:"Multiply.vi"("Real Scalar c"=w485, "Real Matrix A"=w479) -> ("A * c"=w475:T10)
                    n970 = call-poly <vilib>:"Multiply.vi"("Real Scalar c"=w485, "Real Matrix A"=w478) -> ("A * c"=w474:T10)
                    n971 = call-poly <vilib>:"Multiply.vi"("Real Scalar c"=w485, "Real Matrix A"=w477) -> ("A * c"=w473:T10)
                    n972 = Build Array (concatenate) ("Build Matrix")(w483, w482, w476, w475, w474, w473) -> (w488:T10)
                    n973 = local write "NewXYArray"(w488) -> ()
                  }
                }
              }
              frame False {
                n974 = case shown="False" "Input New \nObject Location" {
                  frame True {
                    n975 = local read "# of pairs"() -> (w492:dbl)
                    n976 = Multiply(x=w492, y=1e-07) -> (x*y=w490:dbl)
                    n977 = local read "Radius"() -> (w494:dbl)
                    n978 = Add(x=w494, y=w490) -> (x+y=w493:dbl)
                    n979 = local read "New Center X"() -> (w506:dbl)
                    n980 = local read "# of pairs"() -> (w509:dbl)
                    n981 = Add(x=w506, y=w493) -> (x+y=w512:dbl)
                    n982 = local read "New Center Y"() -> (w510:dbl)
                    n983 = Multiply(x=w509, y=2.0) -> (x*y=w507:dbl)
                    n984 = Multiply(x=w512, y=1e-07) -> (x*y=w505:dbl)
                    n985 = Initialize Array(w505, w507) -> (w503:dbl[])
                    n986 = Multiply(x=w510, y=1e-07) -> (x*y=w504:dbl)
                    n987 = local read "Delta x"() -> (w502:dbl[])
                    n988 = local read "Delta y"() -> (w501:dbl[])
                    n989 = Initialize Array(w504, w507) -> (w500:dbl[])
                    n990 = for {
                      tunnel: w501 -> [w521] mode=indexing
                      tunnel: w500 -> [w520] mode=indexing
                      tunnel: [w519] -> w497 mode=indexing
                      n991 = Add(x=w520, y=w521) -> (x+y=w519:dbl)
                    }
                    n992 = for {
                      tunnel: w503 -> [w518] mode=indexing
                      tunnel: w502 -> [w517] mode=indexing
                      tunnel: [w516] -> w499 mode=indexing
                      n993 = Subtract(x=w518, y=w517) -> (x-y=w516:dbl)
                    }
                    n994 = for {
                      tunnel: w500 -> [w524] mode=indexing
                      tunnel: w501 -> [w523] mode=indexing
                      tunnel: [w522] -> w498 mode=indexing
                      n995 = Subtract(x=w524, y=w523) -> (x-y=w522:dbl)
                    }
                    n996 = Build Array(w499, w497) -> (w496:T10)
                    n997 = Build Array(w499, w498) -> (w495:T10)
                    n998 = Build Array(w505, w504) -> (w515:T10)
                    n999 = Build Array (concatenate)(w515, w496, w495) -> (w514:T10)
                    n1000 = local write "NewXYArray"(w514) -> ()
                  }
                  frame False {
                    # "array of bubbles"
                    n1001 = Square Root(x=3) -> (sqrt(x)=w542:dbl)
                    n1002 = Negate(x=w542) -> (-x=w541:dbl)
                    n1003 = Subtract(x=w542, y=2) -> (x-y=w543:dbl)
                    n1004 = local read "bottomry 2"() -> (w562:dbl)
                    n1005 = Divide(x=w543, y=w541) -> (x/y=w536:dbl)
                    n1006 = local read "toply 2"() -> (w563:dbl)
                    n1007 = local read "Radius"() -> (w560:dbl)
                    n1008 = local read "Max Number \nof Bubbles"() -> (w530:dbl)
                    n1009 = Subtract(x=w563, y=w562) -> (x-y=w531:dbl)
                    n1010 = Multiply(x=w560, y=1e-07) -> (x*y=w527:dbl)
                    "Radius" <- w527
                    n1011 = Divide(x=99, y=100) -> (x/y=w537:dbl)
                    n1012 = case shown="Default" w530 {
                      tunnel: [1 2 3 4 5 6 0] -> w525
                      frame 3 {
                      }
                      frame 4, 5 {
                      }
                      frame 6, 7 {
                      }
                      frame 8, 9 {
                      }
                      frame 10, 11 {
                      }
                      frame 12 {
                      }
                      frame Default {
                      }
                    }
                    "# of pairs" <- w525
                    n1013 = Multiply(x=w536, y=w537) -> (x*y=w535:dbl)
                    n1014 = Divide(x=w531, y=2.0) -> (x/y=w552:dbl)
                    n1015 = local read "bottomrx 2"() -> (w528:dbl)
                    n1016 = local read "bottomry 2"() -> (w529:dbl)
                    n1017 = Multiply(x=w527, y=w535) -> (x*y=w526:dbl)
                    "Caging Radius" <- w526
                    n1018 = Add(x=w529, y=w552) -> (x+y=w553:dbl)
                    n1019 = Multiply(x=w528, y=1e-07) -> (x*y=w546:dbl)
                    n1020 = Add(x=w527, y=w526) -> (x+y=w547:dbl)
                    n1021 = Add(x=w526, y=w546) -> (x+y=w545:dbl)
                    n1022 = Multiply(x=w553, y=1e-07) -> (x*y=w551:dbl)
                    n1023 = for {
                      N: w525 -> [_]
                      tunnel: w530 -> [w581]
                      tunnel: w547 -> [w580]
                      tunnel: w551 -> [w579]
                      tunnel: [w578] -> w550 mode=indexing
                      tunnel: [w577] -> w549 mode=indexing
                      tunnel: [w576] -> w548 mode=indexing
                      tunnel: [w574] -> w533 mode=indexing
                      tunnel: [w573] -> w534 mode=indexing
                      tunnel: w545 -> [w572]
                      i -> [w575]
                      w590 = 2.0
                      n1024 = Divide(x=360, y=w581) -> (x/y=w596:dbl)
                      n1025 = Add(x=1, y=w575) -> (x+y=w594:i32)
                      n1026 = Multiply(x=w596, y=w594) -> (x*y=w589:dbl)
                      n1027 = expression code="(x/180.0)*pi" ("degrees to radians")(w589) -> (w588:dbl)
                      n1028 = Subtract(x=180, y=w589) -> (x-y=w597:dbl)
                      n1029 = Square(x=w580) -> (x^2=w592:dbl)
                      n1030 = Cosine(x=w588) -> (cos(x)=w587:dbl)
                      n1031 = Divide(x=w597, y=w590) -> (x/y=w585:dbl)
                      n1032 = Multiply(x=w590, y=w592) -> (x*y=w593:dbl)
                      n1033 = Compound Arithmetic op=MULTIPLY(w590, w587, w592) -> (w591:dbl)
                      n1034 = expression code="(x/180.0)*pi" ("degrees to radians")(w585) -> (w586:dbl)
                      n1035 = Subtract(x=w593, y=w591) -> (x-y=w583:dbl)
                      n1036 = Sine(x=w586) -> (sin(x)=w582:dbl)
                      n1037 = Cosine(x=w586) -> (cos(x)=w584:dbl)
                      n1038 = Square Root(x=w583) -> (sqrt(x)=w571:dbl)
                      n1039 = Multiply(x=w582, y=w571) -> (x*y=w574:dbl)
                      n1040 = Multiply(x=w584, y=w571) -> (x*y=w573:dbl)
                      n1041 = Add(x=w579, y=w574) -> (x+y=w577:dbl)
                      n1042 = Subtract(x=w579, y=w574) -> (x-y=w578:dbl)
                      n1043 = Subtract(x=w572, y=w573) -> (x-y=w576:dbl)
                    }
                    "Delta y" <- w533
                    "Delta x" <- w534
                    n1044 = Build Array(w548, w549) -> (w556:T10)
                    n1045 = Build Array(w545, w551) -> (w557:T10)
                    n1046 = Build Array(w548, w550) -> (w555:T10)
                    n1047 = Build Array (concatenate) ("Build Matrix")(w557, w556, w555) -> (→"NewXYArray":T10)
                  }
                }
              }
            }
            n1048 = local write "Max Number \nof Bubbles"("Max Number \nof Bubbles") -> ()
            n1049 = local write "LCS"("LCS") -> ()
            n1050 = local write "Rates"("Rates") -> ()
            n1051 = local write "How Many Frames?"("Number of \nPlanned\nSequence Frames") -> ()
            "Initiate Creation" <- 1.0
          }
          frame #2 {
            n1052 = local read "NewXYArray"() -> (w603:dbl[][])
            n1053 = Array Size(array=w603) -> (size(s)=w602:i32[])
            n1054 = Index Array(array=w602, index=0) -> (element=w600:i32)
            "NewXYArraySize" <- w600
            n1055 = for {
              N: w600 -> [w605]
              i -> [w606]
              stop <- w604 stop-if-true
              n1056 = stacked-sequence {
                tunnel: w606 -> [w608 _]
                tunnel: w605 -> [w607 _]
                tunnel: [_ w611] -> w604
                frame #0 {
                  n1057 = local write "Locked Current Spot"(w608) -> ()
                  n1058 = local write "# of Spots"(w607) -> ()
                  n1059 = local write "Rates"(1) -> ()
                  n1060 = local write "LCS"(0) -> ()
                }
                frame #1 {
                  n1061 = local read "Insert"() -> (w611:bool)
                  n1062 = local write "Insert"(TRUE) -> ()
                }
              }
            }
          }
        }
      }
    }
    n1063 = local read "toplx 2"() -> (w53:dbl)
    n1064 = local read "bottomrx 2"() -> (w54:dbl)
    n1065 = Subtract(x=w53, y=w54) -> (x-y=w56:dbl)
    n1066 = local read "toplx 2"() -> (w58:dbl)
    n1067 = Absolute Value(x=w56) -> (abs(x)=w57:dbl)
    n1068 = Divide(x=w57, y=2.0) -> (x/y=w45:dbl)
    n1069 = Add(x=w45, y=w58) -> (x+y=→"Center X":dbl)
    n1070 = local write "New Center X"("New Center X") -> ()
    n1071 = local read "bottomry 2"() -> (w52:dbl)
    n1072 = local read "toply 2"() -> (w51:dbl)
    n1073 = Subtract(x=w52, y=w51) -> (x-y=w50:dbl)
    n1074 = local write "New Center Y"("New Center Y") -> ()
    n1075 = Absolute Value(x=w50) -> (abs(x)=w49:dbl)
    n1076 = local read "toply 2"() -> (w47:dbl)
    n1077 = Divide(x=w49, y=2.0) -> (x/y=w44:dbl)
    n1078 = Add(x=w44, y=w47) -> (x+y=→"Center Y":dbl)
    n1079 = case shown="True" "Lock Current Spot" {
      frame False {
      }
      frame True {
        n1080 = global read "red_tweezers_globals.vi" "Spots"() -> (w690:T3[])
        n1081 = local read "Current Spot #"() -> (w691:dbl)
        "Locked Current Spot" <- w691
        n1082 = Index Array(array=w690, index=w691) -> (element=w692:T3)
        n1083 = Unbundle By Name(w692) -> ("Position.x"=→"LCS X":dbl, "Position.y"=→"LCS Y":dbl)
        n1084 = local write "LCS"(0) -> ()
      }
    }
    n1085 = local read "Rates"() -> (w75:dbl)
    n1086 = Equal?(x=w75, y=1.0) -> (x = y?=w73:bool)
    n1087 = case shown="True" w73 {
      frame False {
      }
      frame True {
        n1088 = stacked-sequence {
          frame #0 {
            n1089 = local read "Number of \nPlanned\nSequence Frames"() -> (w376:dbl)
            n1090 = local read "Tab Control"() -> (w377:enum32{"Line", "Arc"})
            n1091 = case shown="\"Line\"" w377 {
              tunnel: w376 -> [w378 w397]
              frame "Arc" {
                n1092 = stacked-sequence {
                  tunnel: w378 -> [_ w391 _]
                  frame #0 {
                    n1093 = expression code="(x/180.0)*pi" "degrees to radians"("Theta") -> (→"Radians":dbl)
                    n1094 = local read "Radians"() -> (w390:dbl)
                    n1095 = local read "Original Y"() -> (w384:dbl)
                    n1096 = local read "Original X"() -> (w382:dbl)
                    n1097 = Cosine(x=w390) -> (cos(x)=w379:dbl)
                    n1098 = Sine(x=w390) -> (sin(x)=w381:dbl)
                    n1099 = Multiply(x=w379, y="Radius X") -> (x*y=w383:dbl)
                    n1100 = Multiply(x="Radius X", y=w381) -> (x*y=w385:dbl)
                    n1101 = Subtract(x=w382, y=w383) -> (x-y=→"Center X":dbl)
                    n1102 = Subtract(x=w384, y=w385) -> (x-y=→"Center Y":dbl)
                  }
                  frame #1 {
                    n1103 = local read "Radians"() -> (w395:dbl)
                    n1104 = Subtract(x=w391, y=1) -> (x-y=w393:dbl)
                    n1105 = Divide(x=w395, y=w393) -> (x/y=→"Degree Rate":dbl)
                  }
                  frame #2 {
                  }
                }
              }
              frame "Line" {
                n1106 = local read "Max Number \nof Bubbles"() -> (w396:dbl)
                n1107 = for {
                  N: w396 -> [_]
                  tunnel: w397 -> [w399]
                  i -> [w398]
                  n1108 = stacked-sequence {
                    tunnel: w399 -> [_ w417]
                    tunnel: w398 -> [w403 w414]
                    frame #0 {
                      n1109 = local read "NewXYArray"() -> (w409:dbl[][])
                      n1110 = Index Array(array=w409, index (row)=w403) -> (element=w408:dbl[])  [unwired: 1 in]
                      n1111 = Array To Cluster(array=w408) -> (cluster=w407:T33)
                      n1112 = global read "red_tweezers_globals.vi" "Spots"() -> (w404:T3[])
                      n1113 = Unbundle By Name(w407) -> ("NewXYArray[0]"=w406:dbl, "NewXYArray[1]"=w405:dbl)
                      n1114 = Index Array(array=w404, index=w403) -> (element=w402:T3)
                      n1115 = local write "New Y"(w405) -> ()
                      n1116 = local write "New X"(w406) -> ()
                      n1117 = Unbundle By Name(w402) -> ("Position.x"=w401:dbl, "Position.y"=w400:dbl)
                      n1118 = local write "Original X"(w401) -> ()
                      n1119 = local write "Original Y"(w400) -> ()
                    }
                    frame #1 {
                      n1120 = local read "Original X"() -> (w418:dbl)
                      n1121 = local read "Original Y"() -> (w420:dbl)
                      n1122 = Subtract(x=w417, y=1) -> (x-y=w424:dbl)
                      n1123 = local read "New Y"() -> (w421:dbl)
                      n1124 = local read "New X"() -> (w419:dbl)
                      n1125 = Subtract(x=w420, y=w421) -> (x-y=w423:dbl)
                      n1126 = Subtract(x=w418, y=w419) -> (x-y=w422:dbl)
                      n1127 = Divide(x=w423, y=w424) -> (x/y=w412:dbl)
                      "Y Rate" <- w412
                      n1128 = Divide(x=w422, y=w424) -> (x/y=w413:dbl)
                      "X Rate" <- w413
                      n1129 = Bundle(w413, w412) -> (w411:cluster{dbl, dbl})  [unwired: 1 in]
                      n1130 = local read "NewXYRates"() -> (w415:dbl[][])
                      n1131 = Cluster To Array(cluster=w411) -> (array=w410:dbl[])
                      n1132 = Insert Into Array(array=w415, index (row)=w414, new element=w410) -> (w416:dbl[][])  [unwired: 1 in]
                      n1133 = local write "NewXYRates"(w416) -> ()
                    }
                  }
                }
              }
            }
          }
          frame #1 {
            n1134 = local write "Rates"(0) -> ()
          }
        }
      }
    }
    n1135 = case shown="True" "Mark Original Position" {
      frame False {
      }
      frame True {
        w693 = TRUE
        n1136 = local write "Mark Original Position"(FALSE) -> ()
        n1137 = local read "New X"() -> (→"Original X":dbl)
        n1138 = local read "New Y"() -> (→"Original Y":dbl)
        "MOP pressed After" <- w693
        "MOP pressed" <- w693
      }
    }
    n1139 = local read "Sequence Instances"() -> (w131:dbl)
    n1140 = case shown="True" w150 {
      tunnel: w156 -> [_ w759]
      frame False {
      }
      frame True {
        n1141 = global write "red_tweezers_globals_INTERNAL.vi" "Image Overlay (extras from control loop)"(w759) -> ()
      }
    }
    n1142 = local read "Counter"() -> (w130:dbl)
    n1143 = call "red_tweezers_UNDO.vi"("Force Save"=w152, "This change is inconsequential (don't save it)"=w153, "Selection/Group"=w154, "Spots"=w155) -> ()  [unwired: 6 in, 2 out]
    n1144 = call "sync_with_globals.vi"("Selection/Group"=w154, "Spots"=w155) -> ("Selection/Group 2"=w166:T9[], "Spots 2"=w117:T3[])  [unwired: 4 in]
    n1145 = local read "Sequence Storer"() -> (w126:T3[][])
    n1146 = local read "Sequence On?"() -> (w129:bool)
    n1147 = local read "Sequence On?"() -> (w144:bool)
    n1148 = call "SequenceControl.vi"("Sequence On? 2"=w129, "Counter 2"=w130, "Sequence Instances 2"=w131, "Sequence Storer"=w126) -> ("Time per Frame (ms) 2"=w124:dbl, "Sequence Order 2"=w127:dbl, "Reset 2"=w128:bool, "Sequence Storer 2"=w139:T3[][], "Clearance Button 2"=w138:bool, "Manual Edit 2"=w137:bool, "Save State 2"=w136:bool, "Play Sequence 2"=w133:bool, "Bubble ID to Empty 2"=w132:dbl, "Manual Sequence 2"=w134:bool, "Edit Sequence Mode 2"=w135:bool)  [unwired: 1 in]
    n1149 = local write "Play Sequence"(w133) -> ()
    n1150 = local write "Bubble ID to Empty"(w132) -> ()
    n1151 = local write "Manual Sequence"(w134) -> ()
    n1152 = local write "Reset"(w128) -> ()
    n1153 = local write "Edit Sequence Mode"(w135) -> ()
    n1154 = local write "Clearance Button"(w138) -> ()
    n1155 = local write "Sequence Storer"(w139) -> ()
    n1156 = local write "Save State"(w136) -> ()
    n1157 = local write "Manual Edit"(w137) -> ()
    n1158 = Or(x=w144, y="Manual Sequence") -> (x .or. y?=w143:bool)
    n1159 = local write "Time per Frame (ms)"(w124) -> ()
    n1160 = feedback #10() -> (w171:T34)  [unwired: 1 out]
    n1161 = call "Smoothed Frame Rate.vi"("Feedback In"=w171) -> ("Feedback Out"=w170:T34, "Frame Rate"=→"Interface Frame Rate":dbl)  [unwired: 1 in, 4 out]
    n1162 = feedback-in #10(w170) -> ()
    n1163 = local write "Sequence Order"(w127) -> ()
    n1164 = Not(x=w120) -> (.not. x?=w121:bool)
    n1165 = Not(x="Output to SLM") -> (.not. x?=w122:bool)
    n1166 = case shown="True" w143 {
      tunnel: [w729 w734] -> w147
      tunnel: w117 -> [w728 _]
      frame False {
        n1167 = Or(x="Manual Edit", y="Edit Sequence Mode") -> (x .or. y?=w727:bool)
        n1168 = case shown="False" w727 {
          tunnel: w728 -> [w730 _]
          tunnel: [w730 w731] -> w729
          frame False {
          }
          frame True {
            n1169 = local read "Sequence Order"() -> (w732:dbl)
            n1170 = local read "Sequence Storer"() -> (w733:T3[][])
            n1171 = Index Array(array=w733, index (row)=w732) -> (element=w731:T3[])  [unwired: 1 in]
          }
        }
      }
      frame True {
        n1172 = stacked-sequence {
          tunnel: [w736 _] -> w734
          frame #0 {
            n1173 = local read "Counter"() -> (w737:dbl)
            n1174 = local read "Sequence Storer"() -> (w738:T3[][])
            n1175 = Index Array(array=w738, index (row)=w737) -> (element=w736:T3[])  [unwired: 1 in]
            n1176 = Wait (ms)(milliseconds to wait="Time per Frame (ms)") -> ()  [unwired: 1 out]
          }
          frame #1 {
            n1177 = local read "Sequence Instances"() -> (w740:dbl)
            n1178 = local read "Counter"() -> (w743:dbl)
            n1179 = Subtract(x=w740, y=1) -> (x-y=w741:dbl)
            n1180 = Equal?(x=w743, y=w741) -> (x = y?=w742:bool)
            n1181 = case shown="True" w742 {
              frame False {
                n1182 = local read "Counter"() -> (w746:dbl)
                n1183 = Add(x=w746, y=1) -> (x+y=→"Counter":dbl)
              }
              frame True {
                w747 = FALSE
                n1184 = local write "Counter"(0) -> ()
                n1185 = local write "Play Sequence"(w747) -> ()
                n1186 = local write "Sequence On?"(w747) -> ()
              }
            }
          }
        }
      }
    }
    n1187 = case shown="True" "Save State" {
      tunnel: w117 -> [_ w750]
      frame False {
      }
      frame True {
        n1188 = local write "Save State"(FALSE) -> ()
        n1189 = stacked-sequence {
          tunnel: w750 -> [w751 _]
          frame #0 {
            "Spot Storage" <- w751
          }
          frame #1 {
            n1190 = local read "Spot Storage"() -> (w757:T3[])
            n1191 = Replace Array Subset(array="Sequence Storer", new element=w757, index (row)="Sequence Order") -> (w755:T3[][])  [unwired: 1 in]
            n1192 = Array Size(array=w755) -> (size(s)=w754:i32[])
            n1193 = local write "Sequence Storer"(w755) -> ()
            n1194 = Index Array(array=w754, index=0) -> (element=→"Sequence Instances":i32)
          }
        }
      }
    }
    n1195 = case shown="True" "Clearance Button" {
      frame False {
      }
      frame True {
        # "This is the Bubble ID to Empty tool- this \"deletes\" the bubble in a sequence."
        n1196 = local read "Sequence Order"() -> (w720:dbl)
        n1197 = local read "Sequence Storer"() -> (w721:T3[][])
        n1198 = Replace Array Subset(array=w721, new element=T15 {"Position"={"x"=nan, "y"=nan, "z"=nan}, "Intensity"=1.0, "Vortex Charge"=1, "Phase"=1.0, "NA Position"={"x"=0.0, "y"=0.0, "r"=1.0}, "Line Trapping"={"Vector"={"x"=0.0, "y"=0.0, "z"=0.0}, "Phase Gradient"=0.0}, "Amplitude Correction"=0.0} ("Cluster"), index (row)=w720, index (col)="Bubble ID to Empty") -> (w717:T3[][])
        n1199 = local write "Sequence Storer"(w717) -> ()
      }
    }
    n1200 = case shown="True" "Save" {
      frame False {
      }
      frame True {
        n1201 = local read "Sequence Storer"() -> (w686:T3[][])
        n1202 = call "SequenceSaver.vi"("Sequence Storer"=w686) -> ()  [unwired: 10 in, 1 out]
      }
    }
    n1203 = And(x=w122, y=w121) -> (x .and. y?=w125:bool)
    n1204 = case shown="True" "Load" {
      frame False {
      }
      frame True {
        n1205 = call "SequenceSaver.vi"() -> ("Sequence Storer 2"=w685:T3[][])  [unwired: 11 in]
        n1206 = local write "Sequence Storer"(w685) -> ()
      }
    }
    n1207 = local read "Initiate Creation"() -> (w78:dbl)
    n1208 = case shown="True" w125 {
      tunnel: w117 -> [w2147 _]
      frame False {
        n1209 = call "UDP Sender generic_2.vi"("Spots"=w2147) -> ()  [unwired: 2 in, 1 out]
      }
      frame True {
      }
    }
    n1210 = case shown="True" "Reset" {
      frame False {
      }
      frame True {
        n1211 = local write "Counter"(0) -> ()
      }
    }
    n1212 = case shown="True" "Add Additional Frames" {
      frame False {
      }
      frame True {
        # "This adds additional frames to the sequence."
        n1213 = for {
          N: "Additional Frames Wanted" -> [_]
          i -> [w699]
          n1214 = local read "Max Number \nof Bubbles"() -> (w703:dbl)
          n1215 = Add(x=1, y=w699) -> (x+y=w700:i32)
          n1216 = Add(x="Frame Location", y=w700) -> (x+y=w701:dbl)
          n1217 = Initialize Array(T15 {"Position"={"x"=nan, "y"=nan, "z"=nan}, "Intensity"=1.0, "Vortex Charge"=1, "Phase"=1.0, "NA Position"={"x"=0.0, "y"=0.0, "r"=1.0}, "Line Trapping"={"Vector"={"x"=0.0, "y"=0.0, "z"=0.0}, "Phase Gradient"=0.0}, "Amplitude Correction"=0.0} ("Cluster"), w703) -> (w704:T35)
          n1218 = local read "Sequence Storer"() -> (w705:T3[][])
          n1219 = Insert Into Array(array=w705, index (row)=w701, new element=w704) -> (w706:T3[][])  [unwired: 1 in]
          n1220 = local write "Sequence Storer"(w706) -> ()
        }
      }
    }
    n1221 = case shown="1" w78 {
      frame 0, Default {
      }
      frame 1 {
        # "This create the array needed for a sequential\narray."
        n1222 = local read "Number of \nPlanned\nSequence Frames"() -> (w710:dbl)
        n1223 = local read "Max Number \nof Bubbles"() -> (w709:dbl)
        n1224 = for {
          N: w710 -> [_]
          tunnel: w709 -> [w711]
          i -> [w714]
          n1225 = Initialize Array(T15 {"Position"={"x"=nan, "y"=nan, "z"=nan}, "Intensity"=1.0, "Vortex Charge"=1, "Phase"=1.0, "NA Position"={"x"=0.0, "y"=0.0, "r"=1.0}, "Line Trapping"={"Vector"={"x"=0.0, "y"=0.0, "z"=0.0}, "Phase Gradient"=0.0}, "Amplitude Correction"=0.0} ("Cluster"), w711) -> (w712:T35)
          n1226 = local read "Sequence Storer"() -> (w715:T3[][])
          n1227 = Insert Into Array(array=w715, index (row)=w714, new element=w712) -> (w716:T3[][])  [unwired: 1 in]
          n1228 = local write "Sequence Storer"(w716) -> ()
        }
        n1229 = local write "Initiate Creation"(0) -> ()
      }
    }
    n1230 = case shown="False" "Play Sequence" {
      frame False {
        n1231 = local write "Sequence On?"(FALSE) -> ()
      }
      frame True {
        "Sequence On?" <- TRUE
      }
    }
    n1232 = local read "Current Spot #"() -> (w100:dbl)
    n1233 = local read "Selection/Group"() -> (w101:T9[])
    n1234 = local read "# of Spots"() -> (w116:dbl)
    n1235 = Not Equal?(x=w100, y=-1) -> (x != y?=w102:bool)
    n1236 = local read "spots selected 2"() -> (w90:i32)
    n1237 = Index Array(array=w101, index=w100) -> (element=w99:T9)
    n1238 = Unbundle By Name(w99) -> ("Selected"=w98:bool)
    n1239 = local read "spots selected"() -> (w91:i32)
    n1240 = Not(x=w98) -> (.not. x?=w97:bool)
    n1241 = And(x=w97, y=w102) -> (x .and. y?=w92:bool)
    n1242 = Less?(x=w91, y=w90) -> (x < y?=w88:bool)
    n1243 = case shown="True" "Insert" {
      tunnel: w117 -> [_ w296]
      tunnel: w116 -> [_ w295]
      frame False {
      }
      frame True {
        n1244 = for {
          N: w295 -> [_]
          tunnel: w296 -> [w298]
          i -> [w297]
          n1245 = stacked-sequence {
            tunnel: w298 -> [w300 w305 _]
            tunnel: w297 -> [_ w301 _]
            frame #0 {
              n1246 = local read "Start at Which Frame?"() -> (→"Num":dbl)
              "Spot Storage 2" <- w300
            }
            frame #1 {
              n1247 = local read "Selection/Group"() -> (w304:T9[])
              n1248 = Index Array(array=w304, index=w301) -> (element=w303:T9)
              n1249 = Unbundle By Name(w303) -> ("Selected"=w302:bool)
              n1250 = case shown="True" w302 {
                tunnel: w305 -> [_ _]
                frame False {
                }
                frame True {
                  n1251 = stacked-sequence {
                    frame #0 {
                      n1252 = case shown="\"Arc\"" "Tab Control" {
                        frame "Arc" {
                          n1253 = local read "How Many Frames?"() -> (w309:dbl)
                          n1254 = Subtract(x=w309, y=1) -> (x-y=w307:dbl)
                          n1255 = for {
                            N: w309 -> [_]
                            tunnel: w307 -> [w310]
                            i -> [w312]
                            # "What is this ^\n\nFor # of sequence\nframes, don't worry\nabout it"
                            # "How to make position x and y?\nIt's called a cluster, inser the new position to Position.x and Position.y"
                            n1256 = Equal?(x=w310, y=w312) -> (x = y?=w311:bool)
                            n1257 = case shown="True" w311 {
                              tunnel: [w335 w344] -> w314
                              tunnel: [w334 w343] -> w313
                              tunnel: w312 -> [w331 _]
                              frame False {
                                # "calculating new position"
                                n1258 = local read "Degree Rate"() -> (w333:dbl)
                                n1259 = Multiply(x=w333, y=w331) -> (x*y=w332:dbl)
                                n1260 = Cosine(x=w332) -> (cos(x)=w341:dbl)
                                n1261 = Sine(x=w332) -> (sin(x)=w342:dbl)
                                n1262 = local read "Radius X"() -> (w340:dbl)
                                n1263 = Multiply(x=w340, y=w342) -> (x*y=w339:dbl)
                                n1264 = Multiply(x=w341, y=w340) -> (x*y=w338:dbl)
                                n1265 = local read "Center X"() -> (w337:dbl)
                                n1266 = local read "Center Y"() -> (w336:dbl)
                                n1267 = Add(x=w337, y=w338) -> (x+y=w335:dbl)
                                n1268 = Add(x=w336, y=w339) -> (x+y=w334:dbl)
                              }
                              frame True {
                                n1269 = global read "red_tweezers_globals.vi" "Spots"() -> (w347:T3[])
                                n1270 = local read "Numeric"() -> (w346:dbl)
                                n1271 = Index Array(array=w347, index=w346) -> (element=w345:T3)
                                n1272 = Unbundle By Name(w345) -> ("Position.x"=w344:dbl, "Position.y"=w343:dbl)
                              }
                            }
                            n1273 = local read "Spot Storage 2"() -> (w330:T3[])
                            n1274 = local read "Numeric"() -> (w329:dbl)
                            n1275 = Index Array(array=w330, index=w329) -> (element=w316:T3)
                            n1276 = local read "Start at Which Frame?"() -> (w318:dbl)
                            n1277 = Bundle By Name(cluster=w316, "Position.x"=w314, "Position.y"=w313) -> (w315:T3)
                            n1278 = local read "How Many Frames?"() -> (w317:dbl)
                            n1279 = Subtract(x=w318, y=w312) -> (x-y=w327:dbl)
                            n1280 = local read "Sequence Storer"() -> (w328:T3[][])
                            n1281 = local read "Numeric"() -> (w323:dbl)
                            n1282 = Add(x=w327, y=w317) -> (x+y=w326:dbl)
                            n1283 = Subtract(x=w326, y=1) -> (x-y=w324:dbl)
                            n1284 = Replace Array Subset(array=w328, new element=w315, index (row)=w324, index (col)=w323) -> (w322:T3[][])
                            n1285 = Array Size(array=w322) -> (size(s)=w321:i32[])
                            n1286 = local write "Sequence Storer"(w322) -> ()
                            n1287 = Index Array(array=w321, index=0) -> (element=w319:i32)
                            n1288 = local write "Sequence Instances"(w319) -> ()
                          }
                        }
                        frame "Line" {
                          # "This is the automatic sequence generator which allows for the creation of the sequence. This calculates the LAST coordinates of each bubble first\nbefore going for the first few coordinates of the sequence."
                          n1289 = local read "How Many Frames?"() -> (w348:dbl)
                          n1290 = for {
                            N: w348 -> [_]
                            i -> [w356]
                            # "For why do we multiply?"
                            n1291 = local read "Spot Storage 2"() -> (w366:T3[])
                            n1292 = local read "Numeric"() -> (w353:dbl)
                            n1293 = local read "NewXYRates"() -> (w354:dbl[][])
                            n1294 = Index Array(array=w354, index (row)=w353, index (col)=1) -> (element=w349:dbl)
                            n1295 = Index Array(array=w354, index (row)=w353, index (col)=0) -> (element=w350:dbl)
                            n1296 = Index Array(array=w366, index=w353) -> (element=w364:T3)
                            n1297 = Unbundle By Name(w364) -> ("Position.x"=w371:dbl, "Position.y"=w369:dbl)
                            n1298 = Multiply(x=w350, y=w356) -> (x*y=w370:dbl)
                            n1299 = Multiply(x=w349, y=w356) -> (x*y=w365:dbl)
                            "probe" <- w365
                            n1300 = Subtract(x=w371, y=w370) -> (x-y=w368:dbl)
                            n1301 = Subtract(x=w369, y=w365) -> (x-y=w367:dbl)
                            n1302 = Bundle By Name(cluster=w364, "Position.x"=w368, "Position.y"=w367) -> (w359:T3)
                            n1303 = local read "Sequence Storer"() -> (w372:T3[][])
                            n1304 = local read "Numeric"() -> (w358:dbl)
                            n1305 = Add(x="Start at Which Frame?", y=w356) -> (x+y=w355:dbl)
                            n1306 = Replace Array Subset(array=w372, new element=w359, index (row)=w355, index (col)=w358) -> (w363:T3[][])
                            n1307 = Array Size(array=w363) -> (size(s)=w362:i32[])
                            n1308 = local write "Sequence Storer"(w363) -> ()
                            n1309 = Index Array(array=w362, index=0) -> (element=w360:i32)
                            n1310 = local write "Sequence Instances"(w360) -> ()
                          }
                        }
                      }
                    }
                    frame #1 {
                      w374 = FALSE
                      n1311 = Tick Count (ms)() -> (millisecond timer value=→"Stop":u32)
                      n1312 = local write "Play Pressed"(w374) -> ()
                      "Insert End" <- w374
                    }
                  }
                }
              }
              "Numeric" <- w301
            }
            frame #2 {
              n1313 = local write "Insert"(FALSE) -> ()
            }
          }
        }
      }
    }
    n1314 = And(x=w88, y=w92) -> (x .and. y?=w93:bool)
    n1315 = case shown="True" w93 {
      frame False {
      }
      frame True {
        n1316 = local read "# of Spots"() -> (w620:dbl)
        n1317 = for {
          N: w620 -> [_]
          i -> [w622]
          stop <- w621 stop-if-true
          n1318 = local read "Selection/Group"() -> (w624:T9[])
          n1319 = Index Array(array=w624, index=w622) -> (element=w623:T9)
          n1320 = Unbundle By Name(w623) -> ("Selected"=w621:bool)
          n1321 = case shown="True" w621 {
            tunnel: w622 -> [_ w626]
            frame False {
            }
            frame True {
              n1322 = local write "Current Spot #"(w626) -> ()
              "Induce check" <- TRUE
            }
          }
        }
      }
    }
    n1323 = local read "spots selected"() -> (w103:i32)
    n1324 = local read "spots selected 2"() -> (w104:i32)
    n1325 = local read "Prev Current Spot"() -> (w112:dbl)
    n1326 = local read "Current Spot #"() -> (w113:dbl)
    n1327 = Not Equal?(x=w113, y=w112) -> (x != y?=w111:bool)
    n1328 = Greater?(x=w104, y=w103) -> (0:w105:bool)
    n1329 = local read "Induce check"() -> (w94:bool)
    n1330 = Or(x=w111, y=w105) -> (x .or. y?=w96:bool)
    n1331 = Or(x=w96, y=w94) -> (x .or. y?=w95:bool)
    n1332 = case shown="True" w95 {
      frame False {
      }
      frame True {
        n1333 = stacked-sequence {
          frame #0 {
            # "A small 100 ms delay is given to provide enough time for the data to be processed properly."
            n1334 = local read "Null array"() -> (w632:dbl[])
            n1335 = local write "What to Check"(w632) -> ()
            n1336 = local write "ID"(w632) -> ()
            n1337 = local read "Current Spot #"() -> (w634:dbl)
            n1338 = local write "Potential Collisions"(0) -> ()
            n1339 = local read "Spot Checker"() -> (w633:T3[])
            n1340 = Index Array(array=w633, index=w634) -> (element=w635:T3)
            n1341 = Wait (ms)(milliseconds to wait=10) -> ()  [unwired: 1 out]
            n1342 = Unbundle By Name(w635) -> ("Position.x"=w629:dbl, "Position.y"=w630:dbl)
            n1343 = local write "Orig Y SC"(w630) -> ()
            n1344 = local write "Orig X SC"(w629) -> ()
            n1345 = local write "Induce check"(FALSE) -> ()
          }
          frame #1 {
            n1346 = local read "# of Spots"() -> (w636:dbl)
            n1347 = for {
              N: w636 -> [_]
              tunnel: w636 -> [w641]
              i -> [w637]
              n1348 = local read "Selection/Group"() -> (w640:T9[])
              n1349 = Index Array(array=w640, index=w637) -> (element=w639:T9)
              n1350 = Unbundle By Name(w639) -> ("Selected"=w638:bool)
              n1351 = case shown="True" w638 {
                tunnel: w641 -> [_ w643]
                tunnel: w637 -> [_ w642]
                frame False {
                }
                frame True {
                  n1352 = for {
                    N: w643 -> [_]
                    tunnel: w642 -> [w644]
                    i -> [w645]
                    # "If the bubble is not selected, find difference of bubble to bubble\nbeing checked"
                    n1353 = local read "Selection/Group"() -> (w649:T9[])
                    n1354 = Index Array(array=w649, index=w645) -> (element=w648:T9)
                    n1355 = Unbundle By Name(w648) -> ("Selected"=w646:bool)
                    n1356 = Not(x=w646) -> (.not. x?=w647:bool)
                    n1357 = case shown="True" w647 {
                      tunnel: w645 -> [_ w653]
                      tunnel: w644 -> [_ w652]
                      tunnel: w644 -> [_ w651]
                      frame False {
                      }
                      frame True {
                        n1358 = local read "Spot Checker"() -> (w670:T3[])
                        n1359 = Index Array(array=w670, index=w653) -> (element=w671:T3)
                        n1360 = Index Array(array=w670, index=w652) -> (element=w669:T3)
                        n1361 = Unbundle By Name(w669) -> ("Position.x"=w666:dbl, "Position.y"=w662:dbl)
                        n1362 = Unbundle By Name(w671) -> ("Position.x"=w663:dbl, "Position.y"=w659:dbl)
                        n1363 = local read "Area+ Buffer"() -> (w650:dbl)
                        n1364 = Subtract(x=w666, y=w650) -> (x-y=w667:dbl)
                        n1365 = Greater Or Equal?(x=w663, y=w667) -> (x >= y?=w668:bool)
                        n1366 = Add(x=w662, y=w650) -> (x+y=w661:dbl)
                        n1367 = Subtract(x=w662, y=w650) -> (x-y=w660:dbl)
                        n1368 = Add(x=w666, y=w650) -> (x+y=w664:dbl)
                        n1369 = Less Or Equal?(x=w659, y=w661) -> (x <= y?=w658:bool)
                        n1370 = Greater Or Equal?(x=w659, y=w660) -> (x >= y?=w657:bool)
                        n1371 = Less Or Equal?(x=w663, y=w664) -> (x <= y?=w665:bool)
                        n1372 = And(x=w668, y=w665) -> (x .and. y?=w655:bool)
                        n1373 = And(x=w658, y=w657) -> (x .and. y?=w656:bool)
                        n1374 = And(x=w655, y=w656) -> (x .and. y?=w654:bool)
                        n1375 = case shown="True" w654 {
                          tunnel: w653 -> [_ _]
                          tunnel: w653 -> [_ w673]
                          tunnel: w651 -> [_ w672]
                          frame False {
                          }
                          frame True {
                            n1376 = stacked-sequence {
                              tunnel: w673 -> [w674 _]
                              tunnel: w672 -> [w675 _]
                              frame #0 {
                                n1377 = local read "Potential Collisions"() -> (w678:dbl)
                                n1378 = local read "What to Check"() -> (w679:dbl[])
                                n1379 = Insert Into Array(array=w679, index=w678, new element=w674) -> (w680:dbl[])
                                n1380 = local read "ID"() -> (w677:dbl[])
                                n1381 = local write "What to Check"(w680) -> ()
                                n1382 = Insert Into Array(array=w677, index=w678, new element=w675) -> (w676:dbl[])
                                n1383 = local write "ID"(w676) -> ()
                              }
                              frame #1 {
                                n1384 = local read "Potential Collisions"() -> (w683:dbl)
                                n1385 = Add(x=w683, y=1) -> (x+y=w681:dbl)
                                n1386 = local write "Potential Collisions"(w681) -> ()
                              }
                            }
                          }
                        }
                      }
                    }
                  }
                }
              }
            }
          }
          frame #2 {
            n1387 = local read "Current Spot #"() -> (w684:dbl)
            n1388 = local write "Prev Current Spot"(w684) -> ()
          }
        }
      }
    }
    n1389 = local read "Buffer Zone"() -> (w109:dbl)
    n1390 = Multiply(x=w109, y=2) -> (x*y=w110:dbl)
    n1391 = Add(x="Area to check", y=w110) -> (x+y=→"Area+ Buffer":dbl)
    n1392 = feedback #11() -> (w82:dbl)  [unwired: 1 in]
    n1393 = Equal?(x=w82, y=10000) -> (x = y?=w83:bool)
    n1394 = call "Elapsed Time"("Reset"=w83) -> ("Elapsed Time (s)"=w81:dbl, "Time has Elapsed"=w86:bool)  [unwired: 11 in, 6 out]
    "Elapsed Time" <- w81
    n1395 = feedback-in #11(w81) -> ()
    n1396 = And(x="On", y=w86) -> (x .and. y?=w87:bool)
    n1397 = case shown="True" w87 {
      frame False {
      }
      frame True {
        n1398 = local read "Position"() -> (w619:cluster{"x":dbl, "y":dbl, "z":dbl})
        n1399 = Unbundle By Name(w619) -> ("x"=→"X Pos every 10 sec":dbl)
      }
    }
    n1400 = case shown="True" "OK Button" {
      frame False {
      }
      frame True {
        n1401 = script code="clear all;\nclc;\n\ng = gigecam('169.254.154.83');\n\ng.PixelFormat= 'BayerGR8'\n\nimg = snapshot(g);\n\nimshow(img);"() -> ()  [unwired: 1 in, 1 out]
      }
    }
    n1402 = case shown="True" "O Button" {
      frame False {
      }
      frame True {
        n1403 = script code="%\n    rslt = Hough1_data(img);\n\n    % Frame translation\n    %- omit this as of now \n    \n    % Control method\n    increment = 10; %assuming the diamiter of the agent around 20 pic \n    \n    %- NewLoc = [x,y] whose unit is px\n    %- update new location based on current location obtained by the camera\n    NewLoc(1)= rslt(1);\n    NewLoc(2)= rslt(2);\n    \n    \n    % Update microrobot location with NewLoc\n    % the single robot would move to oblique downword\n    \n    % wait seconds"() -> ("NewLoc"=w615:dbl[])  [unwired: 1 in, 1 out]
        n1404 = Index Array(array=w615, index=1) -> (element=→"Y":dbl)
        n1405 = Index Array(array=w615, index=0) -> (element=→"X":dbl)
      }
    }
  }
  n1406 = flat-sequence {
    tunnel: w6 -> [w2150]
    tunnel: w5 -> [w2149]
    tunnel: [w2148] -> w3
    frame #0 {
      n1407 = disable-structure shown="\"White Image (stub)\"" {
        disable-tunnel: w2150 -> [_ _ _ _ _ _]
        disable-tunnel: w2149 -> [_ _ w2208 _ _ _]
        disable-tunnel: [_ _ w2207 _ _ _] -> w2148
        frame condition #0 {
          w2152 = u32 10 ("Number of buffers")
          (unwired) FALSE ("background subtraction")
          # "This subdiagram uses the IMAQ drivers, with a pre-allocated ringbuffer for images.  This is the code I use with my Mikrotron MC1362-CL"
          n1408 = call <vilib>:"IMAQ Init.vi"("Interface Name"="img0") -> ("IMAQ Session Out"=w2159:refnum<k11>)  [unwired: 9 in, 1 out]
          n1409 = call <vilib>:"IMAQ Configure List.vi"("Region of interest"="Global ROI (requires restart)", "Number of buffers"=w2152, "Continuous?"=enum16{"One-Shot", "Continuous"}."Continuous", "IMAQ Session In"=w2159) -> ("error out"=w2153:errorcluster, "IMAQ Session Out"=w2155:refnum<k11>)  [unwired: 6 in]
          n1410 = for {
            N: w2152 -> [_]
            tunnel: 0 ("Channel") -> [w2172]
            shift-right: [w2175] -> w2157
            shift-left: w2153 -> [w2171]
            shift-right: [w2174] -> w2156
            shift-left: w2155 -> [w2173]
            i -> [w2170]
            n1411 = Format Into String(format string="mikrotronbuffer%04d", w2170) -> (resulting string=w2168:string)  [unwired: 2 in, 1 out]
            n1412 = call "IMAQ Create"("Image Name"=w2168) -> ("New Image"=w2167:T11)  [unwired: 4 in, 1 out]
            n1413 = call <vilib>:"IMAQ Configure Buffer.vi"("Channel"=w2172, "error in (no error)"=w2171, "Buffer Number"=w2170, "Image In"=w2167, "IMAQ Session In"=w2173) -> ("error out"=w2175:errorcluster, "IMAQ Session Out"=w2174:refnum<k11>)  [unwired: 5 in]
          }
          n1414 = call <vilib>:"IMAQ Start.vi"("error in (no error)"=w2157, "IMAQ Session In"=w2156) -> ("error out"=w2163:errorcluster, "IMAQ Session Out"=w2164:refnum<k11>)  [unwired: 8 in]
          n1415 = call "IMAQ Create"("Image Name"="Red Tweezers live image") -> ("New Image"=w2165:T11)  [unwired: 3 in, 2 out]
          n1416 = while {
            tunnel: w2164 -> [w2183]
            tunnel: w2163 -> [w2182]
            tunnel: w2165 -> [_]
            tunnel: [w2184] -> w2161
            tunnel: [w2177] -> w2162
            i -> [w2179]
            stop <- w2185 stop-if-true
            n1417 = local read "stop"() -> (w2185:bool)
            n1418 = call <vilib>:"IMAQ Extract Buffer.vi"("error in (no error)"=w2182, "Buffer to extract"=w2179, "IMAQ Session In"=w2183) -> ("error out"=w2177:errorcluster, "Image Out"=w2176:T11, "IMAQ Session Out"=w2184:refnum<k11>)  [unwired: 3 in, 3 out]
            n1419 = call "imageQ_camera_hook.vi"("Image"=w2176) -> ()  [unwired: 11 in]
            n1420 = feedback #12() -> (w2180:T34)  [unwired: 1 in]
            n1421 = call "Smoothed Frame Rate.vi"("Feedback In"=w2180) -> ("Feedback Out"=w2181:T34, "Frame Rate"=w2178:dbl)  [unwired: 1 in, 4 out]
            n1422 = feedback-in #12(w2181) -> ()
            n1423 = global write "red_tweezers_globals_INTERNAL_VOLATILE.vi" "Video Frame Rate"(w2178) -> ()
          }
          n1424 = call <vilib>:"IMAQ Close.vi"("error in (no error)"=w2162, "IMAQ Session In"=w2161) -> ()  [unwired: 9 in, 1 out]
        }
        frame condition #1 {
          (unwired) FALSE ("background subtraction")
          # "This subdiagram acquires using the IMAQdx drivers.  This covers most FireWire and GigE cameras (at least the ones supporting the IIDC or GenICam standards)."
          n1425 = call <vilib>:"IMAQdx Open Camera.vi"("Session In"=T8 "dalsaGenie") -> ("error out"=w2188:errorcluster, "Session Out"=w2187:T8)  [unwired: 9 in]
          n1426 = call <vilib>:"IMAQdx Configure Grab.vi"("error in"=w2188, "Session In"=w2187) -> ("error out"=w2189:errorcluster, "Session Out"=w2190:T8)  [unwired: 8 in]
          n1427 = call "IMAQ Create"("Image Name"="Red Tweezers live image") -> ("New Image"=w2193:T11)  [unwired: 3 in, 2 out]
          n1428 = while {
            tunnel: w2190 -> [w2202]
            tunnel: w2189 -> [w2201]
            tunnel: w2193 -> [w2195]
            tunnel: [w2203] -> w2191
            tunnel: [w2197] -> w2192
            stop <- w2204 stop-if-true
            n1429 = local read "stop"() -> (w2204:bool)
            n1430 = call <vilib>:"IMAQdx Grab.vi"("error in"=w2201, "Image In"=w2195, "Session In"=w2202) -> ("error out"=w2197:errorcluster, "Image Out"=w2196:T11, "Session Out"=w2203:T8)  [unwired: 5 in, 1 out]
            n1431 = call "imageQ_camera_hook.vi"("Image"=w2196) -> ()  [unwired: 11 in]
            n1432 = feedback #13() -> (w2199:T34)  [unwired: 1 in]
            n1433 = call "Smoothed Frame Rate.vi"("Feedback In"=w2199) -> ("Feedback Out"=w2200:T34, "Frame Rate"=w2198:dbl)  [unwired: 1 in, 4 out]
            n1434 = feedback-in #13(w2200) -> ()
            n1435 = global write "red_tweezers_globals_INTERNAL_VOLATILE.vi" "Video Frame Rate"(w2198) -> ()
          }
          n1436 = call <vilib>:"IMAQdx Close Camera.vi"("error in"=w2192, "Session In"=w2191) -> ()  [unwired: 9 in, 1 out]
        }
        frame condition #2 {
          # "This subdiagram acquires using the IMAQdx drivers.  This covers most FireWire and GigE cameras (at least the ones supporting the IIDC or GenICam standards)."
          n1437 = call <vilib>:"IMAQdx Open Camera.vi"("Session In"="Camera") -> ("error out"=w2216:errorcluster, "Session Out"=w2215:T8)  [unwired: 9 in]
          n1438 = call <vilib>:"IMAQdx Configure Grab.vi"("error in"=w2216, "Session In"=w2215) -> ("error out"=w2212:errorcluster, "Session Out"=w2213:T8)  [unwired: 8 in]
          n1439 = call "IMAQ Create"("Image Name"="Red Tweezers live image") -> ("New Image"=w2210:T11)  [unwired: 3 in, 2 out]
          n1440 = call "IMAQdx_get_ROI.vi"("Session In"=w2213) -> ("ROI"=w2209:u32[], "Session Out"=w2211:T8)  [unwired: 8 in]
          n1441 = while {
            shift-right: [w2225] -> w2205
            shift-left: w2212 -> [w2226]
            shift-right: [w2222] -> w2206
            shift-left: w2211 -> [w2223]
            tunnel: w2210 -> [w2221]
            tunnel: w2209 -> [w2220]
            tunnel: w2208 -> [w2219]
            tunnel: [w2218] -> w2207
            stop <- w2232 stop-if-true
            n1442 = event shown="[0] Timeout" {
              selector: _ -> [_ _ _]
              dyn-events: _ -> [_ _ _]
              timeout: 0 -> [_ _ _]
              tunnel: w2226 -> [w2239 w2246 w2261]
              tunnel: [w2238 w2246 w2261] -> w2225
              tunnel: w2223 -> [w2237 w2247 w2262]
              tunnel: [w2236 w2247 w2262] -> w2222
              tunnel: w2221 -> [w2235 _ _]
              tunnel: w2220 -> [w2234 _ _]
              tunnel: w2219 -> [_ w2245 w2260]
              event Timeout {
                w2233 = 0  # timeout in ms
                # "Use a timeout of a few hundred ms if you want to acquire just fast enough to update the image- or a timeout of zero to run the camera at full speed."
                # "This VI sends the image to the loop above for display.\nIt's better to do this than to display here, because it separates the camera loop from the front panel a bit, and increases speed without sacrificing responsiveness of the UI.  Of course, using the event structure removes some of those benefits- but it is possible to write a high-performance camera loop with fast particle tracking, and still use this mechanism to display images without slowing down acquisition."
                # "If we're not dealing with other events, acquire from the camera."
                n1443 = event-data() -> ("Time"=w2244:u32)  [unwired: 1 in]
                n1444 = call <vilib>:"IMAQdx Grab.vi"("error in"=w2239, "Image In"=w2235, "Session In"=w2237) -> ("error out"=w2238:errorcluster, "Image Out"=w2241:T11, "Session Out"=w2236:T8)  [unwired: 5 in, 1 out]
                n1445 = call "IMAQ Clear Overlay"("Image"=w2241) -> ("Image Out"=w2240:T11)  [unwired: 9 in, 1 out]
                n1446 = Multiply(x=w2244, y=u32 1000) -> (x*y=w2242:u32)
                n1447 = call "imageQ_camera_hook.vi"("timeout in ms (0=don't wait if there are no requests)"=w2233, "Timestamp/us"=w2242, "ROI"=w2234, "Image"=w2240) -> ()  [unwired: 8 in]
              }
              event "Draw ROI", "Zoom": Value Change {
                # "This changes the current mouse mode on the image, allowing zooming/drawing of ROI (which can be useful if you want to window down a camera for particle tracking)."
                n1448 = event-data() -> ("CtlRef"=w2252:refnum<vi>)  [unwired: 1 in]
                n1449 = control-ref of="Draw ROI"() -> (w2253:refnum<vi>)
                n1450 = Equal?(x=w2253, y=w2252) -> (x = y?=w2251:bool)
                n1451 = case shown="True" w2251 {
                  tunnel: [w2256 w2259] -> w2250
                  tunnel: [TRUE ("stop") FALSE ("stop")] -> w2248
                  tunnel: [FALSE ("Update Indicators?") TRUE ("Update Indicators?")] -> w2249
                  frame False {
                    w2256 = u32 8 items=["Zoom Tool"=8, "Selection Tool"=0, "Pan Tool"=9, "Point Tool"=1, "Line Tool"=2, "Rectangle Tool"=3, "Rotated Rectangle Tool"=12, "Polyline Tool"=10, "Polygon Tool"=5, "Freehand Tool"=11, "Closed Freehand Tool"=6, "Ellipse Tool"=4, "Annulus Tool"=7] ("Current ROI Tool")
                  }
                  frame True {
                    w2259 = u32 3 items=["Zoom Tool"=8, "Selection Tool"=0, "Pan Tool"=9, "Point Tool"=1, "Line Tool"=2, "Rectangle Tool"=3, "Rotated Rectangle Tool"=12, "Polyline Tool"=10, "Polygon Tool"=5, "Freehand Tool"=11, "Closed Freehand Tool"=6, "Ellipse Tool"=4, "Annulus Tool"=7] ("Current ROI Tool")
                  }
                }
                n1452 = local write "Draw ROI"(w2249) -> ()
                n1453 = local write "Zoom"(w2248) -> ()
                n1454 = property on="Property Node" class="ImageControl"(reference=w2245, "Current ROI Tool"=w2250) -> ()  [unwired: 1 in, 2 out]
              }
              event "Zoom to Fit": Value Change {
                # "The various ROI tools are hidden, so the image control resizes nicely as the Red Tweezers window is resized.  The zoom to fit button/mouse mode buttons return some of this functionality."
                n1455 = event-data() -> ("NewVal"=w2263:bool)  [unwired: 1 in]
                n1456 = property on="Property Node" class="ImageControl"(reference=w2260, "Zoom to Fit Mode"=w2263) -> ()  [unwired: 1 in, 2 out]
              }
            }
            n1457 = feedback #14() -> (w2231:T34)  [unwired: 1 in]
            n1458 = call "Smoothed Frame Rate.vi"("Feedback In"=w2231, "Alpha"=0.05) -> ("Feedback Out"=w2230:T34, "Frame Rate"=w2227:dbl)  [unwired: 4 out]
            n1459 = feedback-in #14(w2230) -> ()
            n1460 = global write "red_tweezers_globals_INTERNAL_VOLATILE.vi" "Video Frame Rate"(w2227) -> ()
            n1461 = local read "stop"() -> (w2228:bool)
            n1462 = Unbundle By Name(w2225) -> ("status"=w2218:bool)
            n1463 = Or(x=w2218, y=w2228) -> (x .or. y?=w2232:bool)
          }
          n1464 = call <vilib>:"IMAQdx Close Camera.vi"("error in"=w2205, "Session In"=w2206) -> ()  [unwired: 9 in, 1 out]
        }
        frame condition #3 (active) {
          w2265 = 0 ("element")
          w2267 = 1920 ("dimension size")
          w2266 = 1080 ("dimension size")
          w2268 = T19 0 items=["Grayscale (U8)", "Grayscale (I16)", "Grayscale (SGL)", "Complex (CSG)", "RGB (U32)", "HSL (U32)", "RGB (U64)", "Grayscale (U16)"] ("Image Type")
          (unwired) FALSE ("background subtraction")
          # "This subdiagram generates a blank white image- useful if you don't have a camera"
          n1465 = Build Array(w2265, w2265, w2267, w2266) -> (w2264:i32[])
          n1466 = Initialize Array(u8 255 ("element"), w2266, w2267) -> (w2269:u8[][])
          n1467 = global write "red_tweezers_globals_INTERNAL.vi" "Global ROI"(w2264) -> ()
          n1468 = call "IMAQ Create"("Image Name"="red tweezers camera stub", "Image Type"=w2268) -> ("New Image"=w2270:T11)  [unwired: 2 in, 2 out]
          n1469 = call "IMAQ ArrayToImage"("Image Pixels (U8)"=w2269, "Image"=w2270) -> ("Image Out"=w2273:T11)  [unwired: 8 in, 1 out]
          n1470 = call "IMAQ Create"("Image Name"="Red Tweezers live image") -> ("New Image"=w2274:T11)  [unwired: 3 in, 2 out]
          n1471 = while {
            tunnel: w2273 -> [w2277]
            tunnel: w2274 -> [_]
            stop <- w2281 stop-if-true
            n1472 = local read "stop"() -> (w2281:bool)
            n1473 = Wait Until Next ms Multiple(millisecond multiple=u32 20) -> ()  [unwired: 1 out]
            n1474 = call "imageQ_camera_hook.vi"("Image"=w2277) -> ()  [unwired: 11 in]
            n1475 = feedback #15() -> (w2279:T34)  [unwired: 1 in]
            n1476 = call "Smoothed Frame Rate.vi"("Feedback In"=w2279) -> ("Feedback Out"=w2280:T34, "Frame Rate"=w2278:dbl)  [unwired: 1 in, 4 out]
            n1477 = feedback-in #15(w2280) -> ()
            n1478 = global write "red_tweezers_globals_INTERNAL_VOLATILE.vi" "Video Frame Rate"(w2278) -> ()
          }
        }
        frame condition #4 {
          # "Use this subdiagram if you have an external camera VI which writes to the image queue (using imageQ_camera_hook.vi)"
        }
        frame condition #5 {
          w2282 = path "C:/Users/Tweezer Cube/Desktop/red_tweezers_1_4_rc0/camera_for_rt136.llb/Particle Tracking.vi"  # Path to camera VI
          # "Use this subdiagram if you have an external camera VI which writes to the image queue (using imageQ_camera_hook.vi).  This is the slightly more sophisticated version, which checks that said external VI is running, and runs it if not."
          n1479 = Open VI Reference(vi path=w2282) -> (vi reference=w2283:refnum<vi>, error out=w2285:errorcluster)  [unwired: 5 in]
          n1480 = property class="VI"(reference=w2283) -> ("Path"=w2284:path)  [unwired: 1 in, 2 out]
          n1481 = global write "red_tweezers_globals_INTERNAL_VOLATILE.vi" "Current Camera VI"(w2284) -> ()
          n1482 = property class="VI"(reference=w2283, error in=w2285) -> (reference out=w2290:refnum<vi>, error out=w2289:errorcluster, "Exec.State"=w2287:T36)
          n1483 = Equal?(x=w2287, y=T36."Idle") -> (x = y?=w2291:bool)
          n1484 = case shown="True" w2291 {
            tunnel: w2290 -> [w2295 w2304]
            tunnel: w2289 -> [w2294 w2301]
            tunnel: [w2293 w2300] -> w2286
            tunnel: w2287 -> [w2297 _]
            frame False {
              n1485 = Close Reference(reference=w2295, error in (no error)=w2294) -> (error out=w2293:errorcluster)
              n1486 = Equal?(x=w2297, y=T36."Bad") -> (x = y?=w2296:bool)
              n1487 = case shown="False" w2296 {
                frame False {
                }
                frame True {
                  n1488 = One Button Dialog(message="The external camera VI is not running and cannot be started- it's probably broken or missing.  Check the static/dynamically loaded VI reference in the bottom loop on the block diagram.") -> ()  [unwired: 1 in, 1 out]
                }
              }
            }
            frame True {
              n1489 = invoke class="VI" method="Run VI"(reference=w2304, error in=w2301, "Wait until done"=FALSE ("Wait Until Done"), "Auto Dispose Ref"=TRUE ("Auto Dispose Reference")) -> (error out=w2300:errorcluster)  [unwired: 1 in, 4 out]
            }
          }
          n1490 = call <vilib>:"Simple Error Handler.vi"("error source (\" \")"="External camera VI (see the bottom loop in the block diagram)" ("error source (\" \")"), "error in (no error)"=w2286) -> ()  [unwired: 3 in, 5 out]
        }
      }
    }
  }
  n1491 = while {
    tunnel: w9 -> [w2322]
    shift-right: [w2321] -> w8
    shift-left: w10 -> [w2323]
    shift-right: [w2318] -> _
    shift-left: _ -> [w2311]
    shift-right: [w2317] -> _
    shift-left: _ -> [w2315]
    shift-right: [w2316] -> _
    shift-left: FALSE ("Saving") -> [w2312]
    stop <- w2320 stop-if-true
    w2309 = u32 50 ("millisecond multiple")
    # "Start/stop saving data, if necessary"
    n1492 = Divide(x=u32 1000, y=w2309) -> (x/y=w2307:dbl)
    n1493 = Wait Until Next ms Multiple(millisecond multiple=w2309) -> ()  [unwired: 1 out]
    n1494 = call "imageQ_dequeue.vi"("timeout in ms (-1)"=2000, "Return queue"=w2323, "Image Dst"=w2322) -> ("Timestamp/us"=w2313:u64, "Return queue out"=w2321:refnum<queue>, "Image Dst Out"=w2324:T11, "timed out?"=w2327:bool, "ROI"=w2306:u64[])  [unwired: 4 in]
    n1495 = Not(x=w2327) -> (.not. x?=w2325:bool)
    n1496 = case shown="True" w2325 {
      tunnel: w2324 -> [_ w2361]
      tunnel: w2315 -> [w2354 w2364]
      tunnel: w2312 -> [_ w2358]
      tunnel: [w2354 w2359] -> w2314
      tunnel: w2313 -> [_ w2362]
      tunnel: w2311 -> [w2355 w2363]
      tunnel: [w2355 w2360] -> w2310
      tunnel: w2306 -> [_ w2357]
      frame False {
      }
      frame True {
        n1497 = global read "red_tweezers_globals_INTERNAL.vi" "Image Overlay (extras from control loop)"() -> (w2372:T21[])
        n1498 = case shown="True" w2358 {
          tunnel: w2364 -> [w2373 w2375]
          tunnel: w2363 -> [w2374 w2381]
          tunnel: w2362 -> [_ w2380]
          tunnel: w2361 -> [_ w2379]
          tunnel: [w2374 w2378] -> w2360
          tunnel: [w2373 w2377] -> w2359
          frame False {
          }
          frame True {
            n1499 = call "save_data_save.vi"("Image"=w2379, "Timestamp"=w2380, "Avi Refnum"=w2375, "Data refnum"=w2381) -> ("error out"=w2376:errorcluster, "Avi Refnum (duplicate)"=w2377:T37, "Data refnum (duplicate)"=w2378:refnum<file>)  [unwired: 5 in]
            n1500 = case shown="Error" w2376 {
              selector: w2376 -> [_ w2383]
              frame No Error {
              }
              frame Error {
                n1501 = call <vilib>:"Clear Errors.vi"("error in (no error)"=w2383) -> ()  [unwired: 5 in, 2 out]
                n1502 = local write "Save Video"(FALSE ("Save")) -> ()
              }
            }
          }
        }
        n1503 = global write "red_tweezers_globals_INTERNAL.vi" "Global ROI"(w2357) -> ()
        n1504 = global read "red_tweezers_globals_INTERNAL_VOLATILE.vi" "Tracked Spot Positions (3D)"() -> (w2365:cluster{"x":dbl, "y":dbl, "Z":dbl}[])
        n1505 = global read "red_tweezers_globals.vi" "Selection/Group"() -> (w2371:T9[])
        n1506 = global read "red_tweezers_globals.vi" "Spots"() -> (w2370:T3[])
        n1507 = call "overlay_positions.vi"("Positions"=w2365, "Image"=w2361) -> ("Image 2"=w2367:T11)  [unwired: 9 in]
        n1508 = call "render_overlay_elements.vi"("Image Overlay (extras from control loop)"=w2372, "Image"=w2367) -> ("Image Out"=w2369:T11)  [unwired: 5 in]
        n1509 = call "grid_and_guides.vi"("Operation"=T16."Render on image", "Image"=w2369) -> ("Image Out"=w2356:T11)  [unwired: 9 in]
        n1510 = call "overlay_spots_on_image.vi"("Selection and Groups"=w2371, "Spots"=w2370, "image"=w2356) -> ("Image"=→"Image":T11)  [unwired: 3 in, 1 out]
      }
    }
    n1511 = global read "red_tweezers_globals_INTERNAL_VOLATILE.vi" "Video Frame Rate"() -> (→"Video Frame Rate":dbl)
    n1512 = case shown="True" "Save Video" {
      tunnel: [w2330 w2345] -> w2318
      tunnel: [w2329 w2339] -> w2317
      tunnel: [FALSE ("Saving") w2344] -> w2316
      tunnel: w2312 -> [w2333 w2343]
      tunnel: w2314 -> [w2331 w2342]
      tunnel: w2310 -> [w2332 w2341]
      tunnel: w2307 -> [_ w2340]
      frame False {
        n1513 = case shown="True" w2333 {
          tunnel: w2332 -> [w2335 w2338]
          tunnel: w2331 -> [w2334 w2337]
          tunnel: [w2335 _] -> w2330
          tunnel: [w2334 _] -> w2329
          frame False {
          }
          frame True {
            n1514 = local write "Save Video"(FALSE ("Save")) -> ()
            n1515 = call "save_data_stop.vi"("Avi Refnum"=w2337, "Data refnum"=w2338) -> ()  [unwired: 10 in]
          }
        }
      }
      frame True {
        n1516 = case shown="False" w2343 {
          selector: w2343 -> [_ w2353]
          tunnel: [w2350 w2351] -> w2345
          tunnel: [w2349 w2352] -> w2339
          tunnel: [w2346 w2353] -> w2344
          tunnel: w2342 -> [_ w2352]
          tunnel: w2341 -> [_ w2351]
          tunnel: w2340 -> [w2348 _]
          frame False {
            n1517 = call "save_data_start.vi"("Save Video"=TRUE, "Frames Per Second"=w2348) -> ("Saving"=w2346:bool, "Avi Refnum"=w2349:T37, "Data Refnum"=w2350:refnum<file>)  [unwired: 3 in]
            n1518 = local write "Save Video"(w2346) -> ()
          }
          frame True {
          }
        }
      }
    }
    n1519 = local read "stop"() -> (w2320:bool)
  }
  n1520 = Release Queue(queue=w8) -> ()  [unwired: 2 in, 3 out]
  n1521 = case shown="True" w3 {
    frame False {
    }
    frame True {
      n1522 = One Button Dialog(message="Warning: there was a camera error.  You may need to restart Red Tweezers.") -> ()  [unwired: 1 in, 1 out]
    }
  }
  n1523 = flat-sequence {
    tunnel: w18 -> [w2389]
    tunnel: w17 -> [_]
    frame #0 {
      # "This autosaves when we stop.  The sequence structures are necessary so that:\n1. loading settings doesn't stop the VI\n2. plugins are still open (and hence saved) when we save settings"
      n1524 = local read "Plugins"() -> (w2392:T5)
      n1525 = global read "red_tweezers_globals_INTERNAL_VOLATILE.vi" "Current Settings File"() -> (w2386:path)
      n1526 = global read "red_tweezers_globals_INTERNAL_VOLATILE.vi" "Save Settings On Exit"() -> (w2385:bool)
      n1527 = flat-sequence {
        tunnel: w2389 -> [w2395]
        tunnel: [w2395] -> w2388
        frame #0 {
          n1528 = local write "stop"(FALSE ("STOP")) -> ()
        }
      }
      n1529 = case shown="True" w2385 {
        tunnel: w2386 -> [_ w2400]
        tunnel: w2388 -> [w2397 w2398]
        tunnel: [w2397 w2398] -> w2387
        frame False {
        }
        frame True {
          n1530 = Path To String(path=w2400) -> (string=w2399:string)
          n1531 = call "settings_save_to_file.vi"("XML File Path"=w2400) -> ()  [unwired: 11 in]
          n1532 = call "settings_filename_to_registry.vi"("Last Used Settings File"=w2399) -> ()  [unwired: 11 in]
        }
      }
      n1533 = flat-sequence {
        tunnel: w2387 -> [w2393]
        tunnel: [w2393] -> _
        frame #0 {
          n1534 = local write "stop"(TRUE ("STOP")) -> ()
        }
      }
      n1535 = control-ref of="Plugin Pnl"() -> (w2390:refnum<vi>)
      n1536 = control-ref of="Plugin:"() -> (w2391:refnum<vi>)
      n1537 = call "plugins_unload.vi"("error in (no error)"=w2387, "Plugins"=w2392, "Sub Panel"=w2390, "Plugin Chooser"=w2391) -> ()  [unwired: 2 in, 2 out]
    }
  }
